vi "TLB Core Programming Tasks 1.00 (incomplete).vi"() -> ()   [LabVIEW 2018]
uses:
  TLB Type Definitions/Intruction Type Definitions.ctl
  TLB Type Definitions/State Type Definitions, for 0.26g versions and later 3.ctl
  <vilib>/Studica/Studica Toolkit/NavX/TypeDefs/Flags/Z900_navX_Flags_OpStatusTypeDef.ctl
  <vilib>/Studica/Studica Toolkit/NavX/TypeDefs/Flags/Z900_navX_Flags_CalibrationStatusTypeDef.ctl
  TLB Type Definitions/Vision cluster.ctl
  TLB Type Definitions/PING CLUSTER.ctl
  TLB Type Definitions/Encoder cluster.ctl
  TLB Type Definitions/Stepper cluster.ctl
  TLB Type Definitions/Yaw Cluster.ctl
  TLB Type Definitions/IR Sensor Type Def.ctl
  TLB Type Definitions/Line Sensor Cluster.ctl
  TLB Type Definitions/Time cluster.ctl
  TLB Type Definitions/Box Colour Detection Cluster (0.26d and above).ctl
  Underlying VI's/FGV's/Box FGV/Box Colour FGV Colours.ctl
  <vilib>/Studica/Studica Toolkit/Background/DIO Channel.ctl
  TLB Type Definitions/Y Stepper cluster.ctl
  TLB Type Definitions/Motor Speed Cluster.ctl
  Labview Training Phase 2/Enum Controls/States for Action Engine.ctl
  Underlying VI's/NavX VI/navX type def.ctl
  <vilib>/Studica/Studica Toolkit/Background/I2C Channel.ctl
  Underlying VI's/I2C Master VI/Arduino_Interfacing.ctl
  Underlying VI's/Motor Control VI with PID/MOTOR CONTROL WITH PID AE DATA MODE TYPE DEF.ctl
  Underlying VI's/Motor Control VI with PID/MOTOR CONTROL WITH PID AE DIRECTION TYPE DEF.ctl
  Experimental VI's/Archived VI's/MOTOR CONTROL NO PID Type Def.ctl
  <vilib>/myRIO/Common/Instrument Driver Framework/myRIO v1.0/AI/typedefs/AI Channels List.ctl
  <vilib>/myRIO/Common/Instrument Driver Framework/myRIO v1.0/AI/typedefs/AI Channels Enum.ctl
  Underlying VI's/Line Sensor AE/Line Sensor AE Type Def.ctl
  Underlying VI's/I2C Master VI/I2C MASTER Type Def.ctl
  Underlying VI's/Elasped Timer/Elapsed timer control.ctl
  Underlying VI's/IMAQ Create Reference AE/IMAQ Reference AE.ctl
  Underlying VI's/FGV's/Box FGV/Box Colour FGV States.ctl
  Underlying VI's/I2C Master VI/I2C_MASTER_WRITE_NEW Type Def.ctl
  Underlying VI's/Modified webcam FGV/Webcam AE.ctl
  <vilib>/userdefined/High Color/IMAQdx.ctl
  <vilib>/Studica/Studica Toolkit/NavX/NavX.lvlib
panel:
  out "Same colour?":bool
  out "Box Colour Detection":T1
  out "Errors detected":bool
  out "Robot ready":bool
  out "Time cluster":T3
  out "Table IR obstruct":bool
  out "Front IR obstruct":bool
  out "Line sensors":T4
  out "IR Sensors":T5
  out "NAVX Values":T6
  out "Stepper position values":T7
  out "Encoder values":T8
  out "Ultrasonic sensors":T9
  out "Selected Task":T10=enum."Start Task 9"
  out "Object recognition mode":enum16{"Ball", "Soap", "Gel", "Pipe", "None"}(ring)
  out "Image Processing Error":errorcluster
  out "Object Detection":T11
  out "Status":T14 {"OP Status" items=["INITIALIZING", "SELFTEST_IN_PROGRESS", "ERROR", "IMU_AUTOCAL_IN_PROGRESS", "NORMAL"]; "Calibration Status" items=["IMU_CAL_STATE_MASK"=3, "IMU_CAL_STATE_INPROGRESS"=0, "IMU_CAL_STATE_ACCUMULATE"=1, "IMU_CAL_STATE_COMPLETE"=2]}
  out "General Errors":errorcluster
  in  "Red LED":bool
  out "Front Ultrasonic obstruct":bool
  out "Speed & distance":T15
  out "Task selection":u8
  out "NavX Readings":T16
  out "Arduino Data":T17
  out "TASK ENABLE":bool
  out "Rising Edge":bool
  in  "Green LED":bool
  out "State Logic":T18=enum."Startup"
  out "elements":T10[](array[typedef])
  in  "STOP TASK":bool
  in  "OK Button":bool
  in  "STOP":bool
  out "Queue Errors":errorcluster
  out "Action Queue Items":i32
  out "State Logic Queue Items":i32
  out "Action Queues items":string[](array[string])=["Hardware reset", "Software reset", ""]
  out "Action State":string
  # "VISION"
  # "TLB FRAMEWORK STATUS"
  # "System Health Status Update"
  # "Test Programme written by Calvin Loke    Dated: 28 Aug 2019\nTest Programme revised by Dr Alex See   Dated 30 Aug 2019\n\nRevision date: 20/03/2020\nProgramme version:   TLB Native Dynamic Events ver 0.19a"
  # "0: Task 1\n1: Task 2\n2: Task 3\n3: Task 4\n4: Task 5\n5: Task 6\n6: Task 7\n7: Task 8 Ball\n8: Task 8 Soap\n9: Task 8 Gel\n10: Task 8 Pipe\n11: Task 9 Blue\n12: Task 9 Black\n13: Task 9 Green\n14: Task 9 Red\n15: Task 9 Yellow"
  # "Ball: Right\nSoap: Left\nGel: Reverse\nPipe: Forward"
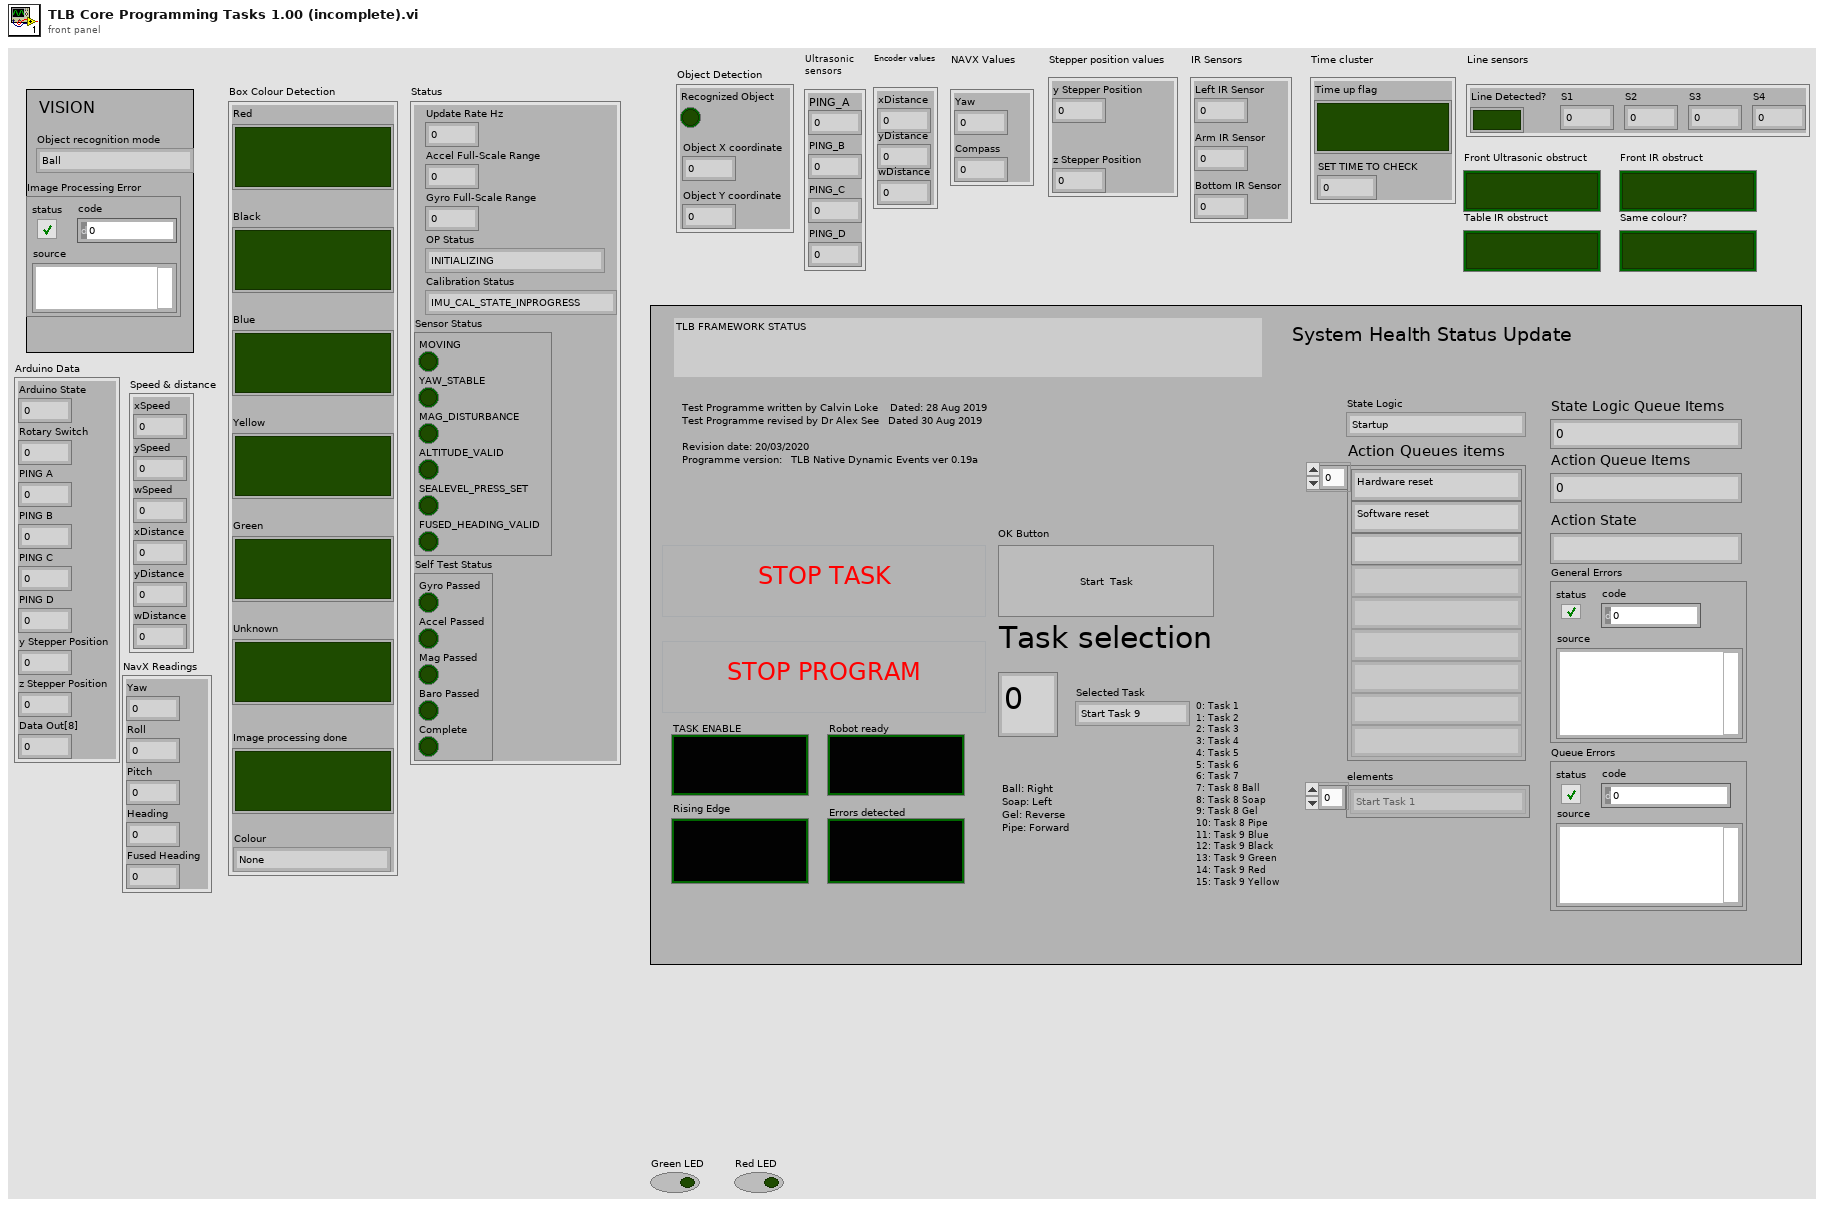
[diagram p1: front panel]
types:
  T1 = typedef "Box Colour Detection Cluster (0.26d and above).ctl" = cluster{"Red":bool, "Black":bool, "Blue":bool, "Yellow":bool, "Green":bool, "Unknown":bool, "Image processing done":bool, "Colour":T2}
  T2 = typedef "Box Colour FGV Colours.ctl" = enum16{"None", "Black", "Blue", "Green", "Red", "Yellow"}
  T3 = typedef "Time cluster.ctl" = cluster{"Time up flag":bool, "SET TIME TO CHECK":dbl}
  T4 = typedef "Line Sensor Cluster.ctl" = cluster{"Line Detected?":bool, "S1":dbl, "S2":dbl, "S3":dbl, "S4":dbl}
  T5 = typedef "IR Sensor Type Def.ctl" = cluster{"Left IR Sensor":dbl, "Arm IR Sensor":dbl, "Bottom IR Sensor":dbl}
  T6 = typedef "Yaw Cluster.ctl" = cluster{"Yaw":dbl, "Compass":dbl}
  T7 = typedef "Stepper cluster.ctl" = cluster{"y Stepper Position":u8, "z Stepper Position":u8}
  T8 = typedef "Encoder cluster.ctl" = cluster{"xDistance":dbl, "yDistance":dbl, "wDistance":dbl}
  T9 = typedef "PING CLUSTER.ctl" = cluster{"PING_A":u8, "PING_B":u8, "PING_C":u8, "PING_D":u8}
  T10 = typedef "Intruction Type Definitions.ctl" = enum16{"None", "Start Task 1", "Start Task 2", "Start Task 3", "Start Task 4", "Start Task 5", "Start Task 6", "Start Task 7", "Start Task 8 - BALL", "Start Task 8 - Gel", "Start Task 8 - Pipe", "Start Task 8 - Soap", "Start Task 9", "Start Task A", "Start Task B", "Exit"}
  T11 = typedef "Vision cluster.ctl" = cluster{"Recognized Object":bool, "Object X coordinate":dbl, "Object Y coordinate":dbl}
  T12 = typedef "NavX.lvlib/Z900_navX_Flags_OpStatusTypeDef.ctl" = u8
  T13 = typedef "NavX.lvlib/Z900_navX_Flags_CalibrationStatusTypeDef.ctl" = u8
  T14 = cluster{"Update Rate Hz":u8, "Accel Full-Scale Range":u8, "Gyro Full-Scale Range":u16, "OP Status":T12, "Calibration Status":T13, "Sensor Status":cluster{"MOVING":bool, "YAW_STABLE":bool, "MAG_DISTURBANCE":bool, "ALTITUDE_VALID":bool, "SEALEVEL_PRESS_SET":bool, "FUSED_HEADING_VALID":bool}, "Self Test Status":cluster{"Gyro Passed":bool, "Accel Passed":bool, "Mag Passed":bool, "Baro Passed":bool, "Complete":bool}}
  T15 = cluster{"xSpeed":dbl, "ySpeed":dbl, "wSpeed":dbl, "xDistance":dbl, "yDistance":dbl, "wDistance":dbl}
  T16 = cluster{"Yaw":dbl, "Roll":dbl, "Pitch":dbl, "Heading":dbl, "Fused Heading":dbl}
  T17 = cluster{"Arduino State":u8, "Rotary Switch":u8, "PING A":u8, "PING B":u8, "PING C":u8, "PING D":u8, "y Stepper Position":u8, "z Stepper Position":u8, "Data Out[8]":u8}
  T18 = typedef "State Type Definitions, for 0.26g versions and later 3.ctl" = enum16{"None", "Startup", "Move to Angle", "True Stop", "Idle", "Shutdown", "Task 1A", "Task 1B", "Task 2:Raise Arm", "Task 2:Sensor Mode", "Task 2:Reverse Mode", "Task 3", "Task 4_A", "Task 4_B", "Task 4_C", "Task 4_D", "Task 5A: RAISING ARM", "Task 5B: STILL WAITING", "Task 5C: GOING DOWN", "Task 5D: GRAB", "Task 5E: GOING UP", "Task 5F: ARM GRAB HEIGHT", "Task 5G: CLOSE CLAW", "Task 5H: RAISE ARM", "Task 6A: RAISE ARM", "Task 6B: CAM BURST", "Task 6C: PROCESS IMAGE", "Task 6D: BALL BUSTER", "Task 6E: STILL WAITING", "Task 6F: CAM BURST 2", "Task 6G: PROCESS IMAGE 2", "Task 6H: SKADI SOAPS", "Task 6I: STILL WAITING 2", "Task 6J: CAM BURST 3", "Task 6K: PROCESS IMAGE 3", "Task 6L: JAM IT IN", "Task 6M: STILL WAITING 3", "Task 6N: CAM BURST 4", "Task 6O: PROCESS IMAGE 4", "Task 6P: PIPE BOMB", "Task 7", "Task 8A: RAISE ARM", "Task 8B: MOVE TO BOX", "Task 8C: CAM BURST", "Task 8D: PROCESS IMAGE", "Task 8E: ROBOT ADJUST", "Task 8F: CAM BURST 2", "Task 8G: PROCESS IMAGE 2", "Task 8H: ARM ADJUST", "Task 8I: ARM GRAB HEIGHT", "Task 8J: CLOSE CLAW", "Task 8K: RAISE MY SWORD", "Task 8I: STILL WAITING", "Task 8L: Return to position", "Task 9A: Raise Arm", "Task 9B: Rotate to Angle", "Task 9C: Detect Box", "Task 9D: MOVE FORWARD", "Task 9E: MOVE LEFT", "Task 9E2: MOVE RIGHT", "Task 9F: SCAN BOX", "Task 9G: MOVE RIGHT", "Task 9H: SCAN BOX 2", "Task 9I: ROTATE 90 CW", "Task 9J: FORWARD", "Task 9K: RAM WALL", "Task 9L: MOVE RIGHT", "Task 9M: SCAN BOX 3", "Task 9N: MOVE RIGHT", "Task 9O: SCAN BOX 4", "Task A1: RAISE ARM", "Task A2: ROTATE TO ANGLE", "Task A3: MOVE TO BL BOX", "Task A4: MOVE FORWARD", "Task A5: ROTATE CW 90"}
  T19 = typedef "Motor Speed Cluster.ctl" = cluster{"ySpeed":dbl, "xSpeed":dbl, "wSpeed":dbl}
  T20 = typedef "Y Stepper cluster.ctl" = cluster{"yStepper desired":u8}
  T21 = typedef "DIO Channel.ctl" = enum16{"Not Connected", "A/DIO1", "A/DIO2", "A/DIO3", "A/DIO4", "A/DIO5", "A/DIO6", "A/DIO7", "A/DIO13", "B/DIO1", "B/DIO2", "B/DIO3", "B/DIO4", "B/DIO5", "B/DIO6", "B/DIO7", "B/DIO13", "C/DIO0", "C/DIO1", "C/DIO2", "C/DIO3", "C/DIO4", "C/DIO5", "C/DIO6", "C/DIO7"}
  T22 = cluster{"DIO Channel":T21, "FPGA VI Reference Out":refnum<k20>}
  T23 = typedef "States for Action Engine.ctl" = enum16{"Initialize", "Write", "Read"}
  T24 = typedef "MOTOR CONTROL WITH PID AE DATA MODE TYPE DEF.ctl" = enum16{"Init AE", "Write to AE", "Read from AE"}
  T25 = typedef "navX type def.ctl" = enum16{"Get i2C reference", "Read Values", "Zero Yaw"}
  T26 = typedef "Arduino_Interfacing.ctl" = enum16{"Initialize", "Write to Arduino", "Read From Arduino"}
  T27 = typedef "I2C Channel.ctl" = enum16{"Not Connected", "A", "B"}
  T28 = cluster{"I2C Ref Out":cluster{"I2C Channel":T27, "FPGA VI Reference Out":refnum<k20>}, "Connected":bool, "Slave Address (7-bit)":u8, "Registry":u8[]}
  T29 = typedef "Box Colour FGV States.ctl" = enum16{"Initialize", "Read", "Write"}
  T30 = typedef "MOTOR CONTROL WITH PID AE DIRECTION TYPE DEF.ctl" = enum16{"y-axis movement", "x-axis movement", "rotation", "stop", "reset encoders"}
  T31 = typedef "Line Sensor AE Type Def.ctl" = enum16{"INIT AE", "READ FROM LINE SENSORS"}
  T32 = typedef "IMAQ Reference AE.ctl" = enum16{"Initialize AE", "Get IMAQ Reference", "Dispose Processing Buffer"}
  T33 = typedef "Elapsed timer control.ctl" = enum16{"Start", "Pause", "Initialize"}
  T34 = typedef "I2C_MASTER_WRITE_NEW Type Def.ctl" = enum16{"Ultrasonic sensors", "Stepper origin", "zStepper 13.3k", "zStepper 13k", "zStepper 12k", "zStepper 11k", "zStepper 10k", "zStepper 9k", "zStepper 8k", "zStepper 7k", "zStepper 6k", "zStepper 5k", "zStepper 4k", "zStepper 3k", "zStepper 2k", "zStepper 1k", "zStepper 900", "zStepper 800", "zStepper 700", "zStepper 600", "zStepper 500", "zStepper 400", "zStepper 300", "zStepper 200", "zStepper 100", "zStepper 0", "yStepper control", "Open Claw", "Close Claw", "Soft Reset"}
  T35 = typedef "Webcam AE.ctl" = enum16{"Initialize Camera", "Open Camera", "Continuous Acquisition", "Close Camera", "Retrieve Image", "Dispose Camera Image Buffer"}
  T36 = typedef "IMAQdx.ctl" = refnum<k21>
  T37 = typedef "MOTOR CONTROL NO PID Type Def.ctl" = enum16{"Init", "Front Back", "Left Right", "Rotate", "Stop", "Latch"}
  T38 = typedef "AI Channels List.ctl" = T39[]
  T39 = typedef "AI Channels Enum.ctl" = enum16{"Not Connected", "AudioIn/Left", "AudioIn/Right", "C/AI0", "C/AI1", "A/AI0", "A/AI1", "A/AI2", "A/AI3", "A/AI4", "A/AI5", "A/AI6", "A/AI7", "B/AI0", "B/AI1", "B/AI2", "B/AI3", "B/AI4", "B/AI5", "B/AI6", "B/AI7", "AI/AI0", "AI/AI1", "AI/AI2", "AI/AI3", "A/AI0 (DIFF)", "A/AI1 (DIFF)", "A/AI2 (DIFF)", "A/AI3 (DIFF)", "B/AI0 (DIFF)", "B/AI1 (DIFF)", "B/AI2 (DIFF)", "B/AI3 (DIFF)"}
  T40 = cluster{"S1":dbl, "S2":dbl, "S3":dbl, "S4":dbl, "Array[4]":dbl, "Array[5]":dbl, "Array[6]":dbl, "Array[7]":dbl, "Array[8]":dbl}
  T41 = typedef "I2C MASTER Type Def.ctl" = enum16{"Last State", "Mode 0", "Mode 1", "Mode 2", "Mode 3", "Mode 4", "Mode 5", "Mode 6", "Mode 7", "Mode 8", "Mode 9", "Mode 10"}
  T42 = typedef "IMAQ Image.ctl" = refnum<image>
  T43 = cluster{"Number of Matches":i32, "Object detected?":bool}
  T44 = cluster{"Red":bool, "Black":bool, "Blue":bool, "Yellow":bool, "Green":bool, "No recognizable coolour":bool}
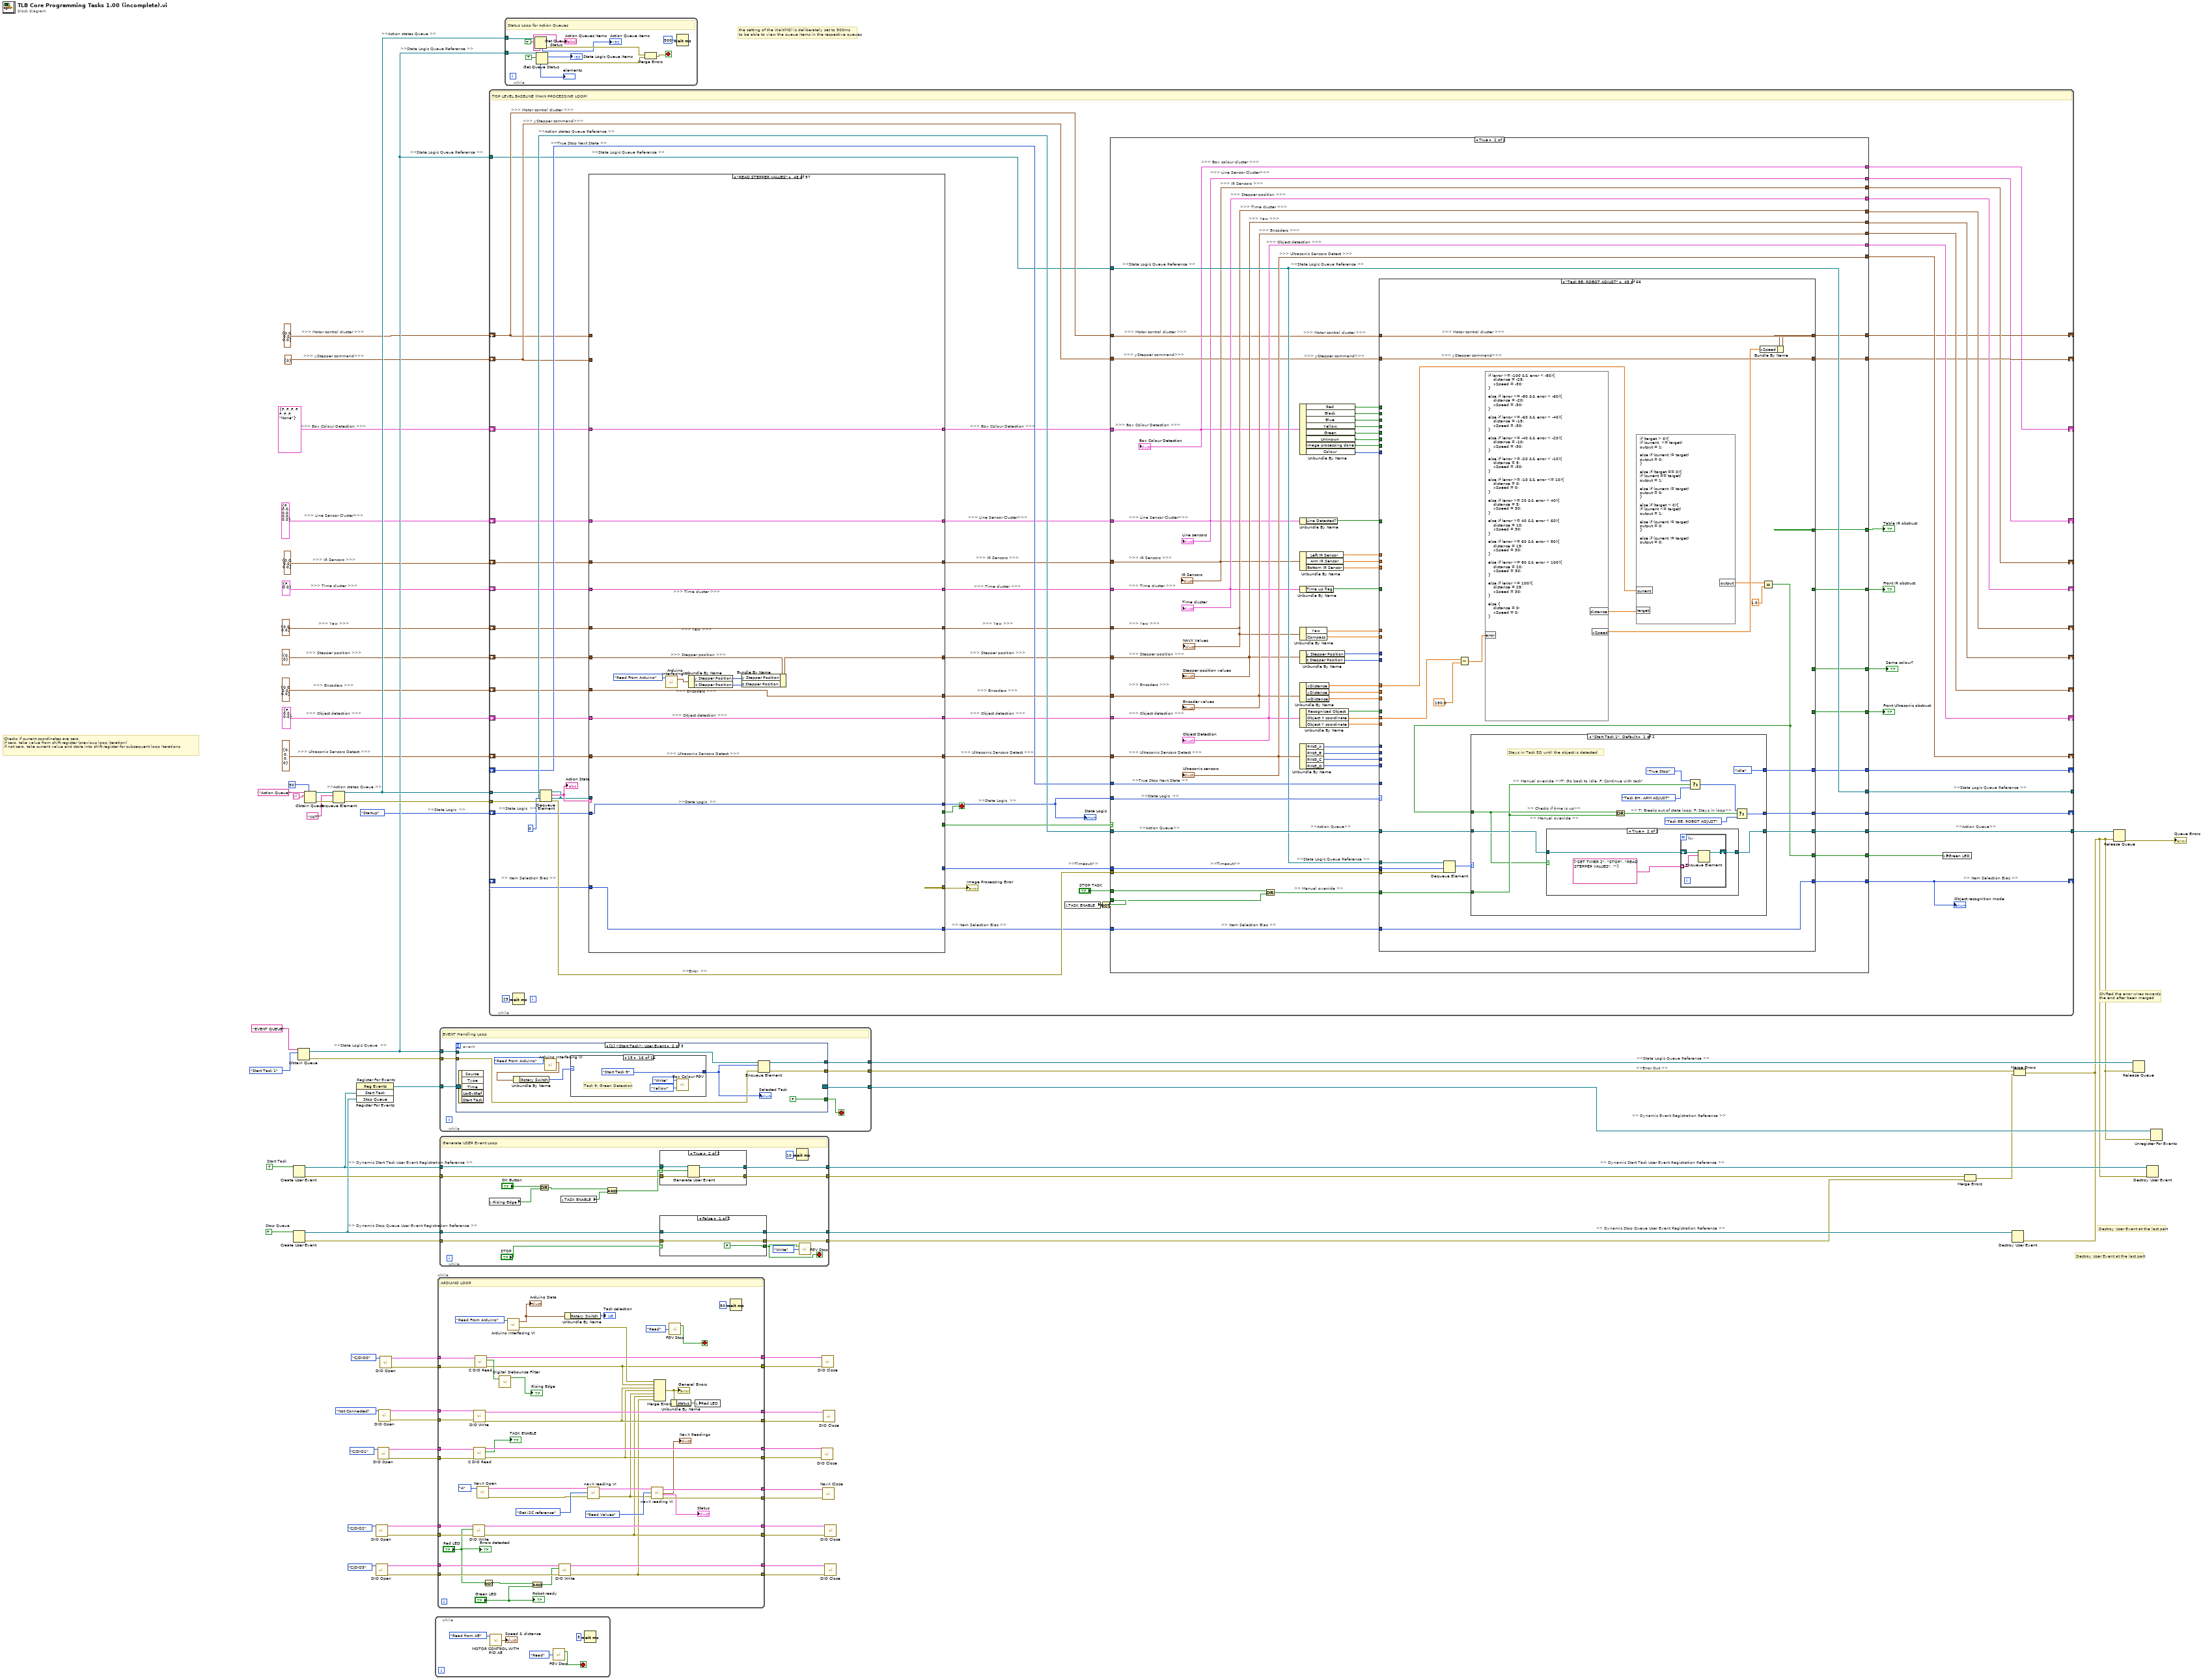
[diagram p0: block diagram]
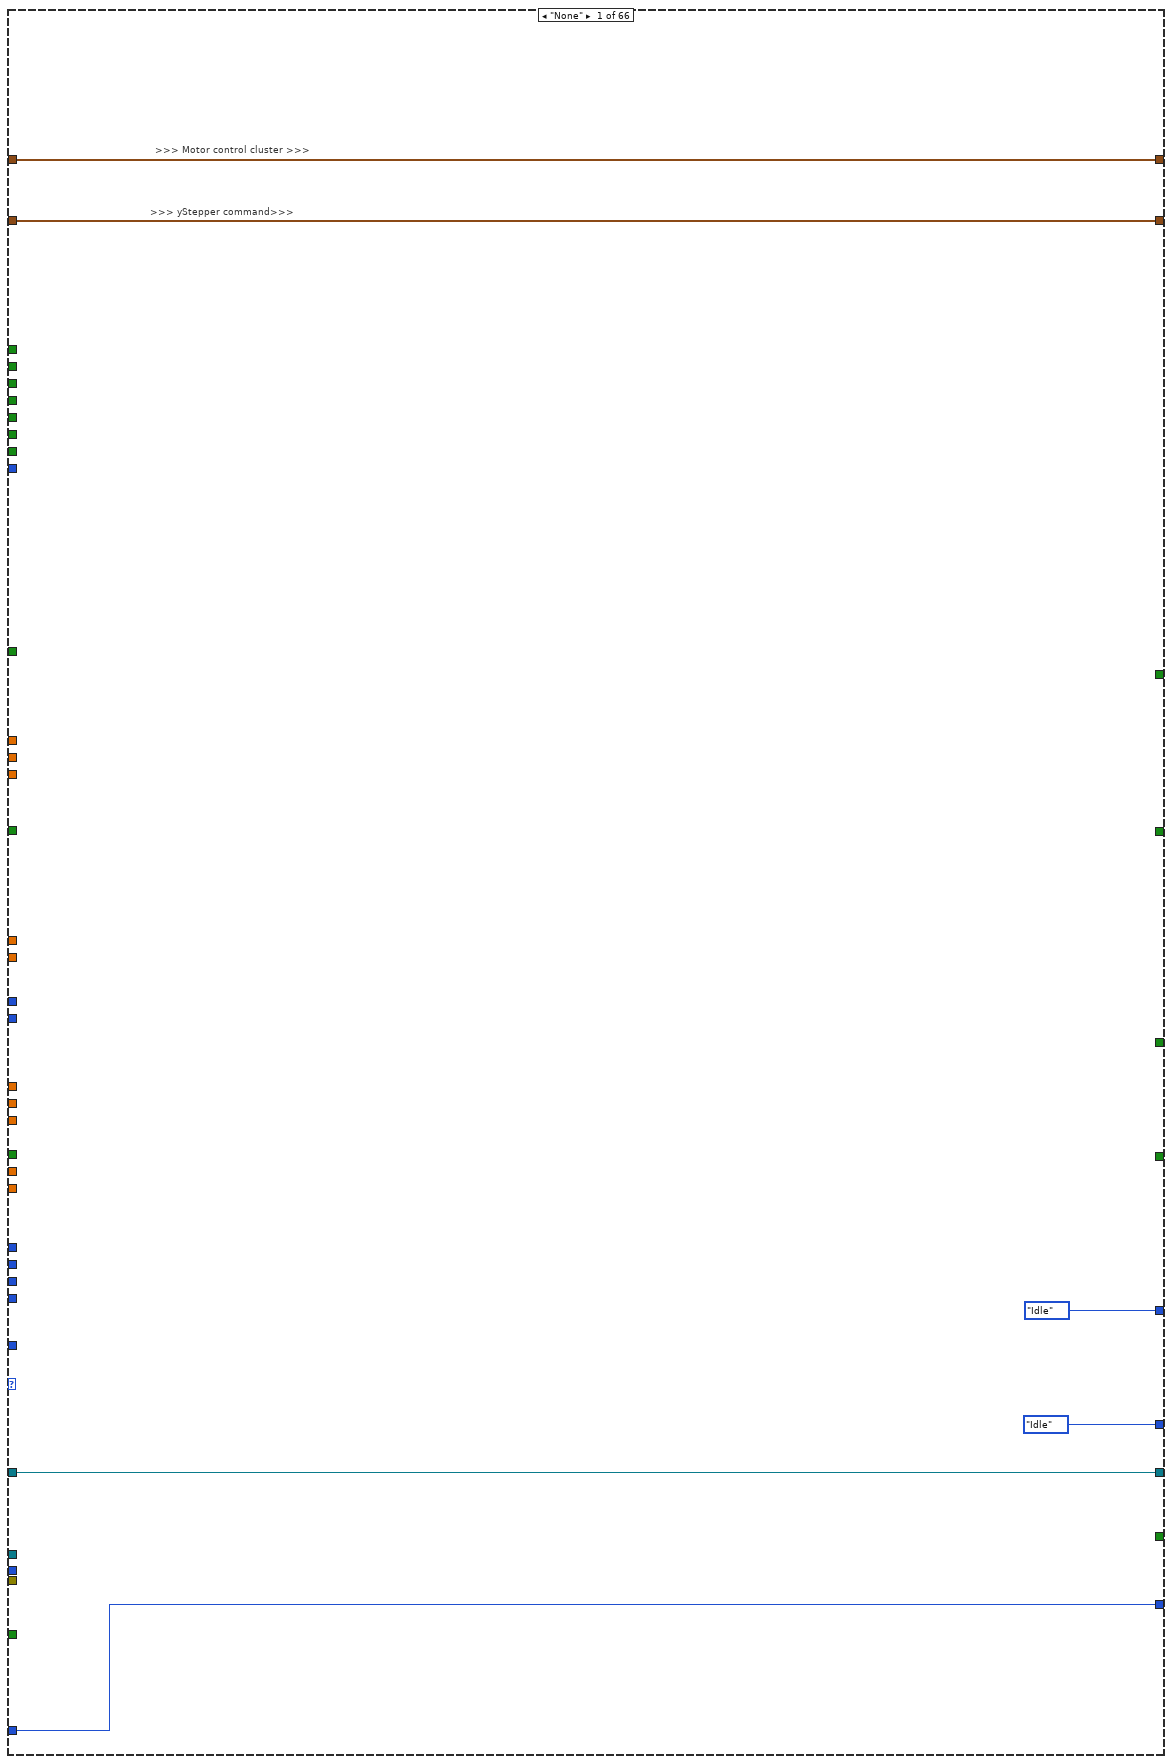
[diagram p3: hidden frame]
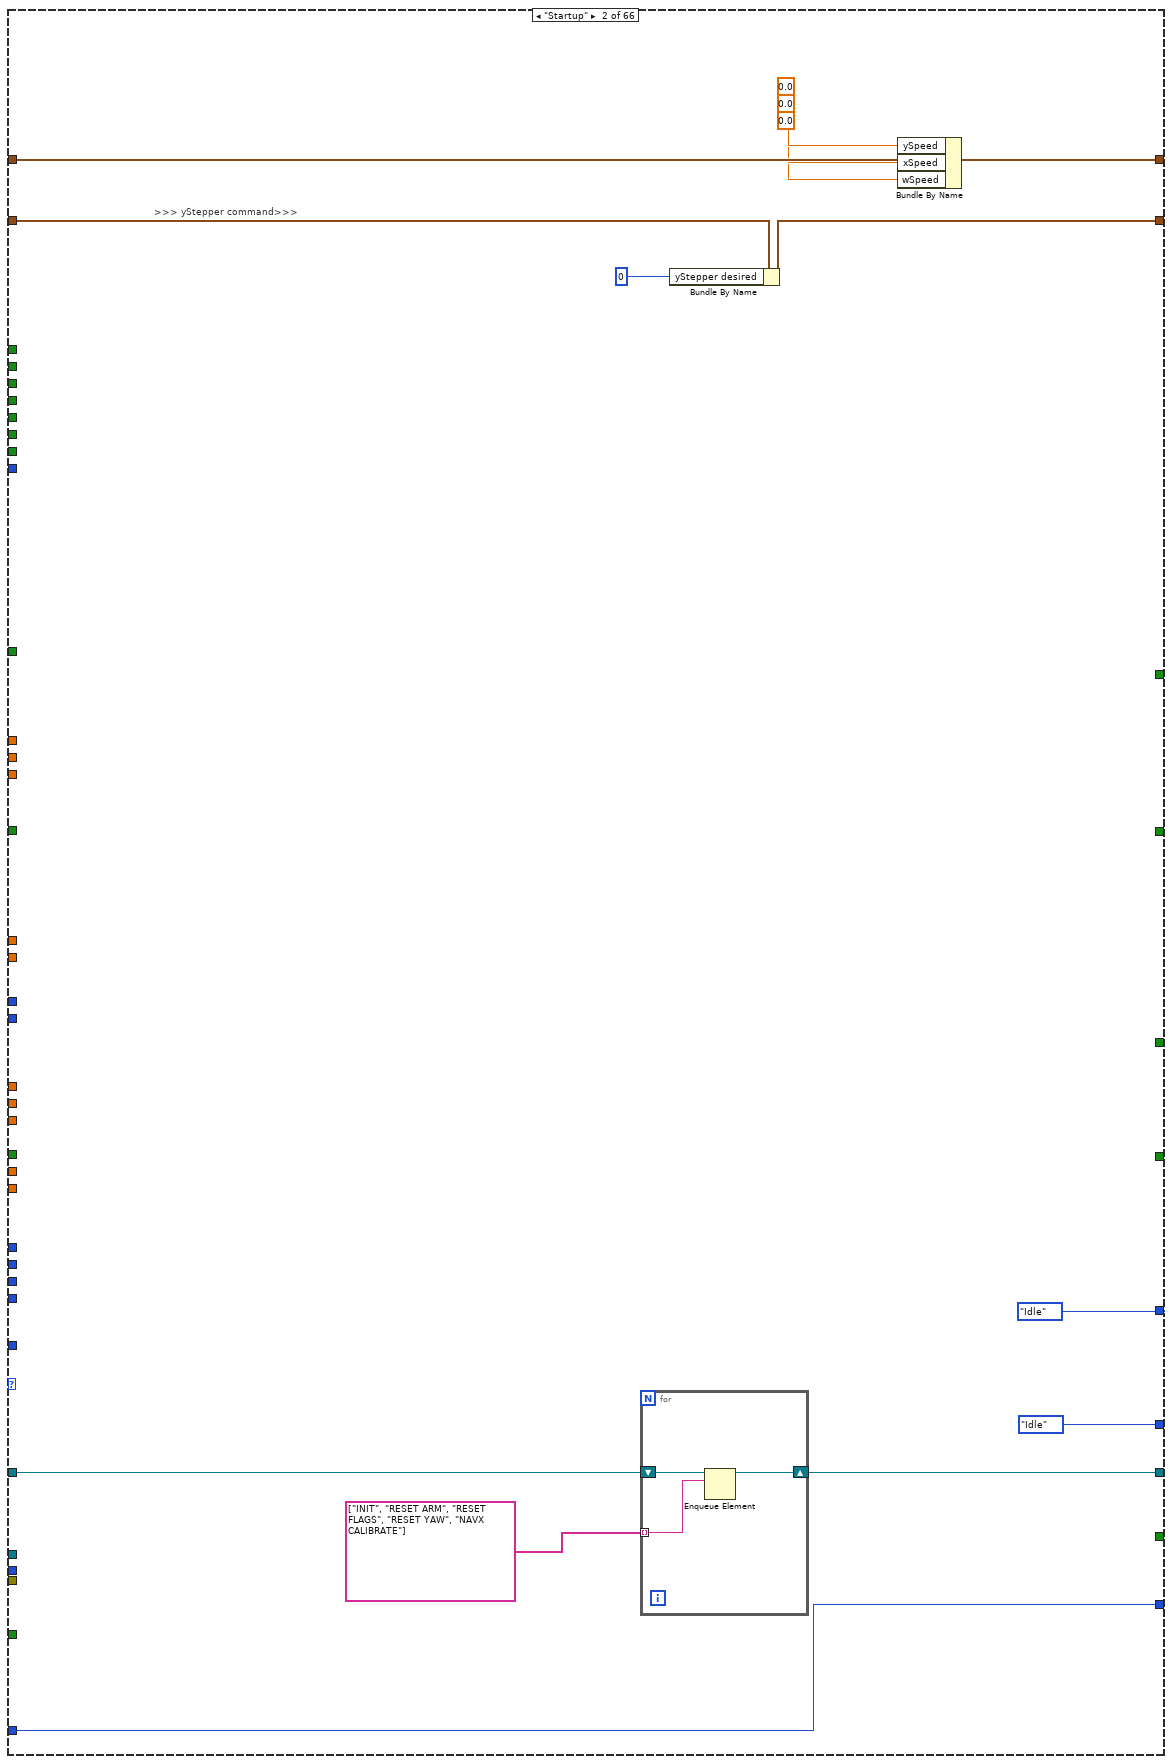
[diagram p4: hidden frame]
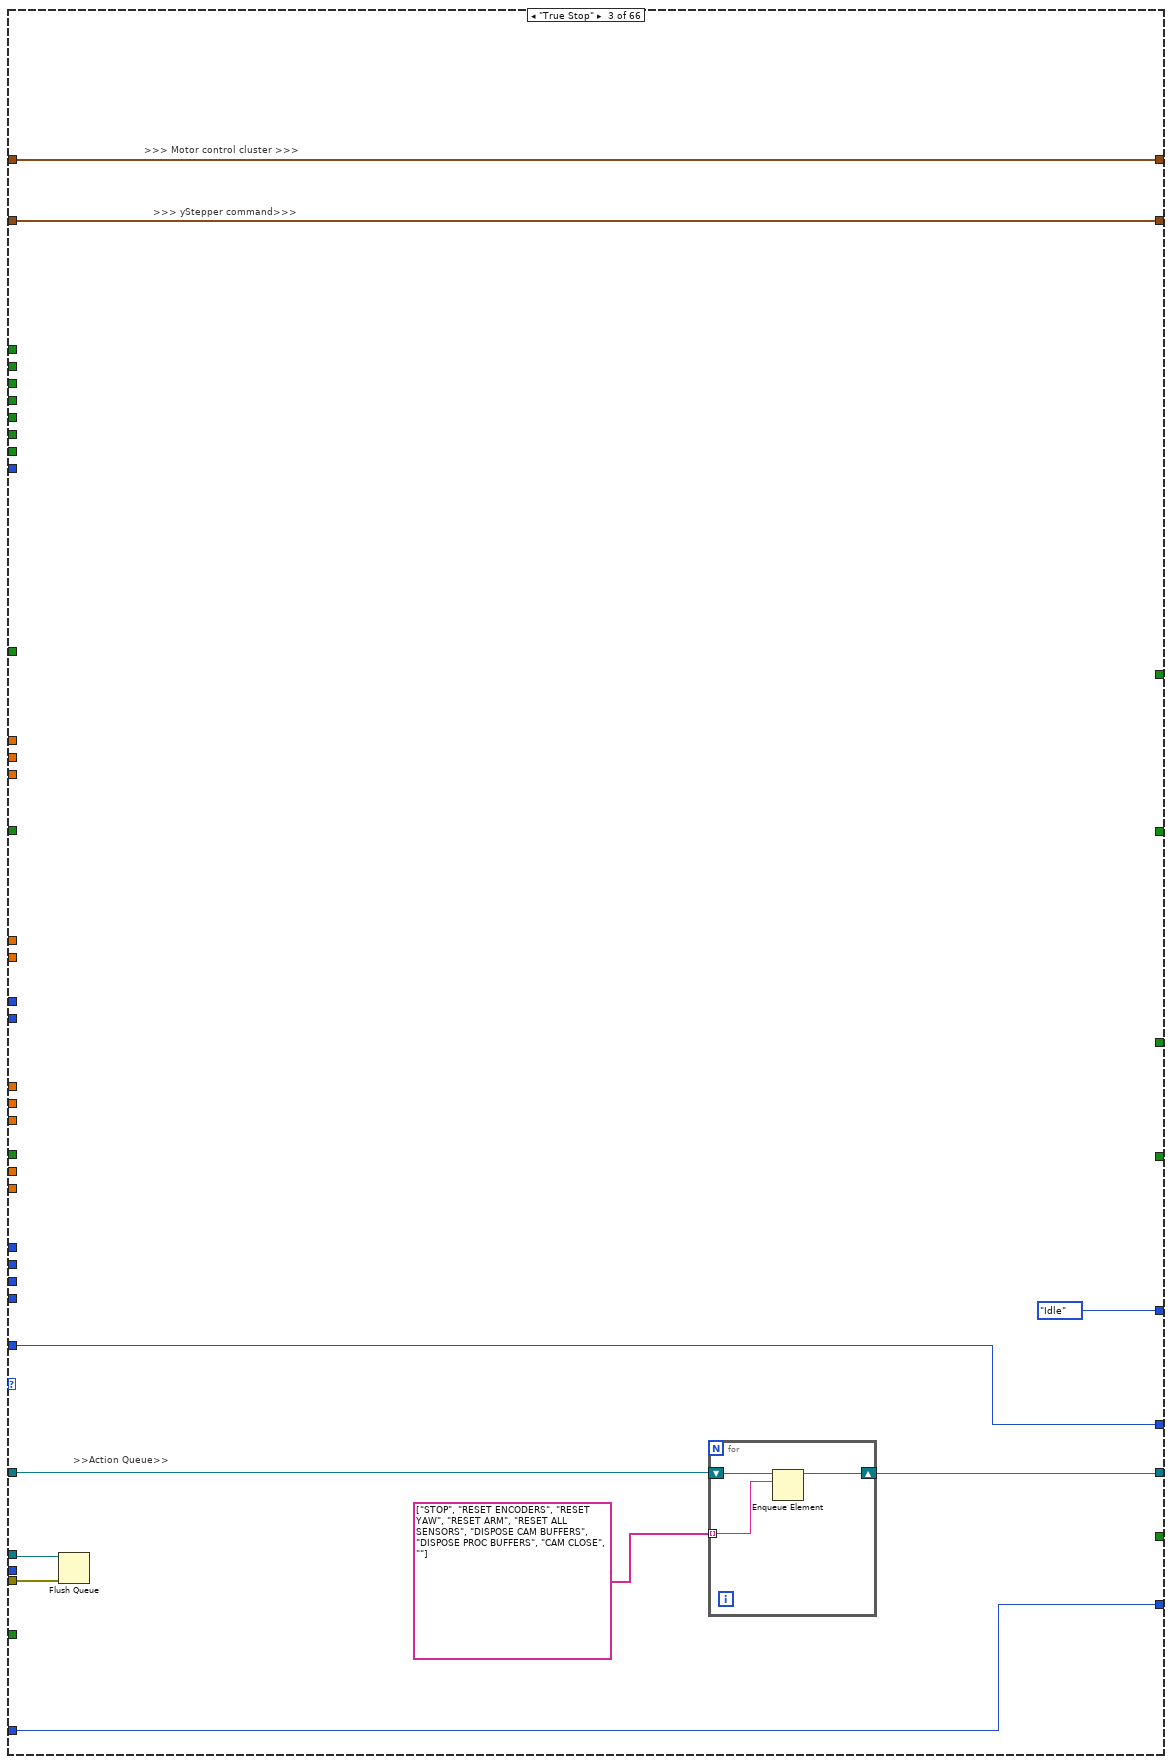
[diagram p5: hidden frame]
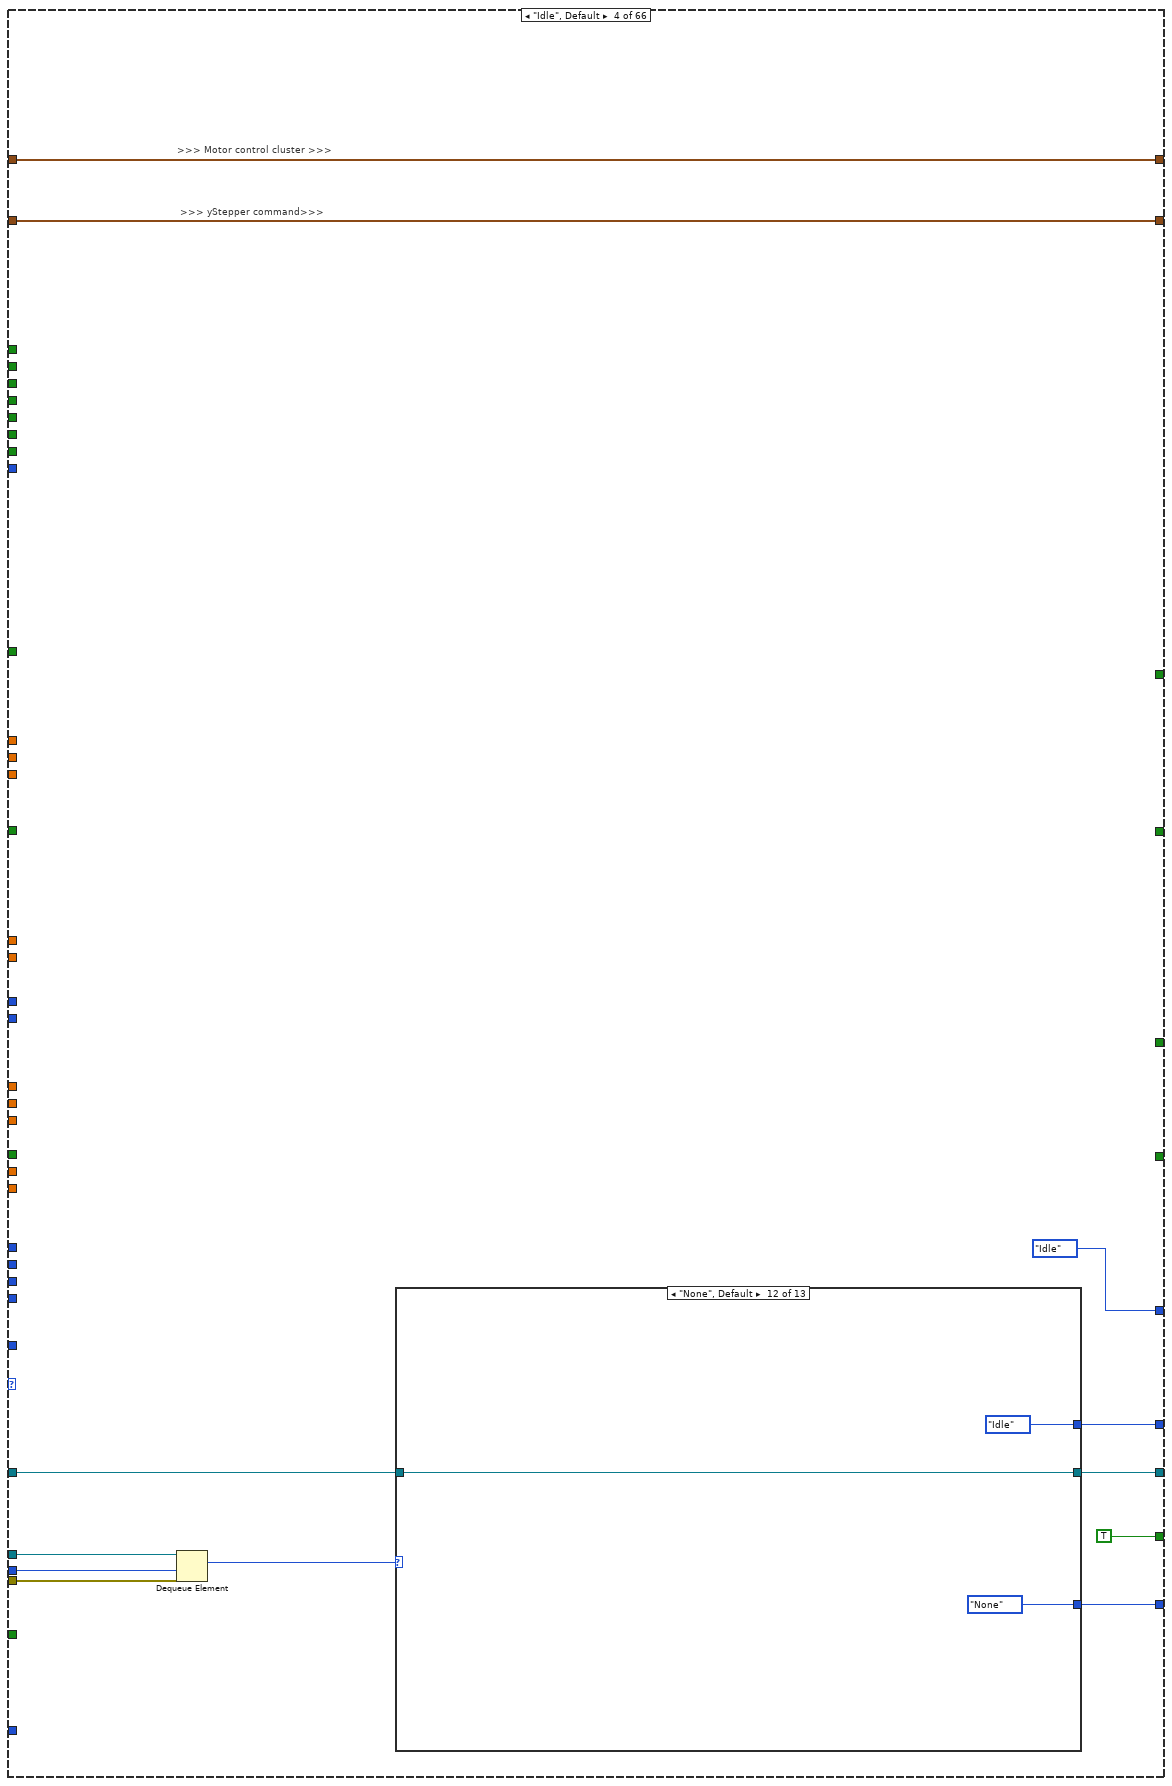
[diagram p6: hidden frame]
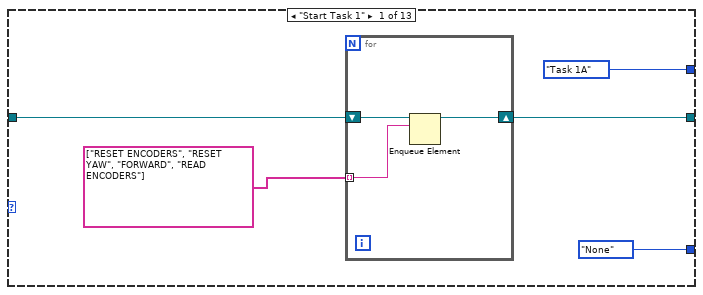
[diagram p7: hidden frame]
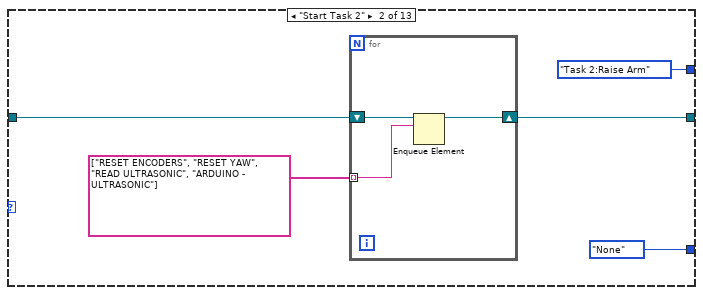
[diagram p8: hidden frame]
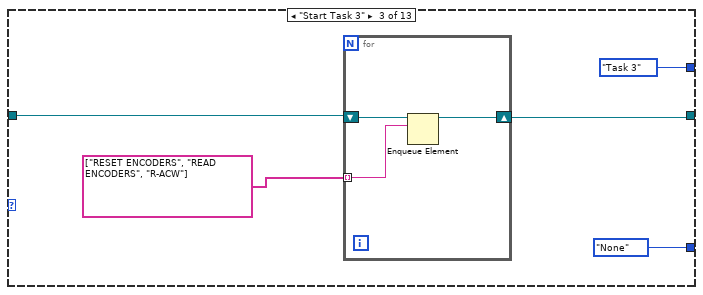
[diagram p9: hidden frame]
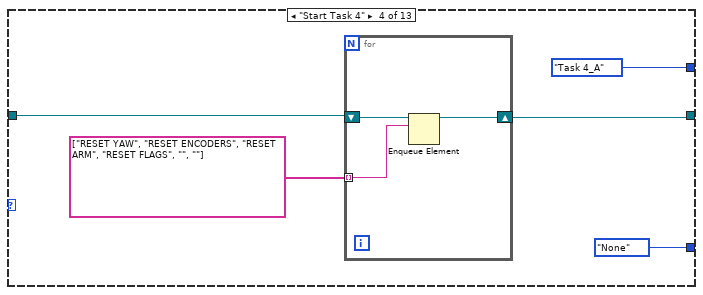
[diagram p10: hidden frame]
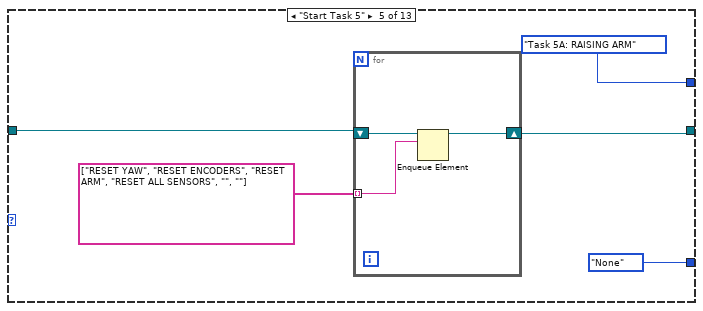
[diagram p11: hidden frame]
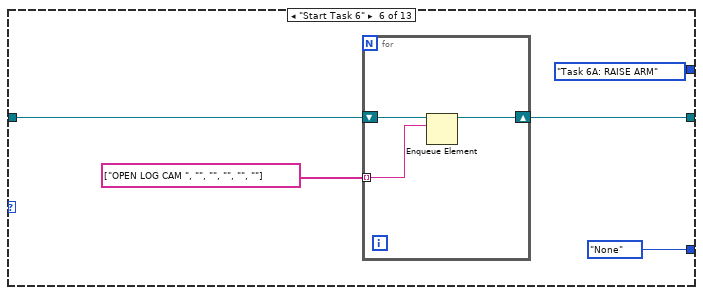
[diagram p12: hidden frame]
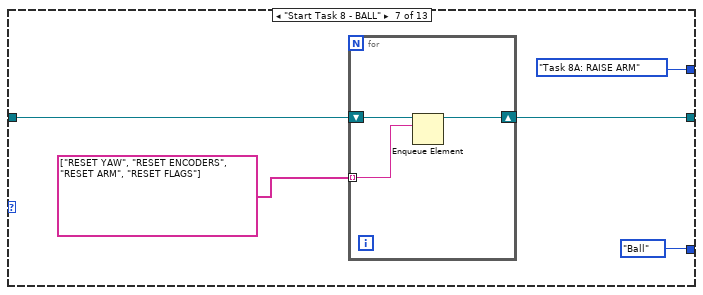
[diagram p13: hidden frame]
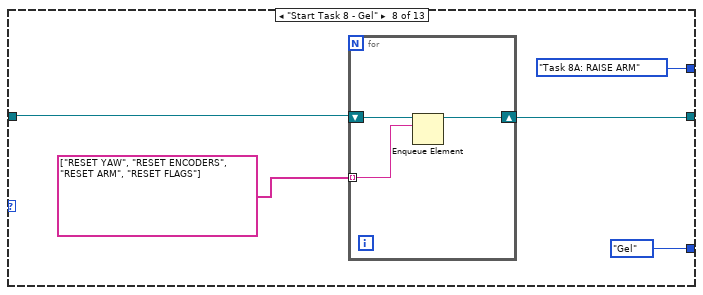
[diagram p14: hidden frame]
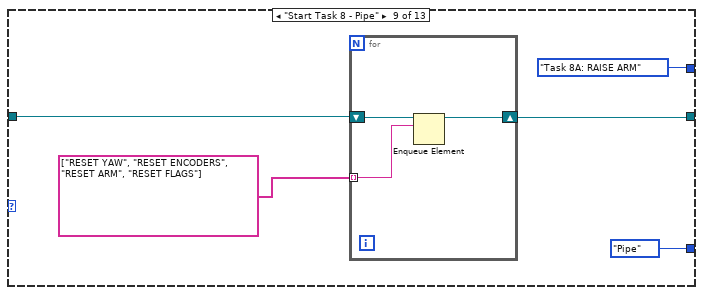
[diagram p15: hidden frame]
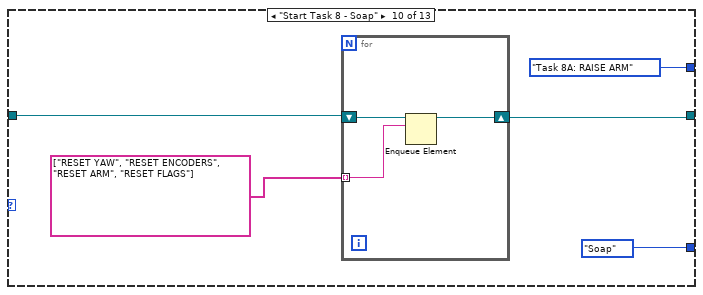
[diagram p16: hidden frame]
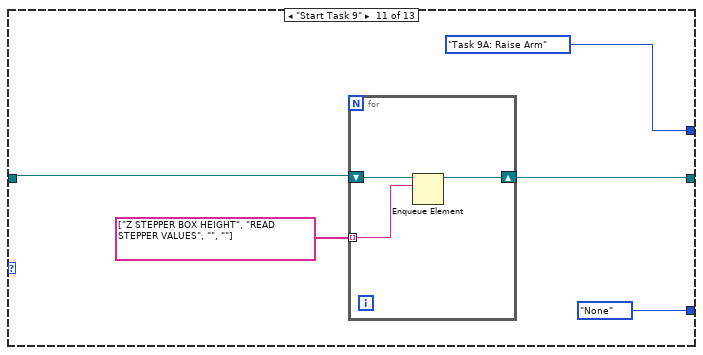
[diagram p17: hidden frame]
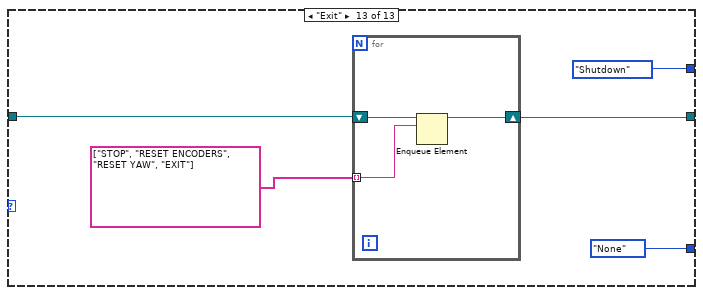
[diagram p18: hidden frame]
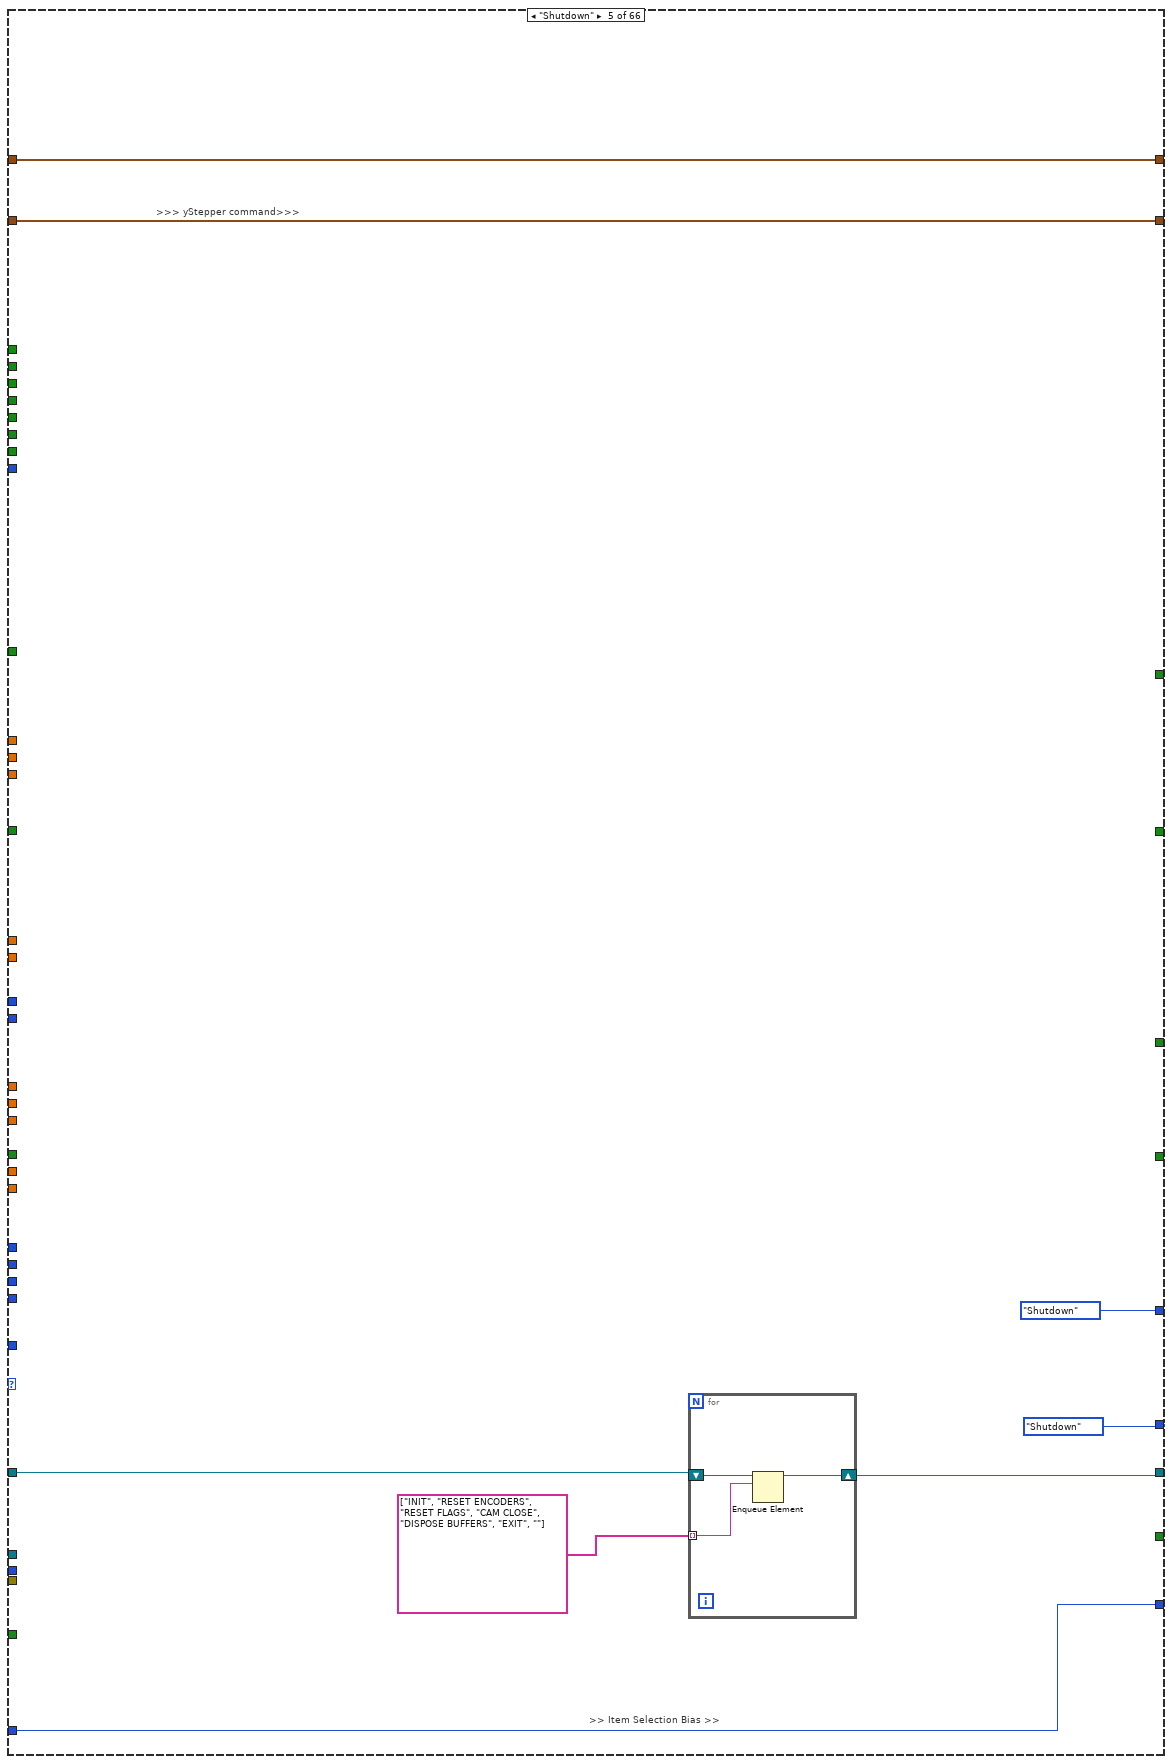
[diagram p19: hidden frame]
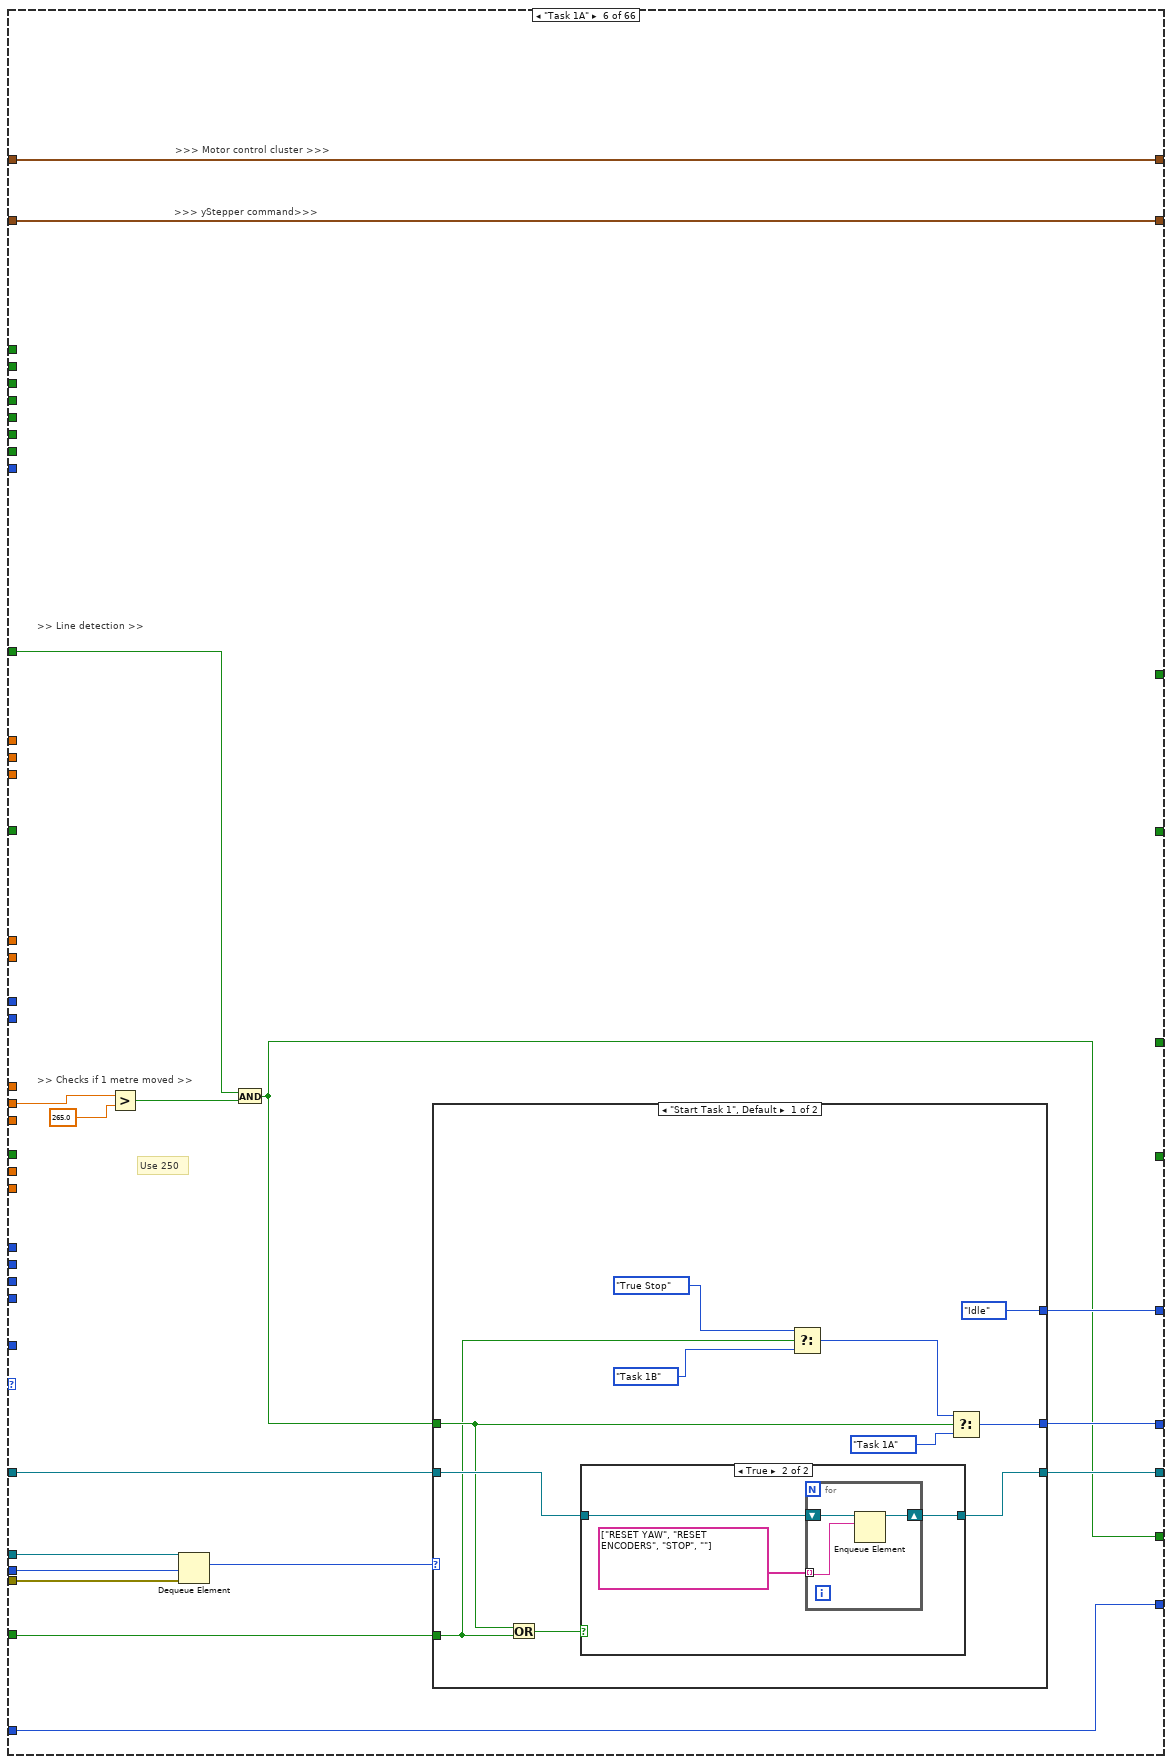
[diagram p20: hidden frame]
diagram:
  w69 = TRUE  # Stop Queue
  w68 = TRUE  # Start Task
  # ">>State Logic Queue Reference >>"
  # ">>Action states Queue >>"
  # ">>> Box Colour Detection >>>"
  # ">>State Logic Queue Reference >>"
  # ">>State Logic  >>"
  # ">>> Line Sensor Cluster>>>"
  # ">>> Motor control cluster >>>"
  # ">>> IR Sensors >>>"
  # "Checks if current coordinates are zero\nif zero, take value from shift register (previous loop iteration)\nif not zero, take current value and store into shift register for subsequent loop iterations"
  # ">>> yStepper command>>>"
  # ">>> Time cluster >>>"
  # ">>> Yaw >>>"
  # ">>> Stepper position >>>"
  # ">>> Encoders >>>"
  # ">>> Object detection >>>"
  # ">>> Ultrasonic Sensors Detect >>>"
  # "the setting of the Wait(MS) is deliberately set to 500ms\nto be able to view the queue items in the respective queues"
  # ">>Error Out >>"
  # ">> Dynamic Stop Queue User Event Registration Reference >>"
  # ">> Dynamic Start Task User Event Registration Reference >>"
  # ">> Dynamic Stop Queue User Event Registration Reference >>"
  # ">> Dynamic Start Task User Event Registration Reference >>"
  # ">> Dynamic Event Registration Reference >>"
  # ">>Action states Queue >>"
  # ">>State Logic Queue  >>"
  # ">>State Logic Queue Reference >>"
  # "Destroy User Event at the last part"
  # "Destroy User Event at the last part"
  # "Shifted the error wires towards\nthe end after been merged"
  n1 = Create User Event(user event datatype=w68) -> (user event=w60:refnum<user-event>, error out=w65:errorcluster)  [unwired: 1 in]
  n2 = Create User Event(user event datatype=w69) -> (user event=w61:refnum<user-event>, error out=w64:errorcluster)  [unwired: 1 in]
  n3 = Obtain Queue(name (unnamed)="EVENT QUEUE", element data type=Intruction_Type_Definitions."Start Task 1" ("Enum")) -> (queue out=w46:refnum<queue>, error out=w52:errorcluster)  [unwired: 3 in, 1 out]
  n4 = Obtain Queue(max queue size (-1, unlimited)=50, name (unnamed)="Action Queue", element data type="") -> (queue out=w55:refnum<queue>, error out=w51:errorcluster)  [unwired: 2 in, 1 out]
  n5 = Enqueue Element(queue=w55, element="INIT", error in (no error)=w51) -> (queue out=w47:refnum<queue>, error out=w50:errorcluster)  [unwired: 1 in, 1 out]
  n6 = register-events "Register For Events"(w60, w61) -> (reference out=w59:refnum<event-registration>)  [unwired: 2 in, 1 out]
  n7 = call <vilib>:"DIO Open.vi"("DIO Channel"=DIO_Channel."C/DIO2") -> ("error out"=w19:errorcluster, "DIO Info Out"=w20:T22)  [unwired: 9 in]
  n8 = call <vilib>:"DIO Open.vi"("DIO Channel"=DIO_Channel."C/DIO3") -> ("error out"=w14:errorcluster, "DIO Info Out"=w15:T22)  [unwired: 9 in]
  n9 = call <vilib>:"DIO Open.vi"("DIO Channel"=DIO_Channel."C/DIO1") -> ("error out"=w24:errorcluster, "DIO Info Out"=w25:T22)  [unwired: 9 in]
  n10 = call <vilib>:"DIO Open.vi"("DIO Channel"=DIO_Channel."Not Connected") -> ("error out"=w29:errorcluster, "DIO Info Out"=w31:T22)  [unwired: 9 in]
  n11 = call <vilib>:"DIO Open.vi"("DIO Channel"=DIO_Channel."C/DIO0") -> ("error out"=w34:errorcluster, "DIO Info Out"=w37:T22)  [unwired: 9 in]
  n12 = while {
    stop <- w71 stop-if-true
    n13 = call "MOTOR CONTROL WITH PID AE.vi"("AE Mode"=MOTOR_CONTROL_WITH_PID_AE_DATA_MODE_TYPE_DEF."Read from AE") -> ("Speed & distance"=→"Speed & distance":T15)  [unwired: 3 in]
    n14 = call "FGV Stop.vi"("Init/Read/Write State"=States_for_Action_Engine."Read") -> ("Output node"=w71:bool)  [unwired: 2 in, 1 out]
    n15 = Wait (ms)(milliseconds to wait=u32 5) -> ()  [unwired: 1 out]
  }
  n16 = while {
    tunnel: w37 -> [w118]
    tunnel: [w117] -> w35
    tunnel: w34 -> [w116]
    tunnel: [w87] -> w33
    tunnel: w31 -> [w113]
    tunnel: [w112] -> w30
    tunnel: w29 -> [w111]
    tunnel: [w86] -> w28
    tunnel: [w110] -> w26
    tunnel: w25 -> [w109]
    tunnel: w24 -> [w108]
    tunnel: [w85] -> w23
    tunnel: w20 -> [w102]
    tunnel: w19 -> [w101]
    tunnel: [w100] -> w18
    tunnel: [w83] -> w17
    tunnel: w15 -> [w99]
    tunnel: w14 -> [w98]
    tunnel: [w97] -> w13
    tunnel: [w82] -> w12
    tunnel: [w94] -> w9
    tunnel: [w93] -> w10
    stop <- w120 stop-if-true
    # "ARDUINO LOOP"
    n17 = call <vilib>:"DIO Write.vi"("error in (no error)"=w101, "Input"="Red LED", "DIO Info In"=w102) -> ("error out"=w83:errorcluster, "DIO Info Out"=w100:T22)  [unwired: 7 in]
    n18 = call <vilib>:"DIO Write.vi"("error in (no error)"=w111, "DIO Info In"=w113) -> ("error out"=w86:errorcluster, "DIO Info Out"=w112:T22)  [unwired: 8 in]
    n19 = call <vilib>:"C DIO Read.vi"("error in (no error)"=w108, "DIO Info In in"=w109) -> ("error out"=w85:errorcluster, "IN"=→"TASK ENABLE":bool, "DIO Info In out"=w110:T22)  [unwired: 7 in]
    n20 = call <vilib>:"C DIO Read.vi"("error in (no error)"=w116, "DIO Info In in"=w118) -> ("error out"=w87:errorcluster, "IN"=w115:bool, "DIO Info In out"=w117:T22)  [unwired: 7 in]
    n21 = call <vilib>:"NavX Open.vi"("I2C Channel"=I2C_Channel."A") -> ("error out"=w104:errorcluster, "NavX Info"=w106:T28)  [unwired: 9 in]
    n22 = Not(x="Red LED") -> (.not. x?=w77:bool)
    n23 = call "Digital Debounce Filter.vi"("Boolean input"=w115) -> ("Rising Edge"=→"Rising Edge":bool)  [unwired: 1 in, 2 out]
    n24 = call "Arduino Interfacing VI.vi"("AE Mode"=Arduino_Interfacing."Read From Arduino") -> ("error out"=w88:errorcluster, "Arduino Data"=w90:T17)  [unwired: 3 in]
    "Arduino Data" <- w90
    n25 = And(x=w77, y="Green LED") -> (x .and. y?=w79:bool)
    n26 = call <vilib>:"DIO Write.vi"("error in (no error)"=w98, "Input"=w79, "DIO Info In"=w99) -> ("error out"=w82:errorcluster, "DIO Info Out"=w97:T22)  [unwired: 7 in]
    n27 = Unbundle By Name(w90) -> ("Rotary Switch"=→"Task selection":u8)
    n28 = call "navX reading VI.vi"("NavX Info In"=w106, "Mode"=navX_type_def."Get i2C reference", "error in (no error)"=w104) -> ("NavX Info Out"=w95:T28, "Error Out"=w84:errorcluster)  [unwired: 2 out]
    n29 = call "navX reading VI.vi"("NavX Info In"=w95, "Mode"=navX_type_def."Read Values", "error in (no error)"=w84) -> ("NavX Info Out"=w94:T28, "NavX Readings"=→"NavX Readings":T16, "Status"=→"Status":T14, "Error Out"=w93:errorcluster)
    n30 = Merge Errors(w88, w87, w86, w85, w84, w83, w82) -> (w80:errorcluster)
    "General Errors" <- w80
    n31 = call "FGV Stop.vi"("Init/Read/Write State"=States_for_Action_Engine."Read") -> ("Output node"=w120:bool)  [unwired: 2 in, 1 out]
    n32 = Unbundle By Name(w80) -> ("status"=w78:bool)
    n33 = local write "Red LED"(w78) -> ()
    n34 = Wait (ms)(milliseconds to wait=u32 50) -> ()  [unwired: 1 out]
    "Robot ready" <- "Green LED"
    "Errors detected" <- "Red LED"
  }
  n35 = while {
    tunnel: w60 -> [w138]
    tunnel: w61 -> [w137]
    tunnel: [w136] -> w67
    tunnel: [w135] -> w66
    tunnel: w65 -> [w134]
    tunnel: [w133] -> w63
    tunnel: w64 -> [w132]
    tunnel: [w131] -> w62
    stop <- w129 stop-if-true
    # "Generate USER Event Loop"
    n36 = local read "Rising Edge"() -> (w126:bool)
    n37 = Or(x="OK Button", y=w126) -> (x .or. y?=w125:bool)
    n38 = local read "TASK ENABLE"() -> (w124:bool)
    n39 = And(x=w125, y=w124) -> (x .and. y?=w123:bool)
    n40 = case shown="True" w123 {
      selector: w123 -> [_ w149]
      tunnel: w138 -> [w148 w153]
      tunnel: [w148 w152] -> w135
      tunnel: w134 -> [w147 w151]
      tunnel: [w147 w150] -> w133
      frame False {
      }
      frame True {
        n41 = Generate User Event(user event=w153, event data cluster=w149, error in=w151) -> (user event out=w152:refnum<user-event>, error out=w150:errorcluster)  [unwired: 1 in]
      }
    }
    n42 = case shown="False" "STOP" {
      selector: "STOP" -> [_ w142]
      tunnel: w137 -> [w141 w146]
      tunnel: [w141 w145] -> w136
      tunnel: w132 -> [w140 w144]
      tunnel: [w140 w143] -> w131
      tunnel: [FALSE w142] -> w129
      frame False {
      }
      frame True {
        n43 = Generate User Event(user event=w146, event data cluster=w142, error in=w144) -> (user event out=w145:refnum<user-event>, error out=w143:errorcluster)  [unwired: 1 in]
      }
    }
    n44 = Wait (ms)(milliseconds to wait=u32 10) -> ()  [unwired: 1 out]
    n45 = call "FGV Stop.vi"("Init/Read/Write State"=States_for_Action_Engine."Write", "Input Node"=w129) -> ()  [unwired: 1 in, 2 out]
  }
  n46 = while {
    tunnel: w59 -> [w160]
    tunnel: [w159] -> w58
    tunnel: w46 -> [w157]
    tunnel: [w156] -> w57
    tunnel: w52 -> [w155]
    tunnel: [w154] -> w49
    stop <- w158 stop-if-true
    # "EVENT Handling Loop"
    n47 = event shown="[1] <Start Task>: User Event" {
      selector: w160 -> [_ _ _]
      dyn-events: [_ _ _] -> w159
      timeout: _ -> [_ _ _]
      tunnel: [FALSE FALSE w207] -> w158
      tunnel: w157 -> [w165 w174 w205]
      tunnel: [w164 w173 w206] -> w156
      tunnel: w155 -> [w163 w172 w204]
      tunnel: [w162 w171 w203] -> w154
      event Timeout {
        n48 = event-data() -> ()  [unwired: 1 in, 3 out]
        n49 = Enqueue Element(queue=w165, element=Intruction_Type_Definitions."Start Task 1" ("Enum"), error in (no error)=w163) -> (queue out=w164:refnum<queue>, error out=w162:errorcluster)  [unwired: 1 in, 1 out]
      }
      event User Event {
        n50 = event-data() -> ()  [unwired: 1 in, 5 out]
        n51 = call "Arduino Interfacing VI.vi"("AE Mode"=Arduino_Interfacing."Read From Arduino") -> ("Arduino Data"=w168:T17)  [unwired: 3 in, 1 out]
        n52 = Unbundle By Name(w168) -> ("Rotary Switch"=w167:u8)
        n53 = case shown="15" w167 {
          tunnel: [Intruction_Type_Definitions."Start Task 1" ("Enum") Intruction_Type_Definitions."Start Task 2" ("Enum") Intruction_Type_Definitions."Start Task 3" ("Enum") Intruction_Type_Definitions."Start Task 4" ("Enum") Intruction_Type_Definitions."Start Task 5" ("Enum") Intruction_Type_Definitions."Start Task 6" ("Enum") Intruction_Type_Definitions."Start Task 7" ("Enum") Intruction_Type_Definitions."Start Task 8 - BALL" ("Enum") Intruction_Type_Definitions."Start Task 8 - Soap" ("Enum") Intruction_Type_Definitions."Start Task 8 - Gel" ("Enum") Intruction_Type_Definitions."Start Task 8 - Pipe" ("Enum") Intruction_Type_Definitions."Start Task 9" ("Enum") Intruction_Type_Definitions."Start Task 9" ("Enum") Intruction_Type_Definitions."Start Task 9" ("Enum") Intruction_Type_Definitions."Start Task 9" ("Enum") Intruction_Type_Definitions."Start Task 9" ("Enum")] -> w170
          frame 0, Default {
          }
          frame 1 {
          }
          frame 2 {
          }
          frame 3 {
          }
          frame 4 {
          }
          frame 5 {
          }
          frame 6 {
          }
          frame 7 {
          }
          frame 8 {
          }
          frame 9 {
          }
          frame 10 {
          }
          frame 11 {
            # "Task 9: Red Detection"
            n54 = call "Box Colour FGV.vi"("Colour to detect"=Box_Colour_FGV_Colours."Blue", "Init/R/W State"=Box_Colour_FGV_States."Write") -> ()  [unwired: 8 in, 2 out]
          }
          frame 12 {
            # "Task 9: Black Detection"
            n55 = call "Box Colour FGV.vi"("Colour to detect"=Box_Colour_FGV_Colours."Black", "Init/R/W State"=Box_Colour_FGV_States."Write") -> ()  [unwired: 8 in, 2 out]
          }
          frame 13 {
            # "Task 9: Blue Detection"
            n56 = call "Box Colour FGV.vi"("Colour to detect"=Box_Colour_FGV_Colours."Green", "Init/R/W State"=Box_Colour_FGV_States."Write") -> ()  [unwired: 8 in, 2 out]
          }
          frame 14 {
            # "Task 9: Yellow Detection"
            n57 = call "Box Colour FGV.vi"("Colour to detect"=Box_Colour_FGV_Colours."Red", "Init/R/W State"=Box_Colour_FGV_States."Write") -> ()  [unwired: 8 in, 2 out]
          }
          frame 15 {
            # "Task 9: Green Detection"
            n58 = call "Box Colour FGV.vi"("Colour to detect"=Box_Colour_FGV_Colours."Yellow", "Init/R/W State"=Box_Colour_FGV_States."Write") -> ()  [unwired: 8 in, 2 out]
          }
        }
        "Selected Task" <- w170
        n59 = Enqueue Element(queue=w174, element=w170, error in (no error)=w172) -> (queue out=w173:refnum<queue>, error out=w171:errorcluster)  [unwired: 1 in, 1 out]
      }
      event User Event {
        n60 = event-data() -> ("Stop Queue"=w207:bool)  [unwired: 1 in, 4 out]
        n61 = Enqueue Element At Opposite End(queue=w205, element=Intruction_Type_Definitions."Exit" ("Enum"), error in (no error)=w204) -> (queue out=w206:refnum<queue>, error out=w203:errorcluster)  [unwired: 1 in, 1 out]
      }
    }
  }
  n62 = while {
    tunnel: w46 -> [w210]
    tunnel: w47 -> [w268]
    tunnel: w50 -> [w266]
    tunnel: [w265] -> _
    tunnel: [w264] -> w40
    shift-right: [w257] -> _
    shift-left: T9 {"PING_A"=0, "PING_B"=0, "PING_C"=0, "PING_D"=0} -> [w259]
    shift-right: [w251] -> _
    shift-left: State_Type_Definitions,_for_0.26g_versions_and_later_3."Startup" ("Enum") -> [w254]
    shift-right: [w247] -> _
    shift-left: T8 {"xDistance"=0.0, "yDistance"=0.0, "wDistance"=0.0} -> [w249]
    shift-right: [w244] -> _
    shift-left: _ -> [w243]
    shift-right: [w240] -> _
    shift-left: T11 {"Recognized Object"=FALSE, "Object X coordinate"=0.0, "Object Y coordinate"=0.0} -> [w242]
    shift-right: [w237] -> _
    shift-left: T7 {"y Stepper Position"=0, "z Stepper Position"=0} -> [w239]
    shift-right: [w234] -> _
    shift-left: T6 {"Yaw"=0.0, "Compass"=0.0} -> [w236]
    shift-right: [w231] -> _
    shift-left: T3 {"Time up flag"=FALSE, "SET TIME TO CHECK"=0.0} -> [w233]
    shift-right: [w229] -> _
    shift-left: T20 {"yStepper desired"=0} -> [w230]
    shift-right: [w225] -> _
    shift-left: T5 {"Left IR Sensor"=0.0, "Arm IR Sensor"=0.0, "Bottom IR Sensor"=0.0} -> [w227]
    shift-right: [w223] -> _
    shift-left: T19 {"ySpeed"=0.0, "xSpeed"=0.0, "wSpeed"=0.0} -> [w224]
    shift-right: [w220] -> _
    shift-left: T4 {"Line Detected?"=FALSE, "S1"=0.0, "S2"=0.0, "S3"=0.0, "S4"=0.0} -> [w222]
    shift-right: [w218] -> _
    shift-left: _ -> [w217]
    shift-right: [w209] -> _
    shift-left: T1 {"Red"=FALSE, "Black"=FALSE, "Blue"=FALSE, "Yellow"=FALSE, "Green"=FALSE, "Unknown"=FALSE, "Image processing done"=FALSE, "Colour"=enum."None"} -> [w212]
    stop <- w256 stop-if-true
    # ">>> Box Colour Detection >>>"
    # ">>State Logic Queue Reference >>"
    # ">>Action Queue>>"
    # ">>State Logic Queue Reference >>"
    # ">>> Line Sensor Cluster>>>"
    # ">>> IR Sensors >>>"
    # ">>> Time cluster >>>"
    # ">>> Object detection >>>"
    # ">>> Yaw >>>"
    # ">>> Ultrasonic Sensors Detect >>>"
    # ">>> Encoders >>>"
    # ">>> Stepper position >>>"
    # ">>State Logic  >>"
    # ">> Item Selection Bias >>"
    # ">> Item Selection Bias >>"
    # ">> Item Selection Bias >>"
    # ">>State Logic  >>"
    # ">>> Motor control cluster >>>"
    # ">>> yStepper command>>>"
    # ">>True Stop Next State >>"
    # ">>Error  >>"
    # ">>Timeout>>"
    # ">>Action states Queue Reference >>"
    # "TOP LEVEL BASELINE (MAIN PROCESSING LOOP)"
    n63 = Wait (ms)(milliseconds to wait=u32 25) -> ()  [unwired: 1 out]
    n64 = Dequeue Element(queue=w268, timeout in ms (-1)=0, error in (no error)=w266) -> (queue out=w260:refnum<queue>, element=w267:string, error out=w261:errorcluster)  [unwired: 1 out]
    "Action State" <- w267
    n65 = case shown="\"READ STEPPER VALUES\"" w267 {
      tunnel: [_ _ _ _ _ _ _ _ _ _ _ _ _ _ _ _ _ _ _ _ 0 w3637 _ _ _ _ _ _ _ _ _ _ _ _ _ _ _ _ _ _ _ _ _ _ _ _ _ _ _ _ _ _ _ _ _ _ _] -> w263
      tunnel: w260 -> [_ _ _ _ _ _ _ _ _ _ _ _ _ _ _ _ _ _ _ _ _ _ _ _ _ _ _ _ _ _ _ _ _ _ _ _ _ _ _ _ _ _ _ _ _ _ _ _ _ _ _ _ _ _ _ _ _]
      tunnel: w259 -> [w3309 w3321 w3336 w3350 w3370 w3385 w3399 w3413 w3429 w3444 w3458 w3468 w3486 w3503 w3518 w3533 w3557 w3567 w3598 w3611 w3625 w3638 w3650 w3663 w3683 w3718 w3755 w3769 w3780 w3792 w3805 w3820 w3836 w3848 w3860 w3880 w3903 w3914 w3930 w3961 w3971 w3984 w3997 w4010 w4020 w4038 w4048 w4067 w4076 w4092 w4108 w4124 w4140 w4156 w4170 w4185 w4205]
      tunnel: [w3309 w3321 w3336 w3350 w3370 w3385 w3399 w3413 w3429 w3444 w3458 w3468 w3486 w3504 w3518 w3533 w3557 w3567 w3599 w3611 w3625 w3638 w3650 w3663 w3683 w3717 w3754 w3769 w3780 w3792 w3805 w3820 w3836 w3848 w3860 w3880 w3903 w3914 w3930 w3961 w3971 w3984 w3997 w4010 w4020 w4038 w4048 w4067 w4076 w4092 w4108 w4124 w4140 w4156 w4170 w4185 w4205] -> w258
      tunnel: [TRUE TRUE _ _ _ _ _ _ _ _ _ _ _ _ _ _ _ _ _ _ _ _ _ _ _ _ _ _ _ _ _ _ _ _ _ _ _ _ _ _ _ _ _ _ _ _ _ _ _ _ _ _ _ _ _ _ _] -> w256
      tunnel: w254 -> [w3307 w3319 w3335 w3349 w3369 w3384 w3398 w3412 w3428 w3443 w3457 w3467 w3485 w3502 w3517 w3531 w3550 w3566 w3597 w3610 w3622 w3635 w3649 w3662 w3682 w3716 w3753 w3768 w3779 w3791 w3797 w3819 w3835 w3847 w3859 w3879 w3902 w3913 w3924 w3955 w3970 w3983 w3996 w4009 w4019 w4029 w4047 w4066 w4075 w4091 w4107 w4123 w4139 w4155 w4169 w4175 w4193]
      tunnel: [_ _ _ _ _ _ _ _ _ _ _ _ _ _ _ _ _ _ _ _ _ TRUE _ _ _ _ _ _ _ _ _ _ _ _ _ _ _ _ _ _ _ _ _ _ _ _ _ _ _ _ _ _ _ _ _ _ _] -> w253
      tunnel: [w3307 w3319 w3335 w3349 w3369 w3384 w3398 w3412 w3428 w3443 w3457 w3467 w3485 w3502 w3517 w3531 w3550 w3566 w3597 w3610 w3622 w3635 w3649 w3662 w3682 w3716 w3753 w3768 w3779 w3791 w3797 w3819 w3835 w3847 w3859 w3879 w3902 w3913 w3924 w3955 w3970 w3983 w3996 w4009 w4019 w4029 w4047 w4066 w4075 w4091 w4107 w4123 w4139 w4155 w4169 w4175 w4193] -> w252
      tunnel: w249 -> [w3306 w3318 w3334 w3352 w3368 w3383 w3397 w3411 w3427 w3442 w3456 w3469 w3484 w3501 w3519 w3535 w3552 w3568 w3596 w3612 w3621 w3634 w3651 w3664 w3678 w3707 w3743 w3767 w3782 w3793 w3802 w3821 w3837 w3849 w3861 w3881 w3904 w3916 w3928 w3959 w3973 w3986 w3999 w4012 w4022 w4033 w4050 w4069 w4078 w4094 w4110 w4126 w4142 w4158 w4172 w4177 w4198]
      tunnel: [w3306 w3318 w3334 w3352 w3368 w3383 w3397 w3411 w3427 w3442 w3456 w3469 w3483 w3501 w3519 w3535 w3552 w3568 w3595 w3612 w3621 w3634 w3651 w3664 w3678 w3706 w3742 w3767 w3782 w3793 w3802 w3821 w3837 w3849 w3861 w3881 w3904 w3916 w3928 w3959 w3973 w3986 w3999 w4012 w4022 w4033 w4050 w4069 w4078 w4094 w4110 w4126 w4142 w4158 w4172 w4177 w4198] -> w248
      tunnel: w242 -> [w3305 w3317 w3333 w3351 w3367 w3382 w3396 w3410 w3426 w3441 w3454 w3466 w3482 w3500 w3512 w3534 w3551 w3565 w3587 w3609 w3620 w3633 w3648 w3661 w3681 w3711 w3748 w3765 w3781 w3790 w3803 w3818 w3834 w3843 w3858 w3877 w3897 w3915 w3929 w3960 w3972 w3985 w3998 w4011 w4021 w4032 w4049 w4068 w4077 w4093 w4109 w4125 w4141 w4157 w4171 w4176 w4197]
      tunnel: [w3305 w3317 w3333 w3351 w3367 w3382 w3396 w3410 w3426 w3441 w3454 w3466 w3482 w3500 w3512 w3534 w3551 w3565 w3586 w3609 w3620 w3633 w3648 w3661 w3680 w3710 w3747 w3765 w3781 w3790 w3803 w3818 w3834 w3843 w3858 w3876 w3897 w3915 w3929 w3960 w3972 w3985 w3998 w4011 w4021 w4032 w4049 w4068 w4077 w4093 w4109 w4125 w4141 w4157 w4171 w4176 w4197] -> w241
      tunnel: w239 -> [w3304 w3316 w3332 w3353 w3366 w3381 w3395 w3409 w3425 w3440 w3453 w3465 w3481 w3499 w3520 w3536 w3553 w3564 w3592 w3608 w3619 w3632 w3647 w3660 w3677 w3702 w3738 w3764 w3778 w3789 w3801 w3817 w3833 w3846 w3857 w3882 w3905 w3917 w3927 w3958 w3969 w3982 w3995 w4008 w4023 w4034 w4051 w4065 w4079 w4095 w4111 w4127 w4143 w4159 w4173 w4178 w4199]
      tunnel: [w3304 w3316 w3332 w3353 w3366 w3381 w3395 w3409 w3425 w3440 w3453 w3465 w3481 w3499 w3520 w3536 w3553 w3564 w3591 w3608 w3619 w3632 w3647 w3660 w3677 w3701 w3737 w3764 w3778 w3789 w3801 w3817 w3833 w3846 w3857 w3882 w3905 w3917 w3927 w3958 w3969 w3982 w3995 w4008 w4023 w4034 w4051 w4064 w4079 w4095 w4111 w4127 w4143 w4159 w4173 w4178 w4199] -> w238
      tunnel: w236 -> [w3303 w3315 w3330 w3354 w3364 w3379 w3393 w3408 w3423 w3438 w3452 w3464 w3480 w3492 w3515 w3537 w3554 w3563 w3582 w3607 w3618 w3631 w3646 w3659 w3676 w3698 w3734 w3763 w3775 w3788 w3800 w3816 w3832 w3845 w3856 w3883 w3906 w3918 w3926 w3957 w3968 w3979 w3992 w4005 w4024 w4035 w4052 w4059 w4080 w4096 w4112 w4128 w4144 w4160 w4174 w4179 w4200]
      tunnel: [w3303 w3315 w3330 w3354 w3364 w3379 w3393 w3408 w3423 w3438 w3452 w3464 w3480 w3492 w3514 w3537 w3554 w3563 w3581 w3607 w3618 w3631 w3646 w3659 w3676 w3697 w3733 w3763 w3775 w3788 w3800 w3816 w3832 w3845 w3856 w3883 w3906 w3918 w3926 w3957 w3968 w3979 w3992 w4005 w4024 w4035 w4052 w4059 w4080 w4096 w4112 w4128 w4144 w4160 w4174 w4179 w4200] -> w235
      tunnel: w233 -> [w3301 w3314 w3331 w3355 w3365 w3380 w3394 w3407 w3424 w3439 w3451 w3463 w3479 w3491 w3511 w3538 w3555 w3562 w3578 w3604 w3617 w3630 w3645 w3658 w3675 w3695 w3731 w3761 w3774 w3787 w3799 w3815 w3831 w3844 w3855 w3884 w3907 w3919 w3925 w3956 w3967 w3978 w3991 w4004 w4025 w4036 w4053 w4058 w4074 w4090 w4106 w4122 w4138 w4154 w4168 w4180 w4201]
      tunnel: [w3301 w3314 w3331 w3355 w3365 w3380 w3394 w3407 w3424 w3439 w3451 w3463 w3479 w3491 w3511 w3538 w3555 w3562 w3578 w3604 w3617 w3630 w3645 w3658 w3674 w3694 w3730 w3761 w3774 w3787 w3799 w3815 w3831 w3844 w3855 w3884 w3907 w3919 w3925 w3956 w3967 w3978 w3991 w4004 w4025 w4036 w4053 w4058 w4074 w4088 w4104 w4120 w4136 w4153 w4167 w4180 w4201] -> w232
      tunnel: w230 -> [_ _ _ _ _ _ _ _ _ _ _ _ _ _ _ _ _ _ _ _ _ _ _ _ _ _ _ _ _ _ _ _ _ _ _ _ _ _ _ _ _ _ _ _ _ _ w4044 _ _ _ _ _ _ _ _ _ _]
      tunnel: [w3300 w3313 w3325 w3345 w3359 w3374 w3389 w3403 w3419 w3433 w3448 w3462 w3473 w3490 w3508 w3529 w3556 w3561 w3575 w3603 w3616 w3629 w3644 w3655 w3668 w3688 w3722 w3760 w3773 w3786 w3804 w3809 w3825 w3841 w3853 w3872 w3900 w3911 w3931 w3962 w3966 w3977 w3990 w4003 w4016 w4037 w4042 w4057 w4073 w4086 w4102 w4118 w4134 w4151 w4164 w4184 w4204] -> w226
      tunnel: w227 -> [w3300 w3313 w3325 w3345 w3359 w3374 w3389 w3403 w3419 w3433 w3448 w3462 w3473 w3490 w3508 w3530 w3556 w3561 w3575 w3603 w3616 w3629 w3644 w3655 w3668 w3689 w3723 w3760 w3773 w3786 w3804 w3809 w3825 w3841 w3853 w3872 w3900 w3911 w3931 w3962 w3966 w3977 w3990 w4003 w4016 w4037 w4042 w4057 w4073 w4086 w4102 w4118 w4134 w4151 w4164 w4184 w4204]
      tunnel: w224 -> [_ _ _ _ _ _ _ _ w3418 _ _ _ _ _ _ _ _ _ _ _ _ _ _ _ _ _ _ _ _ _ _ _ _ _ _ _ _ _ _ _ _ _ _ _ _ _ _ _ _ _ _ _ _ _ _ _ _]
      tunnel: w222 -> [w3299 w3312 w3324 w3339 w3358 w3373 w3388 w3402 w3416 w3432 w3447 w3461 w3472 w3489 w3507 w3525 w3549 w3560 w3573 w3602 w3615 w3628 w3643 w3654 w3671 w3691 w3726 w3759 w3772 w3785 w3796 w3808 w3824 w3840 w3852 w3870 w3899 w3910 w3922 w3954 w3965 w3976 w3989 w4002 w4015 w4028 w4041 w4056 w4072 w4085 w4101 w4117 w4133 w4150 w4163 w4183 w4203]
      tunnel: [w3299 w3312 w3324 w3339 w3358 w3373 w3388 w3402 w3416 w3432 w3447 w3461 w3472 w3489 w3507 w3525 w3548 w3560 w3573 w3602 w3615 w3628 w3643 w3654 w3670 w3690 w3725 w3759 w3772 w3785 w3796 w3808 w3824 w3840 w3852 w3870 w3899 w3910 w3922 w3954 w3965 w3976 w3989 w4002 w4015 w4028 w4041 w4056 w4072 w4085 w4101 w4117 w4133 w4150 w4163 w4183 w4203] -> w221
      tunnel: [_ _ _ _ _ _ _ _ _ _ _ _ _ _ _ _ _ _ _ _ _ _ _ _ _ _ _ _ _ _ _ _ _ _ _ w3864 w3894 _ _ _ _ _ _ _ _ _ _ _ _ _ _ _ _ _ _ _ _] -> w219
      tunnel: w217 -> [w3298 w3311 w3323 w3338 w3357 w3372 w3387 w3401 w3415 w3431 w3446 w3460 w3471 w3488 w3506 w3524 w3540 w3559 w3571 w3601 w3614 w3627 w3642 w3653 w3672 w3692 w3727 w3758 w3771 w3784 w3795 w3807 w3823 w3839 w3851 w3866 w3898 w3909 w3921 w3953 w3964 w3975 w3988 w4001 w4014 w4027 w4040 w4055 w4071 w4084 w4100 w4116 w4132 w4149 w4162 w4182 w4202]
      tunnel: [w3298 w3311 w3323 w3338 w3357 w3372 w3387 w3401 w3415 w3431 w3446 w3460 w3471 w3488 w3506 w3524 w3540 w3559 w3571 w3601 w3614 w3627 w3642 w3653 w3672 w3692 w3727 w3758 w3771 w3784 w3795 w3807 w3823 w3839 w3851 w3866 w3898 w3909 w3921 w3953 w3964 w3975 w3988 w4001 w4014 w4027 w4040 w4055 w4071 w4084 w4100 w4116 w4132 w4149 w4162 w4182 w4202] -> w216
      tunnel: w212 -> [w3297 w3310 w3322 w3337 w3356 w3371 w3386 w3400 w3414 w3430 w3445 w3459 w3470 w3487 w3505 w3521 w3539 w3558 w3570 w3600 w3613 w3626 w3641 w3652 w3667 w3685 w3721 w3757 w3770 w3783 w3794 w3806 w3822 w3838 w3850 w3869 w3892 w3908 w3920 w3952 w3963 w3974 w3987 w4000 w4013 w4026 w4039 w4054 w4070 w4083 w4099 w4115 w4131 w4148 w4161 w4181 w4196]
      tunnel: [w3297 w3310 w3322 w3337 w3356 w3371 w3386 w3400 w3414 w3430 w3445 w3459 w3470 w3487 w3505 w3521 w3539 w3558 w3570 w3600 w3613 w3626 w3641 w3652 w3666 w3685 w3721 w3757 w3770 w3783 w3794 w3806 w3822 w3838 w3850 w3869 w3885 w3908 w3920 w3951 w3963 w3974 w3987 w4000 w4013 w4026 w4039 w4054 w4070 w4083 w4099 w4115 w4131 w4148 w4161 w4181 w4195] -> w211
      frame "Exit" {
        # ">>State Logic  >>"
        # ">>> Time cluster >>>"
        # ">>> Yaw >>>"
        # ">>> Stepper position >>>"
        # ">>> Encoders >>>"
        # ">>> Object detection >>>"
        # ">>> Ultrasonic Sensors Detect >>>"
        n66 = call "Imaq Dispose"("All Images? (No)"=TRUE) -> ()  [unwired: 5 in, 1 out]
      }
      frame "----Movement States----" {
        # ">>State Logic  >>"
        # ">>> Time cluster >>>"
        # ">>> Yaw >>>"
        # ">>> Stepper position >>>"
        # ">>> Encoders >>>"
        # ">>> Object detection >>>"
        # ">>> Ultrasonic Sensors Detect >>>"
      }
      frame "FORWARD" {
        # "High voltage values: 30\nMid voltage values: 40\nLow voltage values: 50"
        # ">>State Logic  >>"
        # ">>> Time cluster >>>"
        # ">>> Yaw >>>"
        # ">>> Stepper position >>>"
        # ">>> Encoders >>>"
        # ">>> Object detection >>>"
        # ">>> Ultrasonic Sensors Detect >>>"
        n67 = Unbundle By Name(w3330) -> ("Yaw"=w3326:dbl)
        n68 = call "MOTOR CONTROL WITH PID AE.vi"("Yaw"=w3326, "Speed"=30.0, "Direction"=MOTOR_CONTROL_WITH_PID_AE_DIRECTION_TYPE_DEF."y-axis movement", "AE Mode"=MOTOR_CONTROL_WITH_PID_AE_DATA_MODE_TYPE_DEF."Write to AE") -> ()  [unwired: 1 out]
      }
      frame "FORWARD - IR ASSIST" {
        # "Algorithm sensitivity"
        # "Distance to maintain from wall"
        # ">>State Logic  >>"
        # ">>> Time cluster >>>"
        # ">>> Yaw >>>"
        # ">>> Stepper position >>>"
        # ">>> Encoders >>>"
        # ">>> Object detection >>>"
        # ">>> Ultrasonic Sensors Detect >>>"
        n69 = Unbundle By Name(w3345) -> ("Left IR Sensor"=w3344:dbl)
        n70 = Subtract(x=w3344, y=20.0) -> (x-y=w3342:dbl)
        n71 = Multiply(x=w3342, y=0.2) -> (x*y=w3340:dbl)
        n72 = call "MOTOR CONTROL WITH PID AE.vi"("Yaw"=w3340, "Speed"=35.0, "Direction"=MOTOR_CONTROL_WITH_PID_AE_DIRECTION_TYPE_DEF."y-axis movement", "AE Mode"=MOTOR_CONTROL_WITH_PID_AE_DATA_MODE_TYPE_DEF."Write to AE") -> ()  [unwired: 1 out]
      }
      frame "LEFT" {
        # ">>State Logic  >>"
        # ">>> Time cluster >>>"
        # ">>> Yaw >>>"
        # ">>> Stepper position >>>"
        # ">>> Encoders >>>"
        # ">>> Object detection >>>"
        # ">>> Ultrasonic Sensors Detect >>>"
        n73 = Unbundle By Name(w3364) -> ("Yaw"=w3361:dbl)
        n74 = call "MOTOR CONTROL WITH PID AE.vi"("Yaw"=w3361, "Speed"=-25.0, "Direction"=MOTOR_CONTROL_WITH_PID_AE_DIRECTION_TYPE_DEF."x-axis movement", "AE Mode"=MOTOR_CONTROL_WITH_PID_AE_DATA_MODE_TYPE_DEF."Write to AE") -> ()  [unwired: 1 out]
      }
      frame "RIGHT" {
        # ">>> Time cluster >>>"
        # ">>> Yaw >>>"
        # ">>> Stepper position >>>"
        # ">>> Encoders >>>"
        # ">>> Object detection >>>"
        # ">>> Ultrasonic Sensors Detect >>>"
        n75 = Unbundle By Name(w3379) -> ("Yaw"=w3375:dbl)
        n76 = call "MOTOR CONTROL WITH PID AE.vi"("Yaw"=w3375, "Speed"=25.0, "Direction"=MOTOR_CONTROL_WITH_PID_AE_DIRECTION_TYPE_DEF."x-axis movement", "AE Mode"=MOTOR_CONTROL_WITH_PID_AE_DATA_MODE_TYPE_DEF."Write to AE") -> ()  [unwired: 1 out]
      }
      frame "R-ACW" {
        # ">>> IR Sensors >>>"
        # ">>> Time cluster >>>"
        # ">>> Yaw >>>"
        # ">>> Stepper position >>>"
        # ">>> Encoders >>>"
        # ">>> Object detection >>>"
        # ">>> Ultrasonic Sensors Detect >>>"
        n77 = call "MOTOR CONTROL WITH PID AE.vi"("Speed"=10.0, "Direction"=MOTOR_CONTROL_WITH_PID_AE_DIRECTION_TYPE_DEF."rotation", "AE Mode"=MOTOR_CONTROL_WITH_PID_AE_DATA_MODE_TYPE_DEF."Write to AE") -> ()  [unwired: 1 in, 1 out]
      }
      frame "R-CW" {
        (unwired) -0.2 ("Speed")
        # ">>> Time cluster >>>"
        # ">>> Yaw >>>"
        # ">>> Stepper position >>>"
        # ">>> Encoders >>>"
        # ">>> Object detection >>>"
        # ">>> Ultrasonic Sensors Detect >>>"
        n78 = call "MOTOR CONTROL WITH PID AE.vi"("Speed"=-10.0, "Direction"=MOTOR_CONTROL_WITH_PID_AE_DIRECTION_TYPE_DEF."rotation", "AE Mode"=MOTOR_CONTROL_WITH_PID_AE_DATA_MODE_TYPE_DEF."Write to AE") -> ()  [unwired: 1 in, 1 out]
      }
      frame "X AXIS - SLOW" {
        # ">>> Line Sensor Cluster>>>"
        # ">>> IR Sensors >>>"
        # ">>> Time cluster >>>"
        # ">>> Yaw >>>"
        # ">>> Stepper position >>>"
        # ">>> Encoders >>>"
        # ">>> Object detection >>>"
        # ">>> Ultrasonic Sensors Detect >>>"
        n79 = Unbundle By Name(w3418) -> ("xSpeed"=w3417:dbl)
        n80 = Unbundle By Name(w3423) -> ("Yaw"=w3420:dbl)
        n81 = call "MOTOR CONTROL WITH PID AE.vi"("Yaw"=w3420, "Speed"=w3417, "Direction"=MOTOR_CONTROL_WITH_PID_AE_DIRECTION_TYPE_DEF."x-axis movement", "AE Mode"=MOTOR_CONTROL_WITH_PID_AE_DATA_MODE_TYPE_DEF."Write to AE") -> ()  [unwired: 1 out]
      }
      frame "REVERSE" {
        # ">>> Time cluster >>>"
        # ">>> Yaw >>>"
        # ">>> Stepper position >>>"
        # ">>> Encoders >>>"
        # ">>> Object detection >>>"
        # ">>> Ultrasonic Sensors Detect >>>"
        n82 = Unbundle By Name(w3438) -> ("Yaw"=w3434:dbl)
        n83 = call "MOTOR CONTROL WITH PID AE.vi"("Yaw"=w3434, "Speed"=-40.0, "Direction"=MOTOR_CONTROL_WITH_PID_AE_DIRECTION_TYPE_DEF."y-axis movement", "AE Mode"=MOTOR_CONTROL_WITH_PID_AE_DATA_MODE_TYPE_DEF."Write to AE") -> ()  [unwired: 1 out]
      }
      frame "STOP" {
        n84 = Wait (ms)(milliseconds to wait=u32 100) -> ()  [unwired: 1 out]
        n85 = call "MOTOR CONTROL WITH PID AE.vi"("Direction"=MOTOR_CONTROL_WITH_PID_AE_DIRECTION_TYPE_DEF."stop", "AE Mode"=MOTOR_CONTROL_WITH_PID_AE_DATA_MODE_TYPE_DEF."Write to AE") -> ()  [unwired: 2 in, 1 out]
      }
      frame "----SENSOR READING---- " {
      }
      frame "READ ENCODERS" {
        # ">>> Time cluster >>>"
        # ">>> Yaw >>>"
        # ">>> Stepper position >>>"
        # ">>> Object detection >>>"
        # ">>> Current encoder distance >>>"
        # ">>> Ultrasonic Sensors Detect >>>"
        n86 = call "MOTOR CONTROL WITH PID AE.vi"("AE Mode"=MOTOR_CONTROL_WITH_PID_AE_DATA_MODE_TYPE_DEF."Read from AE") -> ("Speed & distance"=w3477:T15)  [unwired: 3 in]
        n87 = Unbundle By Name(w3477) -> ("xDistance"=w3476:dbl, "yDistance"=w3475:dbl, "wDistance"=w3474:dbl)
        n88 = Bundle By Name(cluster=w3484, "xDistance"=w3476, "yDistance"=w3475, "wDistance"=w3474) -> (w3483:T8)
      }
      frame "READ ULTRASONIC" {
        (unwired) navX_type_def."Read Values" ("Mode")
        (unwired) MOTOR_CONTROL_NO_PID_Type_Def."Latch" ("Direction")
        # ">>> Line Sensor Cluster>>>"
        # ">>> IR Sensors >>>"
        # ">>State Logic  >>"
        # ">>> Time cluster >>>"
        # ">>> Ultrasonic Sensors Detect >>>"
        # ">>> Object detection >>>"
        # ">>> Encoders >>>"
        # ">>> Stepper position >>>"
        # ">>> Yaw >>>"
        n89 = call "Arduino Interfacing VI.vi"("AE Mode"=Arduino_Interfacing."Read From Arduino") -> ("Arduino Data"=w3497:T17)  [unwired: 3 in, 1 out]
        n90 = Unbundle By Name(w3497) -> ("PING A"=w3496:u8, "PING B"=w3495:u8, "PING C"=w3494:u8, "PING D"=w3493:u8)
        n91 = Bundle By Name(cluster=w3503, "PING_A"=w3496, "PING_B"=w3495, "PING_C"=w3494, "PING_D"=w3493) -> (w3504:T9)
      }
      frame "READ NAVX" {
        # ">> Item Selection Bias >>"
        # ">>State Logic  >>"
        # ">>> Line Sensor Cluster>>>"
        # ">>> IR Sensors >>>"
        # ">>> Time cluster >>>"
        # ">>> Yaw >>>"
        # ">>> Ultrasonic Sensors Detect >>>"
        # ">>> Object detection >>>"
        # ">>> Encoders >>>"
        # ">>> Stepper position >>>"
        n92 = call "navX reading VI.vi"("Mode"=navX_type_def."Read Values") -> ("NavX Readings"=w3510:T16)  [unwired: 2 in, 3 out]
        n93 = Unbundle By Name(w3510) -> ("Heading"=w3509:dbl)
        n94 = Unbundle By Name(w3510) -> ("Yaw"=w3513:dbl)
        n95 = Bundle By Name(cluster=w3515, "Yaw"=w3513, "Compass"=w3509) -> (w3514:T6)
      }
      frame "READ IR" {
        w3523 = T38 [enum."B/AI2"] items=["Not Connected", "AudioIn/Left", "AudioIn/Right", "C/AI0", "C/AI1", "A/AI0", "A/AI1", "A/AI2", "A/AI3", "A/AI4", "A/AI5", "A/AI6", "A/AI7", "B/AI0", "B/AI1", "B/AI2", "B/AI3", "B/AI4", "B/AI5", "B/AI6", "B/AI7", "AI/AI0", "AI/AI1", "AI/AI2", "AI/AI3", "A/AI0 (DIFF)", "A/AI1 (DIFF)", "A/AI2 (DIFF)", "A/AI3 (DIFF)", "B/AI0 (DIFF)", "B/AI1 (DIFF)", "B/AI2 (DIFF)", "B/AI3 (DIFF)"] ("AI Channel")
        w3527 = T38 [enum."B/AI1"] items=["Not Connected", "AudioIn/Left", "AudioIn/Right", "C/AI0", "C/AI1", "A/AI0", "A/AI1", "A/AI2", "A/AI3", "A/AI4", "A/AI5", "A/AI6", "A/AI7", "B/AI0", "B/AI1", "B/AI2", "B/AI3", "B/AI4", "B/AI5", "B/AI6", "B/AI7", "AI/AI0", "AI/AI1", "AI/AI2", "AI/AI3", "A/AI0 (DIFF)", "A/AI1 (DIFF)", "A/AI2 (DIFF)", "A/AI3 (DIFF)", "B/AI0 (DIFF)", "B/AI1 (DIFF)", "B/AI2 (DIFF)", "B/AI3 (DIFF)"] ("AI Channel")
        w3532 = T38 [enum."B/AI0"] items=["Not Connected", "AudioIn/Left", "AudioIn/Right", "C/AI0", "C/AI1", "A/AI0", "A/AI1", "A/AI2", "A/AI3", "A/AI4", "A/AI5", "A/AI6", "A/AI7", "B/AI0", "B/AI1", "B/AI2", "B/AI3", "B/AI4", "B/AI5", "B/AI6", "B/AI7", "AI/AI0", "AI/AI1", "AI/AI2", "AI/AI3", "A/AI0 (DIFF)", "A/AI1 (DIFF)", "A/AI2 (DIFF)", "A/AI3 (DIFF)", "B/AI0 (DIFF)", "B/AI1 (DIFF)", "B/AI2 (DIFF)", "B/AI3 (DIFF)"] ("AI Channel")
        # ">>> Line Sensor Cluster>>>"
        # ">>> IR Sensors >>>"
        # ">>State Logic  >>"
        # ">>> Time cluster >>>"
        # ">>> Ultrasonic Sensors Detect >>>"
        # ">>> Object detection >>>"
        # ">>> Encoders >>>"
        # ">>> Stepper position >>>"
        # ">>> Yaw >>>"
        n96 = call <vilib>:"Sharp IR.vi"("AI Channel"=w3532) -> ("Sharp IR Distance"=w3528:dbl)  [unwired: 8 in, 2 out]
        n97 = call <vilib>:"Sharp IR.vi"("AI Channel"=w3527) -> ("Sharp IR Distance"=w3526:dbl)  [unwired: 8 in, 2 out]
        n98 = call <vilib>:"Sharp IR.vi"("AI Channel"=w3523) -> ("Sharp IR Distance"=w3522:dbl)  [unwired: 8 in, 2 out]
        n99 = Bundle By Name(cluster=w3530, "Left IR Sensor"=w3528, "Arm IR Sensor"=w3526, "Bottom IR Sensor"=w3522) -> (w3529:T5)
      }
      frame "READ LINE SENSOR" {
        # ">>> IR Sensors >>>"
        # ">>> Line Sensor Cluster>>>"
        # ">>State Logic  >>"
        # ">>> Time cluster >>>"
        # ">>> Object detection >>>"
        # ">>> Yaw >>>"
        # ">>> Ultrasonic Sensors Detect >>>"
        # ">>> Encoders >>>"
        # ">>> Stepper position >>>"
        n100 = call "Line Sensor AE.vi"("AE State"=Line_Sensor_AE_Type_Def."READ FROM LINE SENSORS") -> ("Line Detected?"=w3546:bool, "Line Sensor Raw Values"=w3545:T40)
        n101 = Unbundle By Name(w3545) -> ("S1"=w3544:dbl, "S2"=w3543:dbl, "S3"=w3542:dbl, "S4"=w3541:dbl)
        n102 = Bundle By Name(cluster=w3549, "Line Detected?"=w3546, "S1"=w3544, "S2"=w3543, "S3"=w3542, "S4"=w3541) -> (w3548:T4)
      }
      frame "----SYSTEM MODES----" {
        (unwired) I2C_MASTER_Type_Def."Last State" ("Arduino Mode")
        # ">>> Object detection >>>"
        # ">>> Yaw >>>"
        # ">>> Ultrasonic Sensors Detect >>>"
        # ">>> Encoders >>>"
        # ">>> Stepper position >>>"
      }
      frame "INIT" {
        w3593 = u8 0
        w3594 = 0.0
        # ">>> IR Sensors >>>"
        # ">>> IR Sensors >>>"
        # ">>> Line Sensor Cluster>>>"
        # ">>> Time cluster >>>"
        # ">>> Object detection >>>"
        # ">>> Yaw >>>"
        # ">>> Ultrasonic Sensors Detect >>>"
        # ">>> Encoders >>>"
        # ">>> Stepper position >>>"
        # ">>State Logic  >>"
        n103 = call "Arduino Interfacing VI.vi"("AE Mode"=Arduino_Interfacing."Initialize") -> ()  [unwired: 3 in, 2 out]
        n104 = call "FGV Stop.vi"("Init/Read/Write State"=States_for_Action_Engine."Initialize") -> ()  [unwired: 2 in, 2 out]
        n105 = call "Elasped Timer.vi"("Action"=Elapsed_timer_control."Initialize") -> ()  [unwired: 7 in, 4 out]
        n106 = call "MOTOR CONTROL WITH PID AE.vi"("AE Mode"=MOTOR_CONTROL_WITH_PID_AE_DATA_MODE_TYPE_DEF."Init AE") -> ()  [unwired: 3 in, 1 out]
        n107 = call "IMAQ Reference AE.vi"("IMAQ AE States"=IMAQ_Reference_AE."Initialize AE") -> ()  [unwired: 1 in, 2 out]
        n108 = call "Line Sensor AE.vi"("AE State"=Line_Sensor_AE_Type_Def."INIT AE") -> ()  [unwired: 2 out]
        n109 = Bundle By Name(cluster=w3587, "Recognized Object"=FALSE, "Object X coordinate"=0.0, "Object Y coordinate"=0.0) -> (w3586:T11)
        n110 = Bundle By Name(cluster=w3592, "y Stepper Position"=u8 0, "z Stepper Position"=u8 0) -> (w3591:T7)
        n111 = Bundle By Name(cluster=w3596, "xDistance"=w3594, "yDistance"=w3594, "wDistance"=w3594) -> (w3595:T8)
        n112 = Bundle By Name(cluster=w3598, "PING_A"=w3593, "PING_B"=w3593, "PING_C"=w3593, "PING_D"=w3593) -> (w3599:T9)
        n113 = invoke class="VI" method="Default Vals.Reinit All"() -> ()  [unwired: 3 in, 3 out]
        n114 = Bundle By Name(cluster=w3582, "Yaw"=0.0) -> (w3581:T6)
        n115 = call "Box Colour FGV.vi"("Init/R/W State"=Box_Colour_FGV_States."Initialize") -> ()  [unwired: 9 in, 2 out]
      }
      frame "ARDUINO - ULTRASONIC" {
        # ">>> Time cluster >>>"
        # ">>> Line Sensor Cluster>>>"
        # ">>> Object detection >>>"
        # ">>> Yaw >>>"
        # ">>> Ultrasonic Sensors Detect >>>"
        # ">>> Encoders >>>"
        # ">>> Stepper position >>>"
        # ">>State Logic  >>"
        n116 = call "Arduino Interfacing VI.vi"("Data to Write"=I2C_MASTER_WRITE_NEW_Type_Def."Ultrasonic sensors", "AE Mode"=Arduino_Interfacing."Write to Arduino") -> ()  [unwired: 2 in, 2 out]
      }
      frame "NAVX CALIBRATE" {
        # ">>> Object detection >>>"
        # ">>> Yaw >>>"
        # ">>> Ultrasonic Sensors Detect >>>"
        # ">>> Encoders >>>"
        # ">>> Stepper position >>>"
        # ">>State Logic  >>"
        # "Adds a 15 second delay to the startup process \nfor the NavX to calibrate"
        n117 = Wait (ms)(milliseconds to wait=u32 1000) -> ()  [unwired: 1 out]
      }
      frame "NO ACTION", Default {
        (unwired) u8 0 ("y Stepper value")
        (unwired) TRUE ("Latch")
        (unwired) navX_type_def."Read Values" ("Mode")
        (unwired) MOTOR_CONTROL_NO_PID_Type_Def."Latch" ("Direction")
        # ">>> Object detection >>>"
        # ">>> Yaw >>>"
        # ">>> Ultrasonic Sensors Detect >>>"
        # ">>> Encoders >>>"
        # ">>> Stepper position >>>"
        # ">>State Logic  >>"
        n118 = case shown="\"Idle\"" w3635 {
          tunnel: [0 100] -> w3637
          frame "Startup", Default {
          }
          frame "Idle" {
          }
        }
      }
      frame "----RESET CASES----" {
        (unwired) I2C_MASTER_Type_Def."Last State" ("Arduino Mode")
        # ">>> Object detection >>>"
        # ">>> Yaw >>>"
        # ">>> Ultrasonic Sensors Detect >>>"
        # ">>> Encoders >>>"
        # ">>> Stepper position >>>"
        # ">>State Logic  >>"
      }
      frame "RESET ENCODERS" {
        # ">>> Object detection >>>"
        # ">>> Yaw >>>"
        # ">>> Ultrasonic Sensors Detect >>>"
        # ">>> Encoders >>>"
        # ">>> Stepper position >>>"
        # ">>State Logic  >>"
        n119 = call "MOTOR CONTROL WITH PID AE.vi"("Direction"=MOTOR_CONTROL_WITH_PID_AE_DIRECTION_TYPE_DEF."reset encoders", "AE Mode"=MOTOR_CONTROL_WITH_PID_AE_DATA_MODE_TYPE_DEF."Write to AE") -> ()  [unwired: 2 in, 1 out]
      }
      frame "RESET FLAGS" {
        w3665 = FALSE ("Line Detected?")
        # ">>> Line Sensor Cluster>>>"
        # ">>> IR Sensors >>>"
        # ">>> Time cluster >>>"
        # ">>> Object detection >>>"
        # ">>> Yaw >>>"
        # ">>> Ultrasonic Sensors Detect >>>"
        # ">>> Encoders >>>"
        # ">>> Stepper position >>>"
        # ">>> Line Sensor Cluster>>>"
        # ">>> IR Sensors >>>"
        # ">>> Time cluster >>>"
        # ">>> Object detection >>>"
        # ">>> Yaw >>>"
        # ">>> Ultrasonic Sensors Detect >>>"
        # ">>> Encoders >>>"
        # ">>> Stepper position >>>"
        # "Resets BOOLEAN FLAGS only"
        n120 = Wait (ms)(milliseconds to wait=u32 20) -> ()  [unwired: 1 out]
        n121 = Bundle By Name(cluster=w3681, "Recognized Object"=FALSE) -> (w3680:T11)
        n122 = Bundle By Name(cluster=w3671, "Line Detected?"=FALSE) -> (w3670:T4)
        n123 = Bundle By Name(cluster=w3675, "Time up flag"=FALSE) -> (w3674:T3)
        n124 = Bundle By Name(cluster=w3667, "Red"=w3665, "Black"=w3665, "Blue"=w3665, "Yellow"=w3665, "Green"=w3665, "Unknown"=w3665, "Image processing done"=w3665) -> (w3666:T1)
      }
      frame "RESET SENSOR VALUES" {
        w3686 = 0.0 ("S4")
        w3687 = 0.0 ("S4")
        # "Resets SENSOR VALUES only"
        # ">>> Line Sensor Cluster>>>"
        # ">>> IR Sensors >>>"
        # ">>> Time cluster >>>"
        # ">>> Object detection >>>"
        # ">>> Yaw >>>"
        # ">>> Ultrasonic Sensors Detect >>>"
        # ">>> Encoders >>>"
        # ">>> Stepper position >>>"
        # ">>> Line Sensor Cluster>>>"
        # ">>> IR Sensors >>>"
        # ">>> Time cluster >>>"
        # ">>> Object detection >>>"
        # ">>> Yaw >>>"
        # ">>> Ultrasonic Sensors Detect >>>"
        # ">>> Encoders >>>"
        # ">>> Stepper position >>>"
        # "Resets any software variables\nand/or non-critical states"
        n125 = Wait (ms)(milliseconds to wait=u32 20) -> ()  [unwired: 1 out]
        n126 = Bundle By Name(cluster=w3695, "SET TIME TO CHECK"=0.0) -> (w3694:T3)
        n127 = Bundle By Name(cluster=w3711, "Object X coordinate"=0.0, "Object Y coordinate"=0.0) -> (w3710:T11)
        n128 = Bundle By Name(cluster=w3702, "y Stepper Position"=u8 0, "z Stepper Position"=u8 0) -> (w3701:T7)
        n129 = Bundle By Name(cluster=w3689, "Left IR Sensor"=w3686, "Arm IR Sensor"=w3686) -> (w3688:T5)
        n130 = Bundle By Name(cluster=w3707, "xDistance"=0.0, "yDistance"=0.0, "wDistance"=0.0) -> (w3706:T8)
        n131 = Bundle By Name(cluster=w3718, "PING_A"=u8 0, "PING_B"=u8 0, "PING_C"=u8 0, "PING_D"=u8 0) -> (w3717:T9)
        n132 = Bundle By Name(cluster=w3698, "Yaw"=0.0) -> (w3697:T6)
        n133 = Bundle By Name(cluster=w3691, "S1"=w3687, "S2"=w3687, "S3"=w3687, "S4"=w3687) -> (w3690:T4)
      }
      frame "RESET ALL SENSORS" {
        w3720 = 0.0 ("SET TIME TO CHECK")
        # ">>> Line Sensor Cluster>>>"
        # ">>> IR Sensors >>>"
        # ">>> Time cluster >>>"
        # ">>> Object detection >>>"
        # ">>> Yaw >>>"
        # ">>> Ultrasonic Sensors Detect >>>"
        # ">>> Encoders >>>"
        # ">>> Stepper position >>>"
        # ">>> Line Sensor Cluster>>>"
        # ">>> IR Sensors >>>"
        # ">>> Time cluster >>>"
        # ">>> Object detection >>>"
        # ">>> Yaw >>>"
        # ">>> Ultrasonic Sensors Detect >>>"
        # ">>> Encoders >>>"
        # ">>> Stepper position >>>"
        # "Resets ALL SENSOR PARAMTERS"
        n134 = Wait (ms)(milliseconds to wait=u32 20) -> ()  [unwired: 1 out]
        n135 = Bundle By Name(cluster=w3731, "Time up flag"=FALSE, "SET TIME TO CHECK"=0.0) -> (w3730:T3)
        n136 = Bundle By Name(cluster=w3748, "Recognized Object"=FALSE, "Object X coordinate"=0.0, "Object Y coordinate"=0.0) -> (w3747:T11)
        n137 = Bundle By Name(cluster=w3738, "y Stepper Position"=u8 0, "z Stepper Position"=u8 0) -> (w3737:T7)
        n138 = Bundle By Name(cluster=w3723, "Left IR Sensor"=w3720, "Arm IR Sensor"=w3720, "Bottom IR Sensor"=w3720) -> (w3722:T5)
        n139 = Bundle By Name(cluster=w3726, "Line Detected?"=FALSE) -> (w3725:T4)
        n140 = Bundle By Name(cluster=w3743, "xDistance"=0.0, "yDistance"=0.0, "wDistance"=0.0) -> (w3742:T8)
        n141 = Bundle By Name(cluster=w3755, "PING_A"=u8 0, "PING_B"=u8 0, "PING_C"=u8 0, "PING_D"=u8 0) -> (w3754:T9)
        n142 = Bundle By Name(cluster=w3734, "Yaw"=0.0) -> (w3733:T6)
      }
      frame "RESET YAW" {
        n143 = Wait (ms)(milliseconds to wait=u32 100) -> ()  [unwired: 1 out]
        n144 = call "navX reading VI.vi"("Mode"=navX_type_def."Zero Yaw") -> ()  [unwired: 2 in, 4 out]
      }
      frame "RESET ARM" {
        n145 = call "Arduino Interfacing VI.vi"("Data to Write"=I2C_MASTER_WRITE_NEW_Type_Def."Soft Reset", "AE Mode"=Arduino_Interfacing."Write to Arduino") -> ()  [unwired: 2 in, 2 out]
      }
      frame "--------CAM STATES-------" {
      }
      frame "OPEN IMAQ REF" {
        # ">>> Line Sensor Cluster>>>"
        # ">>State Logic  >>"
        # ">>> Time cluster >>>"
        # ">>> Object detection >>>"
        # ">>> Yaw >>>"
        # ">>> Ultrasonic Sensors Detect >>>"
        # ">>> Encoders >>>"
        # ">>> Stepper position >>>"
        # ">>> IR Sensors >>>"
        n146 = call "IMAQ Reference AE.vi"("IMAQ AE States"=IMAQ_Reference_AE."Initialize AE") -> ()  [unwired: 1 in, 2 out]
      }
      frame "OPEN LOG CAM" {
        n147 = call "Webcam AE.vi"("Session In"=T36 "cam0", "Camera states"=Webcam_AE."Initialize Camera") -> ("error out"=w3812:errorcluster, "Session Out"=w3811:T36)  [unwired: 1 in, 1 out]
        n148 = call "Webcam AE.vi"("error in (no error)"=w3812, "Session In"=w3811, "Camera states"=Webcam_AE."Open Camera") -> ()  [unwired: 3 out]
      }
      frame "OPEN LIFE CAM" {
        n149 = call "Webcam AE.vi"("Session In"=T36 "cam1", "Camera states"=Webcam_AE."Initialize Camera") -> ("error out"=w3828:errorcluster, "Session Out"=w3827:T36)  [unwired: 1 in, 1 out]
        n150 = call "Webcam AE.vi"("error in (no error)"=w3828, "Session In"=w3827, "Camera states"=Webcam_AE."Open Camera") -> ()  [unwired: 3 out]
      }
      frame "CAM ACQ" {
        # ">>State Logic  >>"
        # ">>> Time cluster >>>"
        # ">>> Yaw >>>"
        # ">>> Stepper position >>>"
        # ">>> Encoders >>>"
        # ">>> Object detection >>>"
        # ">>> Ultrasonic Sensors Detect >>>"
        n151 = call "Webcam AE.vi"("Camera states"=Webcam_AE."Continuous Acquisition") -> ()  [unwired: 2 in, 3 out]
      }
      frame "CAM CLOSE" {
        # ">>> Box Colour Detection >>>"
        # ">>> Line Sensor Cluster>>>"
        # ">>> IR Sensors >>>"
        # ">>State Logic  >>"
        # ">>> Time cluster >>>"
        # ">>> Yaw >>>"
        # ">>> Stepper position >>>"
        # ">>> Encoders >>>"
        # ">>> Object detection >>>"
        # ">>> Ultrasonic Sensors Detect >>>"
        n152 = call "Webcam AE.vi"("Camera states"=Webcam_AE."Close Camera") -> ()  [unwired: 2 in, 3 out]
      }
      frame "PROCESS IMAGE" {
        # ">>> Line Sensor Cluster>>>"
        # ">>> IR Sensors >>>"
        # ">> Item Selection Bias >>"
        # ">> Item Selection Bias >>"
        # ">>State Logic  >>"
        # ">>> Time cluster >>>"
        # ">>> Yaw >>>"
        # ">>> Stepper position >>>"
        # ">>> Encoders >>>"
        # ">>> Object detection >>>"
        # ">>> Ultrasonic Sensors Detect >>>"
        n153 = call "Webcam AE.vi"("Camera states"=Webcam_AE."Retrieve Image") -> ("error out"=w3865:errorcluster, "Image Out"=w3868:T42)  [unwired: 2 in, 1 out]
        n154 = call "IMAQ Reference AE.vi"("IMAQ AE States"=IMAQ_Reference_AE."Get IMAQ Reference") -> ("Image Out"=w3867:T42)  [unwired: 1 in, 1 out]
        n155 = call "Object Detection SubVI v2.vi"("Error In"=w3865, "Mode"=w3866, "Image Dest"=w3867, "Image in"=w3868) -> ("Error out"=w3864:errorcluster, "Object Center Coordinates"=w3863:cluster{"x":sgl, "y":sgl}, "Object detection cluster"=w3862:T43)  [unwired: 1 out]
        n156 = Unbundle By Name(w3862) -> ("Object detected?"=w3873:bool)
        n157 = Unbundle By Name(w3863) -> ("x"=w3875:sgl, "y"=w3874:sgl)
        n158 = Bundle By Name(cluster=w3877, "Recognized Object"=w3873, "Object X coordinate"=w3875, "Object Y coordinate"=w3874) -> (w3876:T11)
      }
      frame "COLOUR PROCESSING" {
        # ">>> Box Colour Detection >>>"
        # ">>> Box Colour Detection >>>"
        # ">>> Line Sensor Cluster>>>"
        # ">>> IR Sensors >>>"
        # ">> Item Selection Bias >>"
        # ">> Item Selection Bias >>"
        # ">>State Logic  >>"
        # ">>> Time cluster >>>"
        # ">>> Yaw >>>"
        # ">>> Stepper position >>>"
        # ">>> Encoders >>>"
        # ">>> Object detection >>>"
        # ">>> Ultrasonic Sensors Detect >>>"
        n159 = call "Webcam AE.vi"("Camera states"=Webcam_AE."Retrieve Image") -> ("error out"=w3895:errorcluster, "Image Out"=w3896:T42)  [unwired: 2 in, 1 out]
        n160 = call "Box Colour Detection SubVI.vi"("Image In"=w3896, "Error In"=w3895) -> ("Colour output boolean cluster"=w3893:T44, "Error out"=w3894:errorcluster)  [unwired: 1 out]
        n161 = Unbundle By Name(w3893) -> ("Red"=w3891:bool, "Black"=w3890:bool, "Blue"=w3889:bool, "Yellow"=w3888:bool, "Green"=w3887:bool, "No recognizable coolour"=w3886:bool)
        n162 = Bundle By Name(cluster=w3892, "Red"=w3891, "Black"=w3890, "Blue"=w3889, "Yellow"=w3888, "Green"=w3887, "Unknown"=w3886) -> (w3885:T1)
      }
      frame "DISPOSE CAM BUFFERS" {
        # ">> Item Selection Bias >>"
        # ">>> Line Sensor Cluster>>>"
        # ">>> IR Sensors >>>"
        # ">>State Logic  >>"
        # ">>> Time cluster >>>"
        # ">>> Yaw >>>"
        # ">>> Stepper position >>>"
        # ">>> Encoders >>>"
        # ">>> Object detection >>>"
        # ">>> Ultrasonic Sensors Detect >>>"
        n163 = call "Webcam AE.vi"("Camera states"=Webcam_AE."Dispose Camera Image Buffer") -> ()  [unwired: 2 in, 3 out]
      }
      frame "DISPOSE PROC BUFFERS" {
        # ">>> Box Colour Detection >>>"
        # ">>> Line Sensor Cluster>>>"
        # ">>State Logic  >>"
        # ">>> IR Sensors >>>"
        # ">>> Time cluster >>>"
        # ">>> Object detection >>>"
        # ">>> Yaw >>>"
        # ">>> Ultrasonic Sensors Detect >>>"
        # ">>> Encoders >>>"
        # ">>> Stepper position >>>"
        n164 = call "IMAQ Reference AE.vi"("IMAQ AE States"=IMAQ_Reference_AE."Dispose Processing Buffer") -> ()  [unwired: 1 in, 2 out]
      }
      frame "BOX COLOUR" {
        # ">>> Box Colour Detection >>>"
        # ">>> Line Sensor Cluster>>>"
        # ">>State Logic  >>"
        # ">>> IR Sensors >>>"
        # ">>> Time cluster >>>"
        # ">>> Object detection >>>"
        # ">>> Yaw >>>"
        # ">>> Ultrasonic Sensors Detect >>>"
        # ">>> Encoders >>>"
        # ">>> Stepper position >>>"
        n165 = call "Box Colour Detection Sequence.vi"() -> ("Colour scan time out?"=w3948:bool, "Colour output boolean cluster"=w3950:T44)  [unwired: 9 in, 1 out]
        n166 = Unbundle By Name(w3950) -> ("Red"=w3947:bool, "Black"=w3943:bool, "Blue"=w3940:bool, "Yellow"=w3939:bool, "Green"=w3936:bool, "No recognizable coolour"=w3949:bool)
        n167 = Select(t=Box_Colour_FGV_Colours."Green" ("Colour"), s=w3936, f=Box_Colour_FGV_Colours."None" ("Colour")) -> (s? t:f=w3934:T2)
        n168 = Select(t=Box_Colour_FGV_Colours."Yellow" ("Colour"), s=w3939, f=w3934) -> (s? t:f=w3933:T2)
        n169 = Select(t=Box_Colour_FGV_Colours."Blue" ("Colour"), s=w3940, f=w3933) -> (s? t:f=w3942:T2)
        n170 = Select(t=Box_Colour_FGV_Colours."Black" ("Colour"), s=w3943, f=w3942) -> (s? t:f=w3945:T2)
        n171 = Select(t=Box_Colour_FGV_Colours."Red" ("Colour"), s=w3947, f=w3945) -> (s? t:f=w3932:T2)
        n172 = Bundle By Name(cluster=w3952, "Red"=w3947, "Black"=w3943, "Blue"=w3940, "Yellow"=w3939, "Green"=w3936, "Unknown"=w3949, "Image processing done"=w3948, "Colour"=w3932) -> (w3951:T1)
      }
      frame "-----ARM ACTIONS-----" {
      }
      frame "CLOSE CLAW" {
        n173 = call "Arduino Interfacing VI.vi"("Data to Write"=I2C_MASTER_WRITE_NEW_Type_Def."Close Claw", "AE Mode"=Arduino_Interfacing."Write to Arduino") -> ()  [unwired: 2 in, 2 out]
      }
      frame "OPEN CLAW" {
        n174 = call "Arduino Interfacing VI.vi"("Data to Write"=I2C_MASTER_WRITE_NEW_Type_Def."Open Claw", "AE Mode"=Arduino_Interfacing."Write to Arduino") -> ()  [unwired: 2 in, 2 out]
      }
      frame "Z STEPPER CAM HEIGHT" {
        n175 = call "Arduino Interfacing VI.vi"("Data to Write"=I2C_MASTER_WRITE_NEW_Type_Def."zStepper 6k", "AE Mode"=Arduino_Interfacing."Write to Arduino") -> ()  [unwired: 2 in, 2 out]
      }
      frame "Z STEPPER GRAB HEIGHT" {
        # ">>State Logic  >>"
        # ">>> Time cluster >>>"
        # ">>> Yaw >>>"
        # ">>> Stepper position >>>"
        # ">>> Encoders >>>"
        # ">>> Object detection >>>"
        # ">>> Ultrasonic Sensors Detect >>>"
        n176 = call "Arduino Interfacing VI.vi"("Data to Write"=I2C_MASTER_WRITE_NEW_Type_Def."zStepper 100", "AE Mode"=Arduino_Interfacing."Write to Arduino") -> ()  [unwired: 2 in, 2 out]
      }
      frame "Z STEPPER BOX HEIGHT" {
        # ">>> IR Sensors >>>"
        # ">>> Time cluster >>>"
        # ">>> Yaw >>>"
        # ">>> Stepper position >>>"
        # ">>> Encoders >>>"
        # ">>> Object detection >>>"
        # ">>> Ultrasonic Sensors Detect >>>"
        n177 = call "Arduino Interfacing VI.vi"("Data to Write"=I2C_MASTER_WRITE_NEW_Type_Def."zStepper 5k", "AE Mode"=Arduino_Interfacing."Write to Arduino") -> ()  [unwired: 2 in, 2 out]
      }
      frame "Y STEPPER CONTROL" {
        # ">>State Logic  >>"
        # ">>> yStepper command>>>"
        # ">>> Time cluster >>>"
        # ">>> Yaw >>>"
        # ">>> Stepper position >>>"
        # ">>> Encoders >>>"
        # ">>> Object detection >>>"
        # ">>> Ultrasonic Sensors Detect >>>"
        n178 = Unbundle By Name(w4044) -> ("yStepper desired"=w4043:u8)
        n179 = call "Arduino Interfacing VI.vi"("y Stepper value"=w4043, "Data to Write"=I2C_MASTER_WRITE_NEW_Type_Def."yStepper control", "AE Mode"=Arduino_Interfacing."Write to Arduino") -> ()  [unwired: 1 in, 2 out]
      }
      frame "READ STEPPER VALUES" {
        # ">>State Logic  >>"
        # ">>> Time cluster >>>"
        # ">>> Yaw >>>"
        # ">>> Stepper position >>>"
        # ">>> Encoders >>>"
        # ">>> Object detection >>>"
        # ">>> Ultrasonic Sensors Detect >>>"
        n180 = call "Arduino Interfacing VI.vi"("AE Mode"=Arduino_Interfacing."Read From Arduino") -> ("Arduino Data"=w4062:T17)  [unwired: 3 in, 1 out]
        n181 = Unbundle By Name(w4062) -> ("y Stepper Position"=w4061:u8, "z Stepper Position"=w4060:u8)
        n182 = Bundle By Name(cluster=w4065, "y Stepper Position"=w4061, "z Stepper Position"=w4060) -> (w4064:T7)
      }
      frame " -----TIMING-----" {
        # ">>State Logic  >>"
        # ">>> Time cluster >>>"
        # ">>> Yaw >>>"
        # ">>> Stepper position >>>"
        # ">>> Encoders >>>"
        # ">>> Object detection >>>"
        # ">>> Ultrasonic Sensors Detect >>>"
      }
      frame "SET TIMER 1" {
        w4081 = 1.0 ("Time Setting")
        # ">>State Logic  >>"
        # ">>> Time cluster >>>"
        # ">>> Yaw >>>"
        # ">>> Stepper position >>>"
        # ">>> Encoders >>>"
        # ">>> Object detection >>>"
        # ">>> Ultrasonic Sensors Detect >>>"
        n183 = Wait (ms)(milliseconds to wait=u32 250) -> ()  [unwired: 1 out]
        n184 = call "Elasped Timer.vi"("Time Setting"=w4081, "Action"=Elapsed_timer_control."Initialize") -> ()  [unwired: 6 in, 4 out]
        n185 = Bundle By Name(cluster=w4090, "Time up flag"=FALSE, "SET TIME TO CHECK"=w4081) -> (w4088:T3)
      }
      frame "SET TIMER 2" {
        w4097 = 2.0 ("Time Setting")
        # ">>State Logic  >>"
        # ">>> Time cluster >>>"
        # ">>> Yaw >>>"
        # ">>> Stepper position >>>"
        # ">>> Encoders >>>"
        # ">>> Object detection >>>"
        # ">>> Ultrasonic Sensors Detect >>>"
        n186 = Wait (ms)(milliseconds to wait=u32 250) -> ()  [unwired: 1 out]
        n187 = call "Elasped Timer.vi"("Time Setting"=w4097, "Action"=Elapsed_timer_control."Initialize") -> ()  [unwired: 6 in, 4 out]
        n188 = Bundle By Name(cluster=w4106, "Time up flag"=FALSE, "SET TIME TO CHECK"=w4097) -> (w4104:T3)
      }
      frame "SET TIMER 3" {
        w4113 = 3.0 ("Time Setting")
        # ">>State Logic  >>"
        # ">>> Time cluster >>>"
        # ">>> Yaw >>>"
        # ">>> Stepper position >>>"
        # ">>> Encoders >>>"
        # ">>> Object detection >>>"
        # ">>> Ultrasonic Sensors Detect >>>"
        n189 = Wait (ms)(milliseconds to wait=u32 250) -> ()  [unwired: 1 out]
        n190 = call "Elasped Timer.vi"("Time Setting"=w4113, "Action"=Elapsed_timer_control."Initialize") -> ()  [unwired: 6 in, 4 out]
        n191 = Bundle By Name(cluster=w4122, "Time up flag"=FALSE, "SET TIME TO CHECK"=w4113) -> (w4120:T3)
      }
      frame "SET TIMER 4" {
        w4129 = 4.0 ("Time Setting")
        # ">>State Logic  >>"
        # ">>> Time cluster >>>"
        # ">>> Yaw >>>"
        # ">>> Stepper position >>>"
        # ">>> Encoders >>>"
        # ">>> Object detection >>>"
        # ">>> Ultrasonic Sensors Detect >>>"
        n192 = call "Elasped Timer.vi"("Time Setting"=w4129, "Action"=Elapsed_timer_control."Initialize") -> ()  [unwired: 6 in, 4 out]
        n193 = Wait (ms)(milliseconds to wait=u32 250) -> ()  [unwired: 1 out]
        n194 = Bundle By Name(cluster=w4138, "Time up flag"=FALSE, "SET TIME TO CHECK"=w4129) -> (w4136:T3)
      }
      frame "SET TIMER 5" {
        w4146 = 5.0 ("Time Setting")
        # ">>State Logic  >>"
        # ">>> Time cluster >>>"
        # ">>> Yaw >>>"
        # ">>> Stepper position >>>"
        # ">>> Encoders >>>"
        # ">>> Object detection >>>"
        # ">>> Ultrasonic Sensors Detect >>>"
        n195 = call "Elasped Timer.vi"("Time Setting"=w4146, "Action"=Elapsed_timer_control."Initialize") -> ("Time Out?!"=w4145:bool)  [unwired: 6 in, 3 out]
        n196 = Wait (ms)(milliseconds to wait=u32 250) -> ()  [unwired: 1 out]
        n197 = Bundle By Name(cluster=w4154, "Time up flag"=w4145, "SET TIME TO CHECK"=w4146) -> (w4153:T3)
      }
      frame "START TIMER" {
        # ">>State Logic  >>"
        # ">>> Time cluster >>>"
        # ">>> Yaw >>>"
        # ">>> Stepper position >>>"
        # ">>> Encoders >>>"
        # ">>> Object detection >>>"
        # ">>> Ultrasonic Sensors Detect >>>"
        n198 = call "Elasped Timer.vi"("Action"=Elapsed_timer_control."Start") -> ("Time Out?!"=w4165:bool)  [unwired: 7 in, 3 out]
        n199 = Bundle By Name(cluster=w4168, "Time up flag"=w4165) -> (w4167:T3)
      }
      frame "-----MISC-----" {
        # ">>> Box Colour Detection >>>"
        # ">>> Line Sensor Cluster>>>"
        # ">>> IR Sensors >>>"
        # ">>> Time cluster >>>"
        # ">>> Object detection >>>"
        # ">>> Yaw >>>"
        # ">>> Ultrasonic Sensors Detect >>>"
        # ">>> Encoders >>>"
        # ">>> Stepper position >>>"
      }
      frame "Task 9" {
        # ">>> Box Colour Detection >>>"
        # ">>> Line Sensor Cluster>>>"
        # ">>> IR Sensors >>>"
        # ">>> Time cluster >>>"
        # ">>> Object detection >>>"
        # ">>> Yaw >>>"
        # ">>> Ultrasonic Sensors Detect >>>"
        # ">>> Encoders >>>"
        # ">>> Stepper position >>>"
        n200 = call "Colour Processing Test Env.vi"() -> ("Colour scan time out?"=w4194:bool, "Colour output boolean cluster"=w4192:T44)  [unwired: 10 in]
        n201 = Unbundle By Name(w4192) -> ("Red"=w4186:bool, "Black"=w4187:bool, "Blue"=w4188:bool, "Yellow"=w4189:bool, "Green"=w4190:bool, "No recognizable coolour"=w4191:bool)
        n202 = Bundle By Name(cluster=w4196, "Red"=w4186, "Black"=w4187, "Blue"=w4188, "Yellow"=w4189, "Green"=w4190, "Unknown"=w4191, "Image processing done"=w4194) -> (w4195:T1)
      }
    }
    "State Logic" <- w252
    "Image Processing Error" <- w219
    n203 = local read "TASK ENABLE"() -> (w246:bool)
    n204 = Not(x=w246) -> (.not. x?=w245:bool)
    n205 = case shown="True" w253 {
      tunnel: w210 -> [w284 w338]
      tunnel: w260 -> [w280 w340]
      tunnel: [w284 w338] -> w265
      tunnel: [w280 w341] -> w264
      tunnel: w261 -> [_ w336]
      tunnel: w263 -> [_ w337]
      tunnel: w258 -> [w283 w343]
      tunnel: [w283 w343] -> w257
      tunnel: "STOP TASK" -> [_ w326]
      tunnel: w252 -> [w282 w342]
      tunnel: [w282 w339] -> w251
      tunnel: w248 -> [w281 w332]
      tunnel: [w281 w332] -> w247
      tunnel: w245 -> [_ w327]
      tunnel: [w279 w324] -> w244
      tunnel: w243 -> [w279 w323]
      tunnel: w241 -> [w278 w320]
      tunnel: [w278 w320] -> w240
      tunnel: w238 -> [w277 w316]
      tunnel: [w277 w316] -> w237
      tunnel: w235 -> [w276 w314]
      tunnel: [w276 w314] -> w234
      tunnel: w232 -> [w275 w312]
      tunnel: [w275 w312] -> w231
      tunnel: w230 -> [w274 w311]
      tunnel: [w274 w310] -> w229
      tunnel: [_ w308] -> w228
      tunnel: w226 -> [w273 w306]
      tunnel: [w273 w306] -> w225
      tunnel: w224 -> [w272 w305]
      tunnel: [w272 w304] -> w223
      tunnel: w221 -> [w271 w301]
      tunnel: [w271 w301] -> w220
      tunnel: [w270 w300] -> w218
      tunnel: w216 -> [w270 w299]
      tunnel: [_ w297] -> w215
      tunnel: [_ w296] -> w214
      tunnel: [_ w295] -> w213
      tunnel: w211 -> [w269 w294]
      tunnel: [w269 w294] -> w209
      tunnel: [_ w285] -> w208
      frame False {
        # ">>> Box Colour Detection >>>"
        # ">>> Line Sensor Cluster>>>"
        # ">> Item Selection Bias >>"
        # ">>State Logic Queue Reference >>"
        # ">>Action states Queue Reference >>"
        # ">>True Stop Next State >>"
        # ">>State Logic  >>"
        # ">>> IR Sensors >>>"
        # ">>> Line Sensor Cluster>>>"
        # ">>> Line Sensor Cluster>>>"
        # ">>> Motor control cluster >>>"
        # ">>> yStepper command>>>"
        # ">>> Motor control cluster >>>"
        # ">>> yStepper command>>>"
        # ">>> Motor control cluster >>>"
        # ">>> IR Sensors >>>"
        # ">>> IR Sensors >>>"
        # ">>> yStepper command>>>"
        # ">>> Time cluster >>>"
        # ">>> Yaw >>>"
        # ">>> Stepper position >>>"
        # ">>> Encoders >>>"
        # ">>> Object detection >>>"
        # ">>> Ultrasonic Sensors Detect >>>"
        # ">>> Time cluster >>>"
        # ">>> Yaw >>>"
        # ">>> Stepper position >>>"
        # ">>> Encoders >>>"
        # ">>> Object detection >>>"
        # ">>> Ultrasonic Sensors Detect >>>"
      }
      frame True {
        # ">>> Box colour cluster >>>"
        # ">>State Logic Queue Reference >>"
        # ">>> Box Colour Detection >>>"
        # ">> Item Selection Bias >>"
        # ">>> IR Sensors >>>"
        # ">>> Line Sensor Cluster>>>"
        # ">>> Line Sensor Cluster>>>"
        # ">>> Motor control cluster >>>"
        # ">>> yStepper command>>>"
        # ">>> IR Sensors >>>"
        # ">>> Motor control cluster >>>"
        # ">>State Logic Queue Reference >>"
        # ">>Timeout>>"
        # ">>> yStepper command>>>"
        # ">>> Time cluster >>>"
        # ">>> Object detection >>>"
        # ">>> Yaw >>>"
        # ">>> Ultrasonic Sensors Detect >>>"
        # ">>> Encoders >>>"
        # ">>> Stepper position >>>"
        # ">>State Logic  >>"
        # ">>True Stop Next State >>"
        # ">>Action Queue>>"
        # ">> Manual override >>"
        # ">>> Time cluster >>>"
        # ">>> Yaw >>>"
        # ">>> Stepper position >>>"
        # ">>> Encoders >>>"
        # ">>> Object detection >>>"
        # ">>> Ultrasonic Sensors Detect >>>"
        # ">>Action Queue>>"
        # ">>State Logic Queue Reference >>"
        n206 = Or(x=w326, y=w327) -> (x .or. y?=w325:bool)
        n207 = Unbundle By Name(w294) -> ("Red"=w293:bool, "Black"=w292:bool, "Blue"=w291:bool, "Yellow"=w290:bool, "Green"=w289:bool, "Unknown"=w288:bool, "Image processing done"=w287:bool, "Colour"=w286:T2)
        n208 = Unbundle By Name(w301) -> ("Line Detected?"=w302:bool)
        n209 = Unbundle By Name(w306) -> ("Left IR Sensor"=w307:dbl, "Arm IR Sensor"=w303:dbl, "Bottom IR Sensor"=w298:dbl)
        n210 = Unbundle By Name(w312) -> ("Time up flag"=w313:bool)
        n211 = Unbundle By Name(w314) -> ("Yaw"=w315:dbl, "Compass"=w309:dbl)
        n212 = Unbundle By Name(w316) -> ("y Stepper Position"=w318:u8, "z Stepper Position"=w317:u8)
        n213 = Unbundle By Name(w332) -> ("xDistance"=w329:dbl, "yDistance"=w330:dbl, "wDistance"=w331:dbl)
        n214 = Unbundle By Name(w320) -> ("Recognized Object"=w319:bool, "Object X coordinate"=w322:dbl, "Object Y coordinate"=w321:dbl)
        n215 = Unbundle By Name(w343) -> ("PING_A"=w335:u8, "PING_B"=w334:u8, "PING_C"=w333:u8, "PING_D"=w328:u8)
        n216 = case shown="\"Task 8E: ROBOT ADJUST\"" w342 {
          tunnel: [w348 w360 w374 w385 w495 w512 w558 w596 w650 w692 w741 w784 w839 w887 w931 w991 w1032 w1075 w1124 w1167 w1220 w1258 w1310 w1356 w1402 w1443 w1492 w1536 w1582 w1623 w1672 w1716 w1762 w1803 w1852 w1896 w1942 w1983 w2032 w2067 w2085 w2133 w2174 w2224 w2280 w2319 w2368 w2411 w2464 w2502 w2554 w2591 w2639 w2682 w2732 w2776 w2824 w2880 w2921 w2973 w3021 w3066 w3110 w3158 w3209 w3252] -> w341
          tunnel: w340 -> [w348 w363 w375 w388 w497 w513 w559 w605 w648 w696 w742 w790 w832 w890 w938 w981 w1035 w1081 w1123 w1170 w1210 w1264 w1300 w1351 w1394 w1442 w1491 w1535 w1574 w1622 w1671 w1715 w1754 w1802 w1851 w1895 w1934 w1982 w2031 w2067 w2075 w2136 w2180 w2223 w2279 w2325 w2367 w2414 w2454 w2508 w2544 w2595 w2646 w2687 w2737 w2781 w2825 w2878 w2922 w2974 w3023 w3072 w3117 w3163 w3208 w3248]
          tunnel: [State_Type_Definitions,_for_0.26g_versions_and_later_3."Idle" ("Enum") State_Type_Definitions,_for_0.26g_versions_and_later_3."Idle" ("Enum") w370 w387 State_Type_Definitions,_for_0.26g_versions_and_later_3."Shutdown" ("Enum") w514 w560 w603 w651 w693 w740 w785 w838 w888 w933 w990 w1033 w1082 w1125 w1169 w1219 w1265 w1309 w1357 w1395 w1444 w1493 w1537 w1575 w1624 w1673 w1717 w1755 w1804 w1853 w1897 w1935 w1984 w2033 State_Type_Definitions,_for_0.26g_versions_and_later_3."Idle" ("Enum") w2084 w2134 w2181 w2225 w2281 w2326 w2369 w2413 w2463 w2509 w2553 w2592 w2640 w2683 w2733 w2777 w2823 w2881 w2920 w2972 w3022 w3065 w3112 w3164 w3210 w3251] -> w339
          tunnel: w338 -> [_ _ w373 w391 _ w518 w565 w599 w647 w697 w748 w789 w836 w891 w937 w988 w1030 w1080 w1121 w1171 w1217 w1263 w1307 w1354 w1401 w1440 w1489 w1533 w1581 w1620 w1669 w1713 w1761 w1800 w1849 w1893 w1941 w1980 w2029 _ w2082 w2131 w2179 w2221 w2277 w2324 w2365 w2415 w2461 w2507 w2551 w2599 w2645 w2690 w2740 w2784 w2833 w2877 w2923 w2967 w3024 w3071 w3116 w3162 w3207 w3257]
          tunnel: w337 -> [_ _ _ w390 _ w517 w564 w598 w646 w698 w747 w788 w835 w884 w936 w987 w1029 w1079 w1120 w1172 w1216 w1262 w1306 w1353 w1399 w1439 w1488 w1532 w1579 w1619 w1668 w1712 w1759 w1799 w1848 w1892 w1939 w1979 w2028 _ w2081 w2130 w2178 w2220 w2276 w2323 w2364 w2416 w2460 w2506 w2550 w2594 w2644 w2689 w2739 w2783 w2831 w2876 w2924 w2968 w3025 w3070 w3115 w3161 w3206 w3256]
          tunnel: w336 -> [_ _ w372 w386 _ w516 w563 w597 w645 w699 w746 w787 w834 w883 w935 w989 w1031 w1078 w1119 w1173 w1218 w1261 w1308 w1352 w1400 w1438 w1487 w1531 w1580 w1618 w1667 w1711 w1760 w1798 w1847 w1891 w1940 w1978 w2027 _ w2083 w2132 w2177 w2219 w2275 w2322 w2363 w2417 w2462 w2505 w2552 w2598 w2643 w2688 w2738 w2782 w2832 w2875 w2925 w2969 w3026 w3069 w3114 w3160 w3205 w3255]
          tunnel: w325 -> [_ _ _ _ _ w503 w557 w604 w644 w700 w743 w783 w837 w889 w939 w982 w1036 w1076 w1122 w1174 w1211 w1259 w1301 w1355 w1397 w1441 w1490 w1534 w1577 w1621 w1670 w1714 w1757 w1801 w1850 w1894 w1937 w1981 w2030 _ w2076 w2137 w2175 w2222 w2278 w2320 w2366 w2418 w2455 w2503 w2545 w2597 w2638 w2686 w2736 w2780 w2827 w2874 w2926 w2970 w3027 w3068 w3113 w3159 w3204 w3254]
          tunnel: w335 -> [_ _ _ _ _ _ _ _ _ _ _ _ _ _ _ _ _ _ _ _ _ _ _ _ _ _ _ _ _ _ _ _ _ _ _ _ _ _ _ _ _ _ _ _ _ _ _ _ _ _ _ _ _ _ _ _ _ _ _ _ _ _ _ _ _ _]
          tunnel: w334 -> [_ _ _ _ _ _ _ _ w643 _ _ _ w828 w872 w929 _ _ _ _ _ _ _ _ _ _ _ _ _ _ _ _ _ _ _ _ _ _ _ _ _ _ w2123 _ _ _ _ _ _ _ _ _ _ _ _ _ _ _ _ _ _ _ _ _ _ _ _]
          tunnel: w333 -> [_ _ _ _ _ _ _ _ w642 _ _ _ w829 w873 w930 _ _ _ _ _ _ _ _ _ _ _ _ _ _ _ _ _ _ _ _ _ _ _ _ _ _ w2124 _ _ _ _ _ _ _ _ _ _ _ _ _ _ _ _ _ _ _ _ _ _ _ _]
          tunnel: w331 -> [_ _ _ _ _ _ _ _ _ _ w745 _ _ _ _ _ _ _ _ _ _ _ _ _ _ _ _ _ _ _ _ _ _ _ _ _ _ _ _ _ _ _ _ _ _ _ _ _ _ _ _ _ _ _ _ _ _ _ _ w2966 _ _ _ _ _ _]
          tunnel: w330 -> [_ _ _ _ _ w511 w556 _ _ w691 _ _ _ _ w934 _ _ _ _ _ _ _ _ _ _ _ _ _ _ _ _ _ _ _ w1840 _ _ _ w2020 _ _ _ _ _ _ _ _ _ _ _ _ _ _ _ _ _ _ _ _ _ _ _ _ _ _ _]
          tunnel: w329 -> [_ _ _ _ _ _ _ _ _ _ _ _ _ w878 _ _ _ _ _ _ _ _ _ _ _ _ w1480 _ _ _ w1660 _ _ _ _ _ _ _ _ _ _ _ _ _ w2266 _ _ _ _ _ _ _ _ _ _ _ _ w2867 _ _ _ _ _ _ _ _]
          tunnel: w328 -> [_ _ _ _ _ _ _ _ _ _ _ _ _ _ _ _ _ _ _ _ _ _ _ _ _ _ _ _ _ _ _ _ _ _ _ _ _ _ _ _ _ _ _ _ _ _ _ _ _ _ _ _ _ _ _ _ _ _ _ _ _ _ _ _ _ _]
          tunnel: [State_Type_Definitions,_for_0.26g_versions_and_later_3."Idle" ("Enum") State_Type_Definitions,_for_0.26g_versions_and_later_3."Idle" ("Enum") State_Type_Definitions,_for_0.26g_versions_and_later_3."Idle" ("Enum") State_Type_Definitions,_for_0.26g_versions_and_later_3."Idle" ("Enum") State_Type_Definitions,_for_0.26g_versions_and_later_3."Shutdown" ("Enum") w509 w554 w602 w649 w694 w737 w782 w831 w886 w932 w992 w1034 w1074 w1126 w1168 w1221 w1257 w1311 w1358 w1396 w1445 w1494 w1538 w1576 w1625 w1674 w1718 w1756 w1805 w1854 w1898 w1936 w1985 w2034 w2069 w2086 w2135 w2173 w2226 w2282 w2318 w2370 w2412 w2465 w2501 w2555 w2593 w2641 w2685 w2735 w2779 w2822 w2879 w2919 w2971 w3020 w3064 w3111 w3165 w3211 w3250] -> w324
          tunnel: w323 -> [_ _ w370 _ _ _ _ _ _ _ _ _ _ _ _ _ _ _ _ _ _ _ _ _ _ _ _ _ _ _ _ _ _ _ _ _ _ _ _ w2069 _ _ _ _ _ _ _ _ _ _ _ _ _ _ _ _ _ _ _ _ _ _ _ _ _ _]
          tunnel: w319 -> [_ _ _ _ _ _ _ _ _ _ _ _ _ _ _ _ _ _ _ _ _ _ _ _ _ w1432 _ _ _ w1612 _ _ _ w1792 _ _ _ w1972 _ _ _ _ _ w2214 _ _ _ _ _ _ _ _ _ _ _ _ _ _ _ _ _ _ _ _ _ _]
          tunnel: w322 -> [_ _ _ _ _ _ _ _ _ _ _ _ _ _ _ _ _ _ _ _ _ _ _ _ _ _ _ _ _ _ _ _ _ _ _ _ _ _ _ _ _ _ _ _ w2272 _ _ _ _ _ _ _ _ _ _ _ _ _ _ _ _ _ _ _ _ _]
          tunnel: w321 -> [_ _ _ _ _ _ _ _ _ _ _ _ _ _ _ _ _ _ _ w1163 _ _ _ _ _ _ _ _ _ _ _ _ _ _ _ _ _ _ _ _ _ _ _ _ _ _ _ w2407 _ _ _ _ _ _ _ _ _ _ _ _ _ _ _ _ _ _]
          tunnel: w318 -> [_ _ _ _ _ _ _ _ _ _ _ _ _ _ _ _ _ _ _ w1162 _ _ _ _ _ _ _ _ _ _ _ _ _ _ _ _ _ _ _ _ _ _ _ _ _ _ _ w2406 _ _ _ _ _ _ _ _ _ _ _ _ _ _ _ _ _ _]
          tunnel: w317 -> [_ _ _ _ _ _ _ w601 _ _ _ w780 _ _ _ w985 _ w1070 _ _ w1214 _ w1304 w1350 _ _ _ _ _ _ _ _ _ _ _ _ _ _ _ _ w2079 _ _ _ _ _ _ _ w2458 _ w2548 w2596 _ _ _ _ _ _ _ _ _ _ _ _ _ _]
          tunnel: w315 -> [_ _ _ _ _ _ _ _ _ _ _ _ _ _ _ _ _ _ _ _ _ _ _ _ _ _ _ _ _ _ _ _ _ _ _ _ _ _ _ _ _ _ _ _ _ _ _ _ _ _ _ _ _ _ _ _ _ _ _ _ _ _ _ _ _ _]
          tunnel: w313 -> [_ _ _ _ _ _ _ _ _ _ _ _ _ _ _ _ _ _ w1116 _ _ w1255 _ _ w1390 w1433 _ _ w1570 w1613 _ _ w1750 w1793 _ _ w1930 w1973 _ _ _ _ w2171 w2213 _ w2316 w2360 _ _ w2499 _ _ _ _ _ _ _ _ _ _ _ _ _ _ _ _]
          tunnel: w311 -> [w346 w358 w369 w383 w493 w508 w553 w600 w641 w695 w736 w781 w830 w882 w928 w980 w1027 w1073 w1117 w1165 w1209 w1256 w1299 w1348 w1393 w1436 w1485 w1529 w1573 w1616 w1665 w1709 w1753 w1796 w1845 w1889 w1933 w1976 w2025 w2070 w2074 w2128 w2172 w2217 w2273 w2317 w2361 w2409 w2453 w2500 w2543 w2590 w2642 w2684 w2734 w2778 w2830 w2873 w2928 w2976 w3029 w3076 w3119 w3167 w3213 w3262]
          tunnel: [w346 w357 w369 w383 w493 w508 w553 w600 w641 w695 w736 w781 w830 w882 w928 w980 w1027 w1073 w1117 w1164 w1209 w1256 w1299 w1348 w1393 w1436 w1485 w1529 w1573 w1616 w1665 w1709 w1753 w1796 w1845 w1889 w1933 w1976 w2025 w2070 w2074 w2128 w2172 w2217 w2273 w2317 w2361 w2408 w2453 w2500 w2543 w2590 w2642 w2684 w2734 w2778 w2830 w2873 w2928 w2976 w3029 w3076 w3119 w3167 w3213 w3262] -> w310
          tunnel: w309 -> [_ _ _ _ _ _ _ _ _ _ _ _ _ _ _ _ _ _ _ _ _ _ _ _ _ _ _ _ _ _ _ _ _ _ _ _ _ _ _ _ _ _ _ _ _ _ _ _ _ _ _ _ w2637 _ _ _ _ _ _ _ _ _ _ _ _ _]
          tunnel: [_ _ _ TRUE _ w502 w550 w593 w638 w687 w733 w776 _ _ _ _ _ _ _ _ _ _ _ w1344 _ w1433 _ _ _ w1613 _ _ _ w1793 _ _ _ w1973 _ _ _ _ _ w2213 w2261 _ _ _ _ _ _ w2587 w2632 w2679 w2723 w2773 w2817 w2866 w2914 w2964 w3011 _ _ _ w3203 w3247] -> w308
          tunnel: w307 -> [_ _ _ _ _ _ _ _ _ _ _ _ _ _ _ _ _ _ _ _ _ _ _ _ _ _ _ _ _ _ _ _ _ _ _ _ _ _ _ _ _ _ _ _ _ _ _ _ _ _ _ _ _ _ _ _ _ _ _ _ _ w3063 _ _ _ _]
          tunnel: w305 -> [w345 w355 w368 w381 w492 w507 w552 w595 w640 w689 w735 w778 w823 w871 w927 w979 w1026 w1072 w1115 w1159 w1208 w1254 w1298 w1347 w1392 w1435 w1484 w1528 w1572 w1615 w1664 w1708 w1752 w1795 w1844 w1888 w1932 w1975 w2024 w2071 w2073 w2122 w2170 w2216 w2269 w2315 w2359 w2403 w2452 w2498 w2542 w2589 w2634 w2681 w2731 w2775 w2829 w2872 w2930 w2978 w3031 w3077 w3121 w3169 w3215 w3263]
          tunnel: [w345 w354 w368 w381 w492 w507 w552 w595 w640 w689 w735 w778 w823 w871 w927 w979 w1026 w1072 w1115 w1159 w1208 w1254 w1298 w1347 w1392 w1435 w1484 w1528 w1572 w1615 w1664 w1708 w1752 w1795 w1844 w1888 w1932 w1975 w2024 w2071 w2073 w2122 w2170 w2216 w2268 w2315 w2359 w2403 w2452 w2498 w2542 w2589 w2634 w2681 w2731 w2775 w2829 w2872 w2930 w2978 w3031 w3077 w3121 w3169 w3215 w3263] -> w304
          tunnel: w303 -> [_ _ _ _ _ _ _ _ _ _ _ _ _ _ _ _ _ _ _ _ _ _ _ _ _ _ _ _ _ _ _ _ _ _ _ _ _ _ _ _ _ _ _ _ _ _ _ _ _ _ _ _ _ _ w2729 _ _ _ _ _ w3018 _ _ _ _ _]
          tunnel: w302 -> [_ _ _ _ _ w504 _ _ _ _ _ _ _ _ w925 _ _ _ _ _ _ _ _ _ _ _ _ _ _ _ _ _ _ _ _ _ _ _ _ _ _ _ _ _ _ _ _ _ _ _ _ _ _ w2679 _ w2773 _ w2868 _ _ _ _ w3109 _ w3203 _]
          tunnel: [w344 w350 w367 w380 w491 w506 w551 w594 w639 w688 w734 w777 w822 w870 w926 w978 w1025 w1071 w1114 w1158 w1207 w1253 w1297 w1346 enum16{"Ball", "Soap", "Gel", "Pipe", "None"}."Ball" ("Object recognition mode") w1434 w1483 enum16{"Ball", "Soap", "Gel", "Pipe", "None"}."Soap" ("Object recognition mode") enum16{"Ball", "Soap", "Gel", "Pipe", "None"}."Soap" ("Object recognition mode") w1614 w1663 enum16{"Ball", "Soap", "Gel", "Pipe", "None"}."Gel" ("Object recognition mode") enum16{"Ball", "Soap", "Gel", "Pipe", "None"}."Gel" ("Object recognition mode") w1794 w1843 enum16{"Ball", "Soap", "Gel", "Pipe", "None"}."Pipe" ("Object recognition mode") enum16{"Ball", "Soap", "Gel", "Pipe", "None"}."Pipe" ("Object recognition mode") w1974 w2023 w2066 w2072 w2121 w2169 w2215 w2262 w2314 w2358 w2402 w2451 w2497 w2541 w2588 w2633 w2680 w2728 w2774 w2828 w2871 w2929 w2977 w3030 w3067 w3120 w3168 w3214 w3253] -> w300
          tunnel: w299 -> [w344 w350 w367 _ w491 w506 w551 w594 w639 w688 w734 w777 w822 w870 w926 w978 w1025 w1071 w1114 w1158 w1207 w1253 w1297 w1346 _ w1434 w1483 _ _ w1614 w1663 _ _ w1794 w1843 _ _ w1974 w2023 w2066 w2072 w2121 w2169 w2215 w2262 w2314 w2358 w2402 w2451 w2497 w2541 w2588 w2633 w2680 w2728 w2774 w2828 w2871 w2929 w2977 w3030 w3067 w3120 w3168 w3214 w3253]
          tunnel: w298 -> [_ _ _ _ _ _ _ _ _ _ _ _ _ _ _ _ _ _ _ _ _ _ _ _ _ _ _ _ _ _ _ _ _ _ _ _ _ _ _ _ _ w2120 _ _ _ _ _ _ _ _ _ _ _ _ w2727 _ _ _ _ _ w3012 _ _ _ _ _]
          tunnel: [_ _ _ _ _ _ _ _ w638 _ _ _ _ _ _ _ _ _ _ _ _ _ _ _ _ _ _ _ _ _ _ _ _ _ _ _ _ _ _ _ _ _ _ _ _ _ _ _ _ _ _ _ _ _ _ _ _ _ _ _ _ _ _ _ _ _] -> w297
          tunnel: [_ _ _ _ _ _ _ _ _ _ _ _ _ _ _ _ _ _ _ _ _ _ _ _ _ _ _ _ _ _ _ _ _ _ _ _ _ _ _ _ _ _ _ _ _ _ _ _ _ _ _ _ _ _ w2725 _ _ _ _ _ w3010 _ _ _ _ _] -> w296
          tunnel: [_ _ _ _ _ _ _ _ _ _ _ _ _ _ _ _ _ _ _ _ _ _ _ _ _ _ _ _ _ _ _ _ _ _ _ _ _ _ _ _ _ _ _ _ _ _ _ _ _ _ _ _ _ _ w2724 _ _ _ _ _ w3010 _ _ _ _ _] -> w295
          tunnel: w293 -> [_ _ _ _ _ _ _ _ _ _ _ _ _ _ _ _ _ _ _ _ _ _ _ _ _ _ _ _ _ _ _ _ _ _ _ _ _ _ _ _ _ _ _ _ _ _ _ _ _ _ _ _ _ _ _ _ _ _ _ _ _ _ _ _ _ _]
          tunnel: w292 -> [_ _ _ _ _ _ _ _ _ _ _ _ _ _ _ _ _ _ _ _ _ _ _ _ _ _ _ _ _ _ _ _ _ _ _ _ _ _ _ _ _ _ _ _ _ _ _ _ _ _ _ _ _ _ _ _ _ _ _ _ _ _ _ _ _ _]
          tunnel: w291 -> [_ _ _ _ _ _ _ _ _ _ _ _ _ _ _ _ _ _ _ _ _ _ _ _ _ _ _ _ _ _ _ _ _ _ _ _ _ _ _ _ _ _ _ _ _ _ _ _ _ _ _ _ _ _ _ _ _ _ _ _ _ _ _ _ _ _]
          tunnel: w290 -> [_ _ _ _ _ _ _ _ _ _ _ _ _ _ _ _ _ _ _ _ _ _ _ _ _ _ _ _ _ _ _ _ _ _ _ _ _ _ _ _ _ _ _ _ _ _ _ _ _ _ _ _ _ _ _ _ _ _ _ _ _ _ _ _ _ _]
          tunnel: w289 -> [_ _ _ _ _ _ _ _ _ _ _ _ _ _ _ _ _ _ _ _ _ _ _ _ _ _ _ _ _ _ _ _ _ _ _ _ _ _ _ _ _ _ _ _ _ _ _ _ _ _ _ _ _ _ _ _ _ _ _ _ _ _ _ _ _ _]
          tunnel: w288 -> [_ _ _ _ _ _ _ _ _ _ _ _ _ _ _ _ _ _ _ _ _ _ _ _ _ _ _ _ _ _ _ _ _ _ _ _ _ _ _ _ _ _ _ _ _ _ _ _ _ _ _ _ _ _ _ _ _ _ _ _ _ _ _ _ _ _]
          tunnel: w287 -> [_ _ _ _ _ _ _ _ _ _ _ _ _ _ _ _ _ _ _ _ _ _ _ _ _ _ _ _ _ _ _ _ _ _ _ _ _ _ _ _ _ _ _ _ _ _ _ _ _ _ _ _ _ _ _ _ w2817 _ w2914 _ _ _ _ w3153 _ w3247]
          tunnel: w286 -> [_ _ _ _ _ _ _ _ _ _ _ _ _ _ _ _ _ _ _ _ _ _ _ _ _ _ _ _ _ _ _ _ _ _ _ _ _ _ _ _ _ _ _ _ _ _ _ _ _ _ _ _ _ _ _ _ w2820 _ w2916 _ _ _ _ w3155 _ w3249]
          tunnel: [_ _ _ _ _ _ _ _ _ _ _ _ _ _ _ _ _ _ _ _ _ _ _ _ _ _ _ _ _ _ _ _ _ _ _ _ _ _ _ _ _ _ _ _ _ _ _ _ _ _ _ _ _ _ _ _ w2818 _ w2915 _ _ _ _ _ _ _] -> w285
          frame "None" {
            # ">>> Motor control cluster >>>"
            # ">>> yStepper command>>>"
          }
          frame "Startup" {
            # ">>> yStepper command>>>"
            n217 = for {
              shift-right: [w366] -> w360
              shift-left: w363 -> [w365]
              tunnel: string[] ["INIT", "RESET ARM", "RESET FLAGS", "RESET YAW", "NAVX CALIBRATE"] -> [w364] mode=indexing
              n218 = Enqueue Element(queue=w365, element=w364) -> (queue out=w366:refnum<queue>)  [unwired: 2 in, 2 out]
            }
            n219 = Bundle By Name(cluster=w358, "yStepper desired"=u8 0) -> (w357:T20)
            n220 = Bundle By Name(cluster=w355, "ySpeed"=0.0, "xSpeed"=0.0, "wSpeed"=0.0) -> (w354:T19)
          }
          frame "True Stop" {
            # ">>Action Queue>>"
            # ">>> Motor control cluster >>>"
            # ">>> yStepper command>>>"
            n221 = Flush Queue(queue=w373, error in (no error)=w372) -> ()  [unwired: 3 out]
            n222 = for {
              shift-right: [w379] -> w374
              shift-left: w375 -> [w378]
              tunnel: string[] ["STOP", "RESET ENCODERS", "RESET YAW", "RESET ARM", "RESET ALL SENSORS", "DISPOSE CAM BUFFERS", "DISPOSE PROC BUFFERS", "CAM CLOSE", ""] -> [w377] mode=indexing
              n223 = Enqueue Element(queue=w378, element=w377) -> (queue out=w379:refnum<queue>)  [unwired: 2 in, 2 out]
            }
          }
          frame "Idle", Default {
            # ">>> Motor control cluster >>>"
            # ">>> yStepper command>>>"
            n224 = Dequeue Element(queue=w391, timeout in ms (-1)=w390, error in (no error)=w386) -> (element=w389:T10)  [unwired: 3 out]
            n225 = case shown="\"None\", Default" w389 {
              tunnel: [w394 w402 w410 w418 w426 w434 w442 w450 w458 w465 w475 w482 w485] -> w385
              tunnel: w388 -> [w395 w403 w411 w419 w427 w435 w443 w451 w459 w466 w474 w482 w486]
              tunnel: [State_Type_Definitions,_for_0.26g_versions_and_later_3."Task 1A" ("Enum") State_Type_Definitions,_for_0.26g_versions_and_later_3."Task 2:Raise Arm" ("Enum") State_Type_Definitions,_for_0.26g_versions_and_later_3."Task 3" ("Enum") State_Type_Definitions,_for_0.26g_versions_and_later_3."Task 4_A" ("Enum") State_Type_Definitions,_for_0.26g_versions_and_later_3."Task 5A: RAISING ARM" ("Enum") State_Type_Definitions,_for_0.26g_versions_and_later_3."Task 6A: RAISE ARM" ("Enum") State_Type_Definitions,_for_0.26g_versions_and_later_3."Task 8A: RAISE ARM" ("Enum") State_Type_Definitions,_for_0.26g_versions_and_later_3."Task 8A: RAISE ARM" ("Enum") State_Type_Definitions,_for_0.26g_versions_and_later_3."Task 8A: RAISE ARM" ("Enum") State_Type_Definitions,_for_0.26g_versions_and_later_3."Task 8A: RAISE ARM" ("Enum") State_Type_Definitions,_for_0.26g_versions_and_later_3."Task 9A: Raise Arm" ("Enum") State_Type_Definitions,_for_0.26g_versions_and_later_3."Idle" ("Enum") State_Type_Definitions,_for_0.26g_versions_and_later_3."Shutdown" ("Enum")] -> w387
              tunnel: [enum16{"Ball", "Soap", "Gel", "Pipe", "None"}."None" ("Object recognition mode") enum16{"Ball", "Soap", "Gel", "Pipe", "None"}."None" ("Object recognition mode") enum16{"Ball", "Soap", "Gel", "Pipe", "None"}."None" ("Object recognition mode") enum16{"Ball", "Soap", "Gel", "Pipe", "None"}."None" ("Object recognition mode") enum16{"Ball", "Soap", "Gel", "Pipe", "None"}."None" ("Object recognition mode") enum16{"Ball", "Soap", "Gel", "Pipe", "None"}."None" ("Object recognition mode") enum16{"Ball", "Soap", "Gel", "Pipe", "None"}."Ball" ("Object recognition mode") enum16{"Ball", "Soap", "Gel", "Pipe", "None"}."Gel" ("Object recognition mode") enum16{"Ball", "Soap", "Gel", "Pipe", "None"}."Pipe" ("Object recognition mode") enum16{"Ball", "Soap", "Gel", "Pipe", "None"}."Soap" ("Object recognition mode") enum16{"Ball", "Soap", "Gel", "Pipe", "None"}."None" ("Object recognition mode") enum16{"Ball", "Soap", "Gel", "Pipe", "None"}."None" ("Object recognition mode") enum16{"Ball", "Soap", "Gel", "Pipe", "None"}."None" ("Object recognition mode")] -> w380
              frame "Start Task 1" {
                n226 = for {
                  shift-right: [w399] -> w394
                  shift-left: w395 -> [w398]
                  tunnel: string[] ["RESET ENCODERS", "RESET YAW", "FORWARD", "READ ENCODERS"] -> [w397] mode=indexing
                  n227 = Enqueue Element(queue=w398, element=w397) -> (queue out=w399:refnum<queue>)  [unwired: 2 in, 2 out]
                }
              }
              frame "Start Task 2" {
                n228 = for {
                  shift-right: [w407] -> w402
                  shift-left: w403 -> [w406]
                  tunnel: string[] ["RESET ENCODERS", "RESET YAW", "READ ULTRASONIC", "ARDUINO - ULTRASONIC"] -> [w405] mode=indexing
                  n229 = Enqueue Element(queue=w406, element=w405) -> (queue out=w407:refnum<queue>)  [unwired: 2 in, 2 out]
                }
              }
              frame "Start Task 3" {
                n230 = for {
                  shift-right: [w415] -> w410
                  shift-left: w411 -> [w414]
                  tunnel: string[] ["RESET ENCODERS", "READ ENCODERS", "R-ACW"] -> [w413] mode=indexing
                  n231 = Enqueue Element(queue=w414, element=w413) -> (queue out=w415:refnum<queue>)  [unwired: 2 in, 2 out]
                }
              }
              frame "Start Task 4" {
                n232 = for {
                  shift-right: [w423] -> w418
                  shift-left: w419 -> [w422]
                  tunnel: string[] ["RESET YAW", "RESET ENCODERS", "RESET ARM", "RESET FLAGS", "", ""] -> [w421] mode=indexing
                  n233 = Enqueue Element(queue=w422, element=w421) -> (queue out=w423:refnum<queue>)  [unwired: 2 in, 2 out]
                }
              }
              frame "Start Task 5" {
                n234 = for {
                  shift-right: [w431] -> w426
                  shift-left: w427 -> [w430]
                  tunnel: string[] ["RESET YAW", "RESET ENCODERS", "RESET ARM", "RESET ALL SENSORS", "", ""] -> [w429] mode=indexing
                  n235 = Enqueue Element(queue=w430, element=w429) -> (queue out=w431:refnum<queue>)  [unwired: 2 in, 2 out]
                }
              }
              frame "Start Task 6" {
                n236 = for {
                  shift-right: [w439] -> w434
                  shift-left: w435 -> [w438]
                  tunnel: string[] ["OPEN LOG CAM ", "", "", "", "", ""] -> [w437] mode=indexing
                  n237 = Enqueue Element(queue=w438, element=w437) -> (queue out=w439:refnum<queue>)  [unwired: 2 in, 2 out]
                }
              }
              frame "Start Task 8 - BALL" {
                n238 = for {
                  shift-right: [w447] -> w442
                  shift-left: w443 -> [w446]
                  tunnel: string[] ["RESET YAW", "RESET ENCODERS", "RESET ARM", "RESET FLAGS"] -> [w445] mode=indexing
                  n239 = Enqueue Element(queue=w446, element=w445) -> (queue out=w447:refnum<queue>)  [unwired: 2 in, 2 out]
                }
              }
              frame "Start Task 8 - Gel" {
                n240 = for {
                  shift-right: [w455] -> w450
                  shift-left: w451 -> [w454]
                  tunnel: string[] ["RESET YAW", "RESET ENCODERS", "RESET ARM", "RESET FLAGS"] -> [w453] mode=indexing
                  n241 = Enqueue Element(queue=w454, element=w453) -> (queue out=w455:refnum<queue>)  [unwired: 2 in, 2 out]
                }
              }
              frame "Start Task 8 - Pipe" {
                n242 = for {
                  shift-right: [w463] -> w458
                  shift-left: w459 -> [w462]
                  tunnel: string[] ["RESET YAW", "RESET ENCODERS", "RESET ARM", "RESET FLAGS"] -> [w461] mode=indexing
                  n243 = Enqueue Element(queue=w462, element=w461) -> (queue out=w463:refnum<queue>)  [unwired: 2 in, 2 out]
                }
              }
              frame "Start Task 8 - Soap" {
                n244 = for {
                  shift-right: [w471] -> w465
                  shift-left: w466 -> [w470]
                  tunnel: string[] ["RESET YAW", "RESET ENCODERS", "RESET ARM", "RESET FLAGS"] -> [w469] mode=indexing
                  n245 = Enqueue Element(queue=w470, element=w469) -> (queue out=w471:refnum<queue>)  [unwired: 2 in, 2 out]
                }
              }
              frame "Start Task 9" {
                n246 = for {
                  shift-right: [w479] -> w475
                  shift-left: w474 -> [w478]
                  tunnel: string[] ["Z STEPPER BOX HEIGHT", "READ STEPPER VALUES", "", ""] -> [w477] mode=indexing
                  n247 = Enqueue Element(queue=w478, element=w477) -> (queue out=w479:refnum<queue>)  [unwired: 2 in, 2 out]
                }
              }
              frame "None", Default {
              }
              frame "Exit" {
                n248 = for {
                  shift-right: [w490] -> w485
                  shift-left: w486 -> [w489]
                  tunnel: string[] ["STOP", "RESET ENCODERS", "RESET YAW", "EXIT"] -> [w488] mode=indexing
                  n249 = Enqueue Element(queue=w489, element=w488) -> (queue out=w490:refnum<queue>)  [unwired: 2 in, 2 out]
                }
              }
            }
          }
          frame "Shutdown" {
            # ">> Item Selection Bias >>"
            # ">>> yStepper command>>>"
            n250 = for {
              shift-right: [w501] -> w495
              shift-left: w497 -> [w500]
              tunnel: string[] ["INIT", "RESET ENCODERS", "RESET FLAGS", "CAM CLOSE", "DISPOSE BUFFERS", "EXIT", ""] -> [w499] mode=indexing
              n251 = Enqueue Element(queue=w500, element=w499) -> (queue out=w501:refnum<queue>)  [unwired: 2 in, 2 out]
            }
          }
          frame "Task 1A" {
            # ">>> Motor control cluster >>>"
            # ">> Line detection >>"
            # ">> Checks if 1 metre moved >>"
            # ">>> yStepper command>>>"
            # "Use 250"
            n252 = Greater?(x=w511, y=265.0) -> (0:w505:bool)
            n253 = Dequeue Element(queue=w518, timeout in ms (-1)=w517, error in (no error)=w516) -> (element=w515:T10)  [unwired: 3 out]
            n254 = And(x=w504, y=w505) -> (x .and. y?=w502:bool)
            n255 = case shown="\"Start Task 1\", Default" w515 {
              tunnel: w503 -> [w519 _]
              tunnel: [w529 State_Type_Definitions,_for_0.26g_versions_and_later_3."True Stop" ("Enum")] -> w514
              tunnel: w513 -> [w527 w544]
              tunnel: [w526 w543] -> w512
              tunnel: [State_Type_Definitions,_for_0.26g_versions_and_later_3."Idle" ("Enum") State_Type_Definitions,_for_0.26g_versions_and_later_3."Shutdown" ("Enum")] -> w509
              tunnel: w502 -> [w520 _]
              frame "Start Task 1", Default {
                n256 = Or(x=w520, y=w519) -> (x .or. y?=w521:bool)
                n257 = case shown="True" w521 {
                  tunnel: w527 -> [w532 w538]
                  tunnel: [w531 w536] -> w526
                  frame False {
                    n258 = for {
                      shift-right: [w534] -> w531
                      shift-left: w532 -> [w535]
                      tunnel: string[] ["READ ENCODERS", "READ NAVX", "FORWARD", "READ LINE SENSOR"] ("element") -> [w533] mode=indexing
                      n259 = Enqueue Element(queue=w535, element=w533) -> (queue out=w534:refnum<queue>)  [unwired: 2 in, 2 out]
                    }
                  }
                  frame True {
                    n260 = for {
                      shift-right: [w540] -> w536
                      shift-left: w538 -> [w541]
                      tunnel: string[] ["RESET YAW", "RESET ENCODERS", "STOP", ""] -> [w539] mode=indexing
                      n261 = Enqueue Element(queue=w541, element=w539) -> (queue out=w540:refnum<queue>)  [unwired: 2 in, 2 out]
                    }
                  }
                }
                n262 = Select(t=State_Type_Definitions,_for_0.26g_versions_and_later_3."True Stop" ("Enum"), s=w519, f=State_Type_Definitions,_for_0.26g_versions_and_later_3."Task 1B" ("Enum")) -> (s? t:f=w524:T18)
                n263 = Select(t=w524, s=w520, f=State_Type_Definitions,_for_0.26g_versions_and_later_3."Task 1A" ("Enum")) -> (s? t:f=w529:T18)
              }
              frame "Exit" {
                n264 = for {
                  shift-right: [w548] -> w543
                  shift-left: w544 -> [w549]
                  tunnel: string[] ["STOP", "RESET ENCODERS", "RESET YAW", ""] -> [w547] mode=indexing
                  n265 = Enqueue Element(queue=w549, element=w547) -> (queue out=w548:refnum<queue>)  [unwired: 2 in, 2 out]
                }
              }
            }
          }
          frame "Task 1B" {
            # ">>> Motor control cluster >>>"
            # ">> Line detection >>"
            # ">> Adds small distance overhead after 1M >>"
            # ">>> yStepper command>>>"
            n266 = Greater?(x=w556, y=50.0) -> (0:w550:bool)
            n267 = Dequeue Element(queue=w565, timeout in ms (-1)=w564, error in (no error)=w563) -> (element=w562:T10)  [unwired: 3 out]
            n268 = Or(x=w550, y=w557) -> (x .or. y?=w561:bool)
            n269 = case shown="\"Start Task 1\", Default" w562 {
              tunnel: w561 -> [w568 _]
              tunnel: [w572 State_Type_Definitions,_for_0.26g_versions_and_later_3."True Stop" ("Enum")] -> w560
              tunnel: w559 -> [w569 w587]
              tunnel: [w567 w586] -> w558
              tunnel: [State_Type_Definitions,_for_0.26g_versions_and_later_3."Idle" ("Enum") State_Type_Definitions,_for_0.26g_versions_and_later_3."Shutdown" ("Enum")] -> w554
              frame "Start Task 1", Default {
                n270 = case shown="True" w568 {
                  tunnel: w569 -> [w575 w581]
                  tunnel: [w574 w579] -> w567
                  frame False {
                    n271 = for {
                      shift-right: [w577] -> w574
                      shift-left: w575 -> [w578]
                      tunnel: string[] ["READ ENCODERS", "READ NAVX", "FORWARD", "READ LINE SENSOR"] ("element") -> [w576] mode=indexing
                      n272 = Enqueue Element(queue=w578, element=w576) -> (queue out=w577:refnum<queue>)  [unwired: 2 in, 2 out]
                    }
                  }
                  frame True {
                    n273 = for {
                      shift-right: [w583] -> w579
                      shift-left: w581 -> [w584]
                      tunnel: string[] ["RESET YAW", "RESET ENCODERS", "STOP", ""] -> [w582] mode=indexing
                      n274 = Enqueue Element(queue=w584, element=w582) -> (queue out=w583:refnum<queue>)  [unwired: 2 in, 2 out]
                    }
                  }
                }
                n275 = Select(t=State_Type_Definitions,_for_0.26g_versions_and_later_3."True Stop" ("Enum"), s=w568, f=State_Type_Definitions,_for_0.26g_versions_and_later_3."Task 1B" ("Enum")) -> (s? t:f=w572:T18)
              }
              frame "Exit" {
                n276 = for {
                  shift-right: [w591] -> w586
                  shift-left: w587 -> [w592]
                  tunnel: string[] ["STOP", "RESET ENCODERS", "RESET YAW", ""] -> [w590] mode=indexing
                  n277 = Enqueue Element(queue=w592, element=w590) -> (queue out=w591:refnum<queue>)  [unwired: 2 in, 2 out]
                }
              }
            }
          }
          frame "Task 2:Raise Arm" {
            # ">> Stepper height reeached >>"
            # ">>> yStepper command>>>"
            # ">> Manual override >>"
            n278 = Dequeue Element(queue=w599, timeout in ms (-1)=w598, error in (no error)=w597) -> (element=w607:T10)  [unwired: 3 out]
            n279 = Equal?(x=w601, y=u8 60) -> (x = y?=w593:bool)
            n280 = case shown="\"Start Task 1\", Default" w607 {
              tunnel: [w618 State_Type_Definitions,_for_0.26g_versions_and_later_3."True Stop" ("Enum")] -> w603
              tunnel: [w616 w633] -> w596
              tunnel: w605 -> [w615 _]
              tunnel: w604 -> [w609 _]
              tunnel: [State_Type_Definitions,_for_0.26g_versions_and_later_3."Idle" ("Enum") State_Type_Definitions,_for_0.26g_versions_and_later_3."Shutdown" ("Enum")] -> w602
              tunnel: w593 -> [w608 _]
              frame "Start Task 1", Default {
                # ">> WIill proceed to part ii if not manual override >>"
                # ">>If ENABLE or Trigger is set to true>>"
                n281 = Or(x=w608, y=w609) -> (x .or. y?=w610:bool)
                n282 = case shown="True" w608 {
                  tunnel: [w621 w627] -> w616
                  tunnel: w615 -> [w620 w626]
                  frame False {
                    n283 = for {
                      shift-right: [w623] -> w621
                      shift-left: w620 -> [w624]
                      tunnel: string[] ["Z STEPPER CAM HEIGHT", "READ STEPPER VALUES"] ("element") -> [w622] mode=indexing
                      n284 = Enqueue Element(queue=w624, element=w622) -> (queue out=w623:refnum<queue>)  [unwired: 2 in, 2 out]
                    }
                  }
                  frame True {
                    n285 = for {
                      shift-right: [w629] -> w627
                      shift-left: w626 -> [w630]
                      tunnel: string[] ["ARDUINO - ULTRASONIC", "READ ULTRASONIC", "", "", "", ""] -> [w628] mode=indexing
                      n286 = Enqueue Element(queue=w630, element=w628) -> (queue out=w629:refnum<queue>)  [unwired: 2 in, 2 out]
                    }
                  }
                }
                n287 = Select(t=State_Type_Definitions,_for_0.26g_versions_and_later_3."True Stop" ("Enum"), s=w609, f=State_Type_Definitions,_for_0.26g_versions_and_later_3."Task 2:Sensor Mode" ("Enum")) -> (s? t:f=w612:T18)
                n288 = Select(t=w612, s=w610, f=State_Type_Definitions,_for_0.26g_versions_and_later_3."Task 2:Raise Arm" ("Enum")) -> (s? t:f=w618:T18)
              }
              frame "Exit" {
                n289 = for {
                  shift-right: [w636] -> w633
                  shift-left: _ -> [w637]
                  tunnel: string[] ["STOP", "RESET ENCODERS", "RESET YAW", ""] -> [w635] mode=indexing
                  n290 = Enqueue Element(queue=w637, element=w635) -> (queue out=w636:refnum<queue>)  [unwired: 2 in, 2 out]
                }
              }
            }
          }
          frame "Task 2:Sensor Mode" {
            w654 = u8 20 ("y")
            # ">>> yStepper command>>>"
            # ">>Object detected>>"
            n291 = Dequeue Element(queue=w647, timeout in ms (-1)=w646, error in (no error)=w645) -> (element=w655:T10)  [unwired: 3 out]
            n292 = Less?(x=w643, y=w654) -> (x < y?=w653:bool)
            n293 = Less?(x=w642, y=w654) -> (x < y?=w652:bool)
            n294 = Or(x=w653, y=w652) -> (x .or. y?=w638:bool)
            n295 = case shown="\"Start Task 1\", Default" w655 {
              tunnel: w638 -> [w658 _]
              tunnel: [w665 State_Type_Definitions,_for_0.26g_versions_and_later_3."True Stop" ("Enum")] -> w651
              tunnel: w644 -> [w657 _]
              tunnel: w648 -> [w664 w681]
              tunnel: [w663 w682] -> w650
              tunnel: [State_Type_Definitions,_for_0.26g_versions_and_later_3."Idle" ("Enum") State_Type_Definitions,_for_0.26g_versions_and_later_3."Shutdown" ("Enum")] -> w649
              frame "Start Task 1", Default {
                n296 = case shown="False" w658 {
                  tunnel: w664 -> [w668 w675]
                  tunnel: [w669 w674] -> w663
                  frame False {
                    n297 = for {
                      tunnel: string[] ["READ ULTRASONIC", "STOP"] ("element") -> [w670] mode=indexing
                      shift-right: [w672] -> w669
                      shift-left: w668 -> [w671]
                      n298 = Enqueue Element(queue=w671, element=w670) -> (queue out=w672:refnum<queue>)  [unwired: 2 in, 2 out]
                    }
                  }
                  frame True {
                    n299 = for {
                      shift-right: [w677] -> w674
                      shift-left: w675 -> [w678]
                      tunnel: string[] ["RESET ENCODERS", "READ NAVX", "READ ENCODERS"] -> [w676] mode=indexing
                      n300 = Enqueue Element(queue=w678, element=w676) -> (queue out=w677:refnum<queue>)  [unwired: 2 in, 2 out]
                    }
                  }
                }
                n301 = Or(x=w658, y=w657) -> (x .or. y?=w656:bool)
                n302 = Select(t=State_Type_Definitions,_for_0.26g_versions_and_later_3."True Stop" ("Enum"), s=w657, f=State_Type_Definitions,_for_0.26g_versions_and_later_3."Task 2:Reverse Mode" ("Enum")) -> (s? t:f=w659:T18)
                n303 = Select(t=w659, s=w656, f=State_Type_Definitions,_for_0.26g_versions_and_later_3."Task 2:Sensor Mode" ("Enum")) -> (s? t:f=w665:T18)
              }
              frame "Exit" {
                n304 = for {
                  shift-right: [w685] -> w682
                  shift-left: w681 -> [w686]
                  tunnel: string[] ["STOP", "RESET ENCODERS", "RESET YAW", "ARDUINO MODE 0"] -> [w684] mode=indexing
                  n305 = Enqueue Element(queue=w686, element=w684) -> (queue out=w685:refnum<queue>)  [unwired: 2 in, 2 out]
                }
              }
            }
          }
          frame "Task 2:Reverse Mode" {
            # ">>> yStepper command>>>"
            n306 = Dequeue Element(queue=w697, timeout in ms (-1)=w698, error in (no error)=w699) -> (element=w701:T10)  [unwired: 3 out]
            n307 = Less?(x=w691, y=-30.0) -> (x < y?=w687:bool)
            n308 = case shown="\"Start Task 1\", Default" w701 {
              tunnel: [w711 State_Type_Definitions,_for_0.26g_versions_and_later_3."True Stop" ("Enum")] -> w693
              tunnel: w700 -> [w704 _]
              tunnel: w696 -> [w710 w727]
              tunnel: [w709 w728] -> w692
              tunnel: [State_Type_Definitions,_for_0.26g_versions_and_later_3."Idle" ("Enum") State_Type_Definitions,_for_0.26g_versions_and_later_3."Shutdown" ("Enum")] -> w694
              tunnel: w687 -> [w702 _]
              frame "Start Task 1", Default {
                n309 = case shown="True" w702 {
                  tunnel: w710 -> [w714 w721]
                  tunnel: [w715 w720] -> w709
                  frame False {
                    n310 = for {
                      tunnel: string[] ["READ ENCODERS", "REVERSE", "READ NAVX"] ("element") -> [w716] mode=indexing
                      shift-right: [w718] -> w715
                      shift-left: w714 -> [w717]
                      n311 = Enqueue Element(queue=w717, element=w716) -> (queue out=w718:refnum<queue>)  [unwired: 2 in, 2 out]
                    }
                  }
                  frame True {
                    n312 = for {
                      shift-right: [w723] -> w720
                      shift-left: w721 -> [w724]
                      tunnel: string[] ["STOP", "ARDUINO - ULTRASONIC", "READ ULTRASONIC", "RESET ENCODERS"] -> [w722] mode=indexing
                      n313 = Enqueue Element(queue=w724, element=w722) -> (queue out=w723:refnum<queue>)  [unwired: 2 in, 2 out]
                    }
                  }
                }
                n314 = Or(x=w702, y=w704) -> (x .or. y?=w703:bool)
                n315 = Select(t=State_Type_Definitions,_for_0.26g_versions_and_later_3."True Stop" ("Enum"), s=w704, f=State_Type_Definitions,_for_0.26g_versions_and_later_3."Task 2:Sensor Mode" ("Enum")) -> (s? t:f=w705:T18)
                n316 = Select(t=w705, s=w703, f=State_Type_Definitions,_for_0.26g_versions_and_later_3."Task 2:Reverse Mode" ("Enum")) -> (s? t:f=w711:T18)
              }
              frame "Exit" {
                n317 = for {
                  shift-right: [w731] -> w728
                  shift-left: w727 -> [w732]
                  tunnel: string[] ["STOP", "RESET ENCODERS", "RESET YAW", "ARDUINO MODE 0"] -> [w730] mode=indexing
                  n318 = Enqueue Element(queue=w732, element=w730) -> (queue out=w731:refnum<queue>)  [unwired: 2 in, 2 out]
                }
              }
            }
          }
          frame "Task 3" {
            # ">>> Motor control cluster >>>"
            # ">>> yStepper command>>>"
            n319 = Dequeue Element(queue=w748, timeout in ms (-1)=w747, error in (no error)=w746) -> (element=w738:T10)  [unwired: 3 out]
            n320 = Less?(x=w745, y=-160.0) -> (x < y?=w733:bool)
            n321 = Or(x=w733, y=w743) -> (x .or. y?=w739:bool)
            n322 = case shown="\"Start Task 1\", Default" w738 {
              tunnel: w739 -> [w751 _]
              tunnel: [w755 State_Type_Definitions,_for_0.26g_versions_and_later_3."True Stop" ("Enum")] -> w740
              tunnel: w742 -> [w752 w771]
              tunnel: [w750 w770] -> w741
              tunnel: [State_Type_Definitions,_for_0.26g_versions_and_later_3."Idle" ("Enum") State_Type_Definitions,_for_0.26g_versions_and_later_3."Shutdown" ("Enum")] -> w737
              frame "Start Task 1", Default {
                n323 = case shown="False" w751 {
                  tunnel: w752 -> [w758 w764]
                  tunnel: [w757 w762] -> w750
                  frame False {
                    n324 = for {
                      shift-right: [w760] -> w757
                      shift-left: w758 -> [w761]
                      tunnel: string[] ["READ ENCODERS", "R-CW"] ("element") -> [w759] mode=indexing
                      n325 = Enqueue Element(queue=w761, element=w759) -> (queue out=w760:refnum<queue>)  [unwired: 2 in, 2 out]
                    }
                  }
                  frame True {
                    n326 = for {
                      shift-right: [w766] -> w762
                      shift-left: w764 -> [w767]
                      tunnel: string[] ["RESET YAW", "RESET ENCODERS", "STOP", "ARDUINO MODE 0"] -> [w765] mode=indexing
                      n327 = Enqueue Element(queue=w767, element=w765) -> (queue out=w766:refnum<queue>)  [unwired: 2 in, 2 out]
                    }
                  }
                }
                n328 = Select(t=State_Type_Definitions,_for_0.26g_versions_and_later_3."True Stop" ("Enum"), s=w751, f=State_Type_Definitions,_for_0.26g_versions_and_later_3."Task 3" ("Enum")) -> (s? t:f=w755:T18)
              }
              frame "Exit" {
                n329 = for {
                  shift-right: [w774] -> w770
                  shift-left: w771 -> [w775]
                  tunnel: string[] ["STOP", "RESET ENCODERS", "RESET YAW", ""] -> [w773] mode=indexing
                  n330 = Enqueue Element(queue=w775, element=w773) -> (queue out=w774:refnum<queue>)  [unwired: 2 in, 2 out]
                }
              }
            }
          }
          frame "Task 4_A" {
            # ">> Stepper height reeached >>"
            # ">>> yStepper command>>>"
            # ">> Manual override >>"
            n331 = Dequeue Element(queue=w789, timeout in ms (-1)=w788, error in (no error)=w787) -> (element=w786:T10)  [unwired: 3 out]
            n332 = Equal?(x=w780, y=u8 60) -> (x = y?=w776:bool)
            n333 = case shown="\"Start Task 1\", Default" w786 {
              tunnel: [w801 State_Type_Definitions,_for_0.26g_versions_and_later_3."True Stop" ("Enum")] -> w785
              tunnel: [w799 w817] -> w784
              tunnel: w790 -> [w798 w814]
              tunnel: w783 -> [w792 _]
              tunnel: [State_Type_Definitions,_for_0.26g_versions_and_later_3."Idle" ("Enum") State_Type_Definitions,_for_0.26g_versions_and_later_3."Shutdown" ("Enum")] -> w782
              tunnel: w776 -> [w791 _]
              frame "Start Task 1", Default {
                # ">> WIill proceed to part ii if not manual override >>"
                # ">>If ENABLE or Trigger is set to true>>"
                n334 = Or(x=w791, y=w792) -> (x .or. y?=w793:bool)
                n335 = case shown="False" w791 {
                  tunnel: [w804 w810] -> w799
                  tunnel: w798 -> [w803 w809]
                  frame False {
                    n336 = for {
                      shift-right: [w806] -> w804
                      shift-left: w803 -> [w807]
                      tunnel: string[] ["Z STEPPER CAM HEIGHT", "READ STEPPER VALUES"] ("element") -> [w805] mode=indexing
                      n337 = Enqueue Element(queue=w807, element=w805) -> (queue out=w806:refnum<queue>)  [unwired: 2 in, 2 out]
                    }
                  }
                  frame True {
                    n338 = for {
                      shift-right: [w812] -> w810
                      shift-left: w809 -> [w813]
                      tunnel: string[] ["ARDUINO - ULTRASONIC", "READ ULTRASONIC", "FORWARD", "", "", ""] -> [w811] mode=indexing
                      n339 = Enqueue Element(queue=w813, element=w811) -> (queue out=w812:refnum<queue>)  [unwired: 2 in, 2 out]
                    }
                  }
                }
                n340 = Select(t=State_Type_Definitions,_for_0.26g_versions_and_later_3."True Stop" ("Enum"), s=w792, f=State_Type_Definitions,_for_0.26g_versions_and_later_3."Task 4_B" ("Enum")) -> (s? t:f=w795:T18)
                n341 = Select(t=w795, s=w793, f=State_Type_Definitions,_for_0.26g_versions_and_later_3."Task 4_A" ("Enum")) -> (s? t:f=w801:T18)
              }
              frame "Exit" {
                n342 = for {
                  shift-right: [w820] -> w817
                  shift-left: w814 -> [w821]
                  tunnel: string[] ["STOP", "RESET ENCODERS", "RESET YAW", ""] -> [w819] mode=indexing
                  n343 = Enqueue Element(queue=w821, element=w819) -> (queue out=w820:refnum<queue>)  [unwired: 2 in, 2 out]
                }
              }
            }
          }
          frame "Task 4_B" {
            w827 = u8 20
            # ">> Path blocked >>"
            # ">>> yStepper command>>>"
            # ">> Manual override >>"
            n344 = Dequeue Element(queue=w836, timeout in ms (-1)=w835, error in (no error)=w834) -> (element=w833:T10)  [unwired: 3 out]
            n345 = Less?(x=w829, y=w827) -> (x < y?=w824:bool)
            n346 = Less?(x=w828, y=w827) -> (x < y?=w825:bool)
            n347 = And(x=w825, y=w824) -> (x .and. y?=w826:bool)
            n348 = case shown="\"Start Task 1\", Default" w833 {
              tunnel: [w850 State_Type_Definitions,_for_0.26g_versions_and_later_3."True Stop" ("Enum")] -> w838
              tunnel: [w848 w865] -> w839
              tunnel: w832 -> [w847 _]
              tunnel: w837 -> [w841 _]
              tunnel: [State_Type_Definitions,_for_0.26g_versions_and_later_3."Idle" ("Enum") State_Type_Definitions,_for_0.26g_versions_and_later_3."Shutdown" ("Enum")] -> w831
              tunnel: w826 -> [w840 _]
              frame "Start Task 1", Default {
                # ">> Manual override forces program to true stop >>"
                # ">>If ENABLE or Trigger is set to true>>"
                n349 = Or(x=w840, y=w841) -> (x .or. y?=w846:bool)
                n350 = case shown="False" w840 {
                  tunnel: [w853 w858] -> w848
                  tunnel: w847 -> [w852 w857]
                  frame False {
                    n351 = for {
                      shift-right: [w855] -> w853
                      shift-left: w852 -> [w856]
                      tunnel: string[] ["FORWARD", "READ ULTRASONIC", "READ NAVX"] ("element") -> [w854] mode=indexing
                      n352 = Enqueue Element(queue=w856, element=w854) -> (queue out=w855:refnum<queue>)  [unwired: 2 in, 2 out]
                    }
                  }
                  frame True {
                    n353 = for {
                      shift-right: [w861] -> w858
                      shift-left: w857 -> [w862]
                      tunnel: string[] ["STOP", "RESET YAW", "RESET ENCODERS", "RESET FLAGS"] -> [w860] mode=indexing
                      n354 = Enqueue Element(queue=w862, element=w860) -> (queue out=w861:refnum<queue>)  [unwired: 2 in, 2 out]
                    }
                  }
                }
                n355 = Select(t=State_Type_Definitions,_for_0.26g_versions_and_later_3."True Stop" ("Enum"), s=w841, f=State_Type_Definitions,_for_0.26g_versions_and_later_3."Task 4_C" ("Enum")) -> (s? t:f=w843:T18)
                n356 = Select(t=w843, s=w846, f=State_Type_Definitions,_for_0.26g_versions_and_later_3."Task 4_B" ("Enum")) -> (s? t:f=w850:T18)
              }
              frame "Exit" {
                n357 = for {
                  shift-right: [w868] -> w865
                  shift-left: _ -> [w869]
                  tunnel: string[] ["STOP", "RESET ENCODERS", "RESET YAW", ""] -> [w867] mode=indexing
                  n358 = Enqueue Element(queue=w869, element=w867) -> (queue out=w868:refnum<queue>)  [unwired: 2 in, 2 out]
                }
              }
            }
          }
          frame "Task 4_C" {
            w881 = u8 20
            # ">> xDistance travelled>>"
            # ">> Path NOT blocked >>"
            # ">>> yStepper command>>>"
            # ">> Manual override >>"
            n359 = Dequeue Element(queue=w891, timeout in ms (-1)=w884, error in (no error)=w883) -> (element=w885:T10)  [unwired: 3 out]
            n360 = Greater?(x=w873, y=w881) -> (0:w879:bool)
            n361 = Greater?(x=w878, y=80.0) -> (0:w876:bool)
            n362 = Greater?(x=w872, y=w881) -> (0:w880:bool)
            n363 = And(x=w880, y=w879) -> (x .and. y?=w875:bool)
            n364 = And(x=w876, y=w875) -> (x .and. y?=w874:bool)
            n365 = case shown="\"Start Task 1\", Default" w885 {
              tunnel: [w902 State_Type_Definitions,_for_0.26g_versions_and_later_3."True Stop" ("Enum")] -> w888
              tunnel: [w900 w918] -> w887
              tunnel: w890 -> [w899 w915]
              tunnel: w889 -> [w893 _]
              tunnel: [State_Type_Definitions,_for_0.26g_versions_and_later_3."Idle" ("t") State_Type_Definitions,_for_0.26g_versions_and_later_3."Shutdown" ("Enum")] -> w886
              tunnel: w874 -> [w892 _]
              frame "Start Task 1", Default {
                # ">> Manual override forces program to true stop >>"
                # ">>If ENABLE or Trigger is set to true>>"
                n366 = Or(x=w892, y=w893) -> (x .or. y?=w898:bool)
                n367 = case shown="False" w892 {
                  tunnel: [w905 w910] -> w900
                  tunnel: w899 -> [w903 w909]
                  frame False {
                    n368 = for {
                      shift-right: [w907] -> w905
                      shift-left: w903 -> [w908]
                      tunnel: string[] ["RIGHT", "READ NAVX", "READ ENCODERS", "READ ULTRASONIC"] ("element") -> [w906] mode=indexing
                      n369 = Enqueue Element(queue=w908, element=w906) -> (queue out=w907:refnum<queue>)  [unwired: 2 in, 2 out]
                    }
                  }
                  frame True {
                    n370 = for {
                      shift-right: [w913] -> w910
                      shift-left: w909 -> [w914]
                      tunnel: string[] ["STOP", "RESET YAW", "RESET ENCODERS", "ARDUINO - ULTRASONIC"] -> [w912] mode=indexing
                      n371 = Enqueue Element(queue=w914, element=w912) -> (queue out=w913:refnum<queue>)  [unwired: 2 in, 2 out]
                    }
                  }
                }
                n372 = Select(t=State_Type_Definitions,_for_0.26g_versions_and_later_3."True Stop" ("Enum"), s=w893, f=State_Type_Definitions,_for_0.26g_versions_and_later_3."Task 4_D" ("Enum")) -> (s? t:f=w894:T18)
                n373 = Select(t=w894, s=w898, f=State_Type_Definitions,_for_0.26g_versions_and_later_3."Task 4_C" ("Enum")) -> (s? t:f=w902:T18)
              }
              frame "Exit" {
                n374 = for {
                  shift-right: [w921] -> w918
                  shift-left: w915 -> [w922]
                  tunnel: string[] ["STOP", "RESET ENCODERS", "RESET YAW", ""] -> [w920] mode=indexing
                  n375 = Enqueue Element(queue=w922, element=w920) -> (queue out=w921:refnum<queue>)  [unwired: 2 in, 2 out]
                }
              }
            }
          }
          frame "Task 4_D" {
            w945 = u8 20
            # ">>> Motor control cluster >>>"
            # ">> Line detected >>"
            # ">> yDistance travelled>>"
            # ">> Path blocked >>"
            # ">>> yStepper command>>>"
            # ">> Manual override >>"
            n376 = Less?(x=w930, y=w945) -> (x < y?=w943:bool)
            n377 = Greater?(x=w934, y=200.0) -> (0:w941:bool)
            n378 = Less?(x=w929, y=w945) -> (x < y?=w944:bool)
            n379 = And(x=w944, y=w943) -> (x .and. y?=w940:bool)
            n380 = Dequeue Element(queue=w937, timeout in ms (-1)=w936, error in (no error)=w935) -> (element=w946:T10)  [unwired: 3 out]
            n381 = Or(x=w941, y=w940) -> (x .or. y?=w924:bool)
            n382 = And(x=w925, y=w924) -> (x .and. y?=w923:bool)
            n383 = case shown="\"Start Task 1\", Default" w946 {
              tunnel: [w957 State_Type_Definitions,_for_0.26g_versions_and_later_3."True Stop" ("Enum")] -> w933
              tunnel: [w955 w973] -> w931
              tunnel: w938 -> [w954 w970]
              tunnel: w939 -> [w948 _]
              tunnel: [State_Type_Definitions,_for_0.26g_versions_and_later_3."Idle" ("t") State_Type_Definitions,_for_0.26g_versions_and_later_3."Shutdown" ("Enum")] -> w932
              tunnel: w923 -> [w947 _]
              frame "Start Task 1", Default {
                # ">> Manual override forces program to true stop >>"
                # ">>If ENABLE or Trigger is set to true>>"
                n384 = Or(x=w947, y=w948) -> (x .or. y?=w953:bool)
                n385 = case shown="False" w947 {
                  tunnel: [w960 w965] -> w955
                  tunnel: w954 -> [w958 w964]
                  frame False {
                    n386 = for {
                      shift-right: [w962] -> w960
                      shift-left: w958 -> [w963]
                      tunnel: string[] ["FORWARD", "READ NAVX", "READ ENCODERS", "READ ULTRASONIC", "READ LINE SENSOR"] ("element") -> [w961] mode=indexing
                      n387 = Enqueue Element(queue=w963, element=w961) -> (queue out=w962:refnum<queue>)  [unwired: 2 in, 2 out]
                    }
                  }
                  frame True {
                    n388 = for {
                      shift-right: [w968] -> w965
                      shift-left: w964 -> [w969]
                      tunnel: string[] ["STOP", "RESET YAW", "RESET ENCODERS", "RESET FLAGS"] -> [w967] mode=indexing
                      n389 = Enqueue Element(queue=w969, element=w967) -> (queue out=w968:refnum<queue>)  [unwired: 2 in, 2 out]
                    }
                  }
                }
                n390 = Select(t=State_Type_Definitions,_for_0.26g_versions_and_later_3."True Stop" ("Enum"), s=w948, f=State_Type_Definitions,_for_0.26g_versions_and_later_3."True Stop" ("Enum")) -> (s? t:f=w949:T18)
                n391 = Select(t=w949, s=w953, f=State_Type_Definitions,_for_0.26g_versions_and_later_3."Task 4_D" ("Enum")) -> (s? t:f=w957:T18)
              }
              frame "Exit" {
                n392 = for {
                  shift-right: [w976] -> w973
                  shift-left: w970 -> [w977]
                  tunnel: string[] ["STOP", "RESET ENCODERS", "RESET YAW", ""] -> [w975] mode=indexing
                  n393 = Enqueue Element(queue=w977, element=w975) -> (queue out=w976:refnum<queue>)  [unwired: 2 in, 2 out]
                }
              }
            }
          }
          frame "Task 5A: RAISING ARM" {
            # "Stays in Task 5_A until stepper reaches desired \nheight"
            # ">>> Motor control cluster >>>"
            # ">>> yStepper command>>>"
            # ">> Manual override >>"
            n394 = Dequeue Element(queue=w988, timeout in ms (-1)=w987, error in (no error)=w989) -> (element=w986:T10)  [unwired: 3 out]
            n395 = Equal?(x=w985, y=u8 60) -> (x = y?=w983:bool)
            n396 = case shown="\"Start Task 1\", Default" w986 {
              tunnel: [w999 State_Type_Definitions,_for_0.26g_versions_and_later_3."True Stop" ("Enum")] -> w990
              tunnel: [w1002 w1019] -> w991
              tunnel: [State_Type_Definitions,_for_0.26g_versions_and_later_3."Idle" ("Enum") State_Type_Definitions,_for_0.26g_versions_and_later_3."Shutdown" ("Enum")] -> w992
              tunnel: w983 -> [w998 _]
              tunnel: w982 -> [w997 _]
              tunnel: w981 -> [w993 w1016]
              frame "Start Task 1", Default {
                # "T: Go back to idle, F: Continue with task\""
                # ">> Manual override >>"
                n397 = case shown="True" w998 {
                  tunnel: [w1006 w1012] -> w1002
                  tunnel: w993 -> [w1004 w1010]
                  frame False {
                    n398 = for {
                      tunnel: string[] ["Z STEPPER GRAB HEIGHT", "READ STEPPER VALUES"] ("element") -> [w1007] mode=indexing
                      shift-right: [w1009] -> w1006
                      shift-left: w1004 -> [w1008]
                      n399 = Enqueue Element(queue=w1008, element=w1007) -> (queue out=w1009:refnum<queue>)  [unwired: 2 in, 2 out]
                    }
                  }
                  frame True {
                    n400 = for {
                      shift-right: [w1014] -> w1012
                      shift-left: w1010 -> [w1015]
                      tunnel: string[] ["", "", ""] -> [w1013] mode=indexing
                      n401 = Enqueue Element(queue=w1015, element=w1013) -> (queue out=w1014:refnum<queue>)  [unwired: 2 in, 2 out]
                    }
                  }
                }
                n402 = Or(x=w998, y=w997) -> (x .or. y?=w1000:bool)
                n403 = Select(t=State_Type_Definitions,_for_0.26g_versions_and_later_3."True Stop" ("Enum"), s=w997, f=State_Type_Definitions,_for_0.26g_versions_and_later_3."Task 5B: STILL WAITING" ("Enum")) -> (s? t:f=w994:T18)
                n404 = Select(t=w994, s=w1000, f=State_Type_Definitions,_for_0.26g_versions_and_later_3."Task 5A: RAISING ARM" ("Enum")) -> (s? t:f=w999:T18)
              }
              frame "Exit" {
                n405 = for {
                  shift-right: [w1022] -> w1019
                  shift-left: w1016 -> [w1023]
                  tunnel: string[] ["STOP", "RESET ENCODERS", "RESET YAW", "ARDUINO MODE 0"] -> [w1021] mode=indexing
                  n406 = Enqueue Element(queue=w1023, element=w1021) -> (queue out=w1022:refnum<queue>)  [unwired: 2 in, 2 out]
                }
              }
            }
          }
          frame "Task 5B: STILL WAITING" {
            # ">>> yStepper command>>>"
            n407 = Dequeue Element(queue=w1030, timeout in ms (-1)=w1029, error in (no error)=w1031) -> (element=w1028:T10)  [unwired: 3 out]
            n408 = local read "Rising Edge"() -> (w1024:bool)
            n409 = case shown="\"Start Task 1\", Default" w1028 {
              tunnel: [w1043 State_Type_Definitions,_for_0.26g_versions_and_later_3."True Stop" ("Enum")] -> w1033
              tunnel: [w1046 w1063] -> w1032
              tunnel: [State_Type_Definitions,_for_0.26g_versions_and_later_3."Idle" ("Enum") State_Type_Definitions,_for_0.26g_versions_and_later_3."Shutdown" ("Enum")] -> w1034
              tunnel: w1036 -> [w1042 _]
              tunnel: w1035 -> [w1038 w1060]
              tunnel: w1024 -> [w1037 _]
              frame "Start Task 1", Default {
                # "T: Go back to idle, F: Continue with task\""
                # ">> Manual override >>"
                n410 = case shown="True" w1037 {
                  tunnel: [w1050 w1056] -> w1046
                  tunnel: w1038 -> [w1048 w1054]
                  frame False {
                    n411 = for {
                      tunnel: string[] ["CLOSE CLAW", "START TIMER", ""] ("element") -> [w1051] mode=indexing
                      shift-right: [w1053] -> w1050
                      shift-left: w1048 -> [w1052]
                      n412 = Enqueue Element(queue=w1052, element=w1051) -> (queue out=w1053:refnum<queue>)  [unwired: 2 in, 2 out]
                    }
                  }
                  frame True {
                    n413 = for {
                      shift-right: [w1058] -> w1056
                      shift-left: w1054 -> [w1059]
                      tunnel: string[] ["STOP", "", "", ""] -> [w1057] mode=indexing
                      n414 = Enqueue Element(queue=w1059, element=w1057) -> (queue out=w1058:refnum<queue>)  [unwired: 2 in, 2 out]
                    }
                  }
                }
                n415 = Or(x=w1037, y=w1042) -> (x .or. y?=w1044:bool)
                n416 = Select(t=State_Type_Definitions,_for_0.26g_versions_and_later_3."True Stop" ("Enum"), s=w1042, f=State_Type_Definitions,_for_0.26g_versions_and_later_3."Task 5C: GOING DOWN" ("Enum")) -> (s? t:f=w1039:T18)
                n417 = Select(t=w1039, s=w1044, f=State_Type_Definitions,_for_0.26g_versions_and_later_3."Task 5B: STILL WAITING" ("Enum")) -> (s? t:f=w1043:T18)
              }
              frame "Exit" {
                n418 = for {
                  shift-right: [w1066] -> w1063
                  shift-left: w1060 -> [w1067]
                  tunnel: string[] ["STOP", "RESET ENCODERS", "RESET YAW", "ARDUINO MODE 0"] -> [w1065] mode=indexing
                  n419 = Enqueue Element(queue=w1067, element=w1065) -> (queue out=w1066:refnum<queue>)  [unwired: 2 in, 2 out]
                }
              }
            }
          }
          frame "Task 5C: GOING DOWN" {
            # ">>> Motor control cluster >>>"
            # ">>> yStepper command>>>"
            # ">> Manual override >>"
            n420 = Equal?(x=w1070, y=u8 1) -> (x = y?=w1068:bool)
            n421 = Dequeue Element(queue=w1080, timeout in ms (-1)=w1079, error in (no error)=w1078) -> (element=w1077:T10)  [unwired: 3 out]
            n422 = case shown="\"Start Task 1\", Default" w1077 {
              tunnel: [w1089 State_Type_Definitions,_for_0.26g_versions_and_later_3."True Stop" ("Enum")] -> w1082
              tunnel: [w1092 w1109] -> w1075
              tunnel: [State_Type_Definitions,_for_0.26g_versions_and_later_3."Idle" ("Enum") State_Type_Definitions,_for_0.26g_versions_and_later_3."Shutdown" ("Enum")] -> w1074
              tunnel: w1076 -> [w1083 _]
              tunnel: w1081 -> [w1088 w1106]
              tunnel: w1068 -> [w1087 _]
              frame "Start Task 1", Default {
                # ">> Is time up? >>"
                # "Determines if object is in range to pick up"
                # ">> Manual override >>"
                n423 = case shown="False" w1087 {
                  tunnel: [w1096 w1102] -> w1092
                  tunnel: w1088 -> [w1095 w1100]
                  frame False {
                    n424 = for {
                      tunnel: string[] ["Z STEPPER GRAB HEIGHT", "READ STEPPER VALUES", "", ""] -> [w1097] mode=indexing
                      shift-right: [w1099] -> w1096
                      shift-left: w1095 -> [w1098]
                      n425 = Enqueue Element(queue=w1098, element=w1097) -> (queue out=w1099:refnum<queue>)  [unwired: 2 in, 2 out]
                    }
                  }
                  frame True {
                    n426 = for {
                      shift-right: [w1104] -> w1102
                      shift-left: w1100 -> [w1105]
                      tunnel: string[] ["SET TIMER 5", "", ""] -> [w1103] mode=indexing
                      n427 = Enqueue Element(queue=w1105, element=w1103) -> (queue out=w1104:refnum<queue>)  [unwired: 2 in, 2 out]
                    }
                  }
                }
                n428 = Or(x=w1087, y=w1083) -> (x .or. y?=w1090:bool)
                n429 = Select(t=State_Type_Definitions,_for_0.26g_versions_and_later_3."True Stop" ("Enum"), s=w1083, f=State_Type_Definitions,_for_0.26g_versions_and_later_3."Task 5D: GRAB" ("Enum")) -> (s? t:f=w1085:T18)
                n430 = Select(t=w1085, s=w1090, f=State_Type_Definitions,_for_0.26g_versions_and_later_3."Task 5C: GOING DOWN" ("Enum")) -> (s? t:f=w1089:T18)
              }
              frame "Exit" {
                n431 = for {
                  shift-right: [w1112] -> w1109
                  shift-left: w1106 -> [w1113]
                  tunnel: string[] ["STOP", "RESET ENCODERS", "RESET YAW", "ARDUINO MODE 0"] -> [w1111] mode=indexing
                  n432 = Enqueue Element(queue=w1113, element=w1111) -> (queue out=w1112:refnum<queue>)  [unwired: 2 in, 2 out]
                }
              }
            }
          }
          frame "Task 5D: GRAB" {
            # ">>> Motor control cluster >>>"
            # ">>> yStepper command>>>"
            n433 = Dequeue Element(queue=w1121, timeout in ms (-1)=w1120, error in (no error)=w1119) -> (element=w1118:T10)  [unwired: 3 out]
            n434 = case shown="\"Start Task 1\", Default" w1118 {
              tunnel: [w1133 State_Type_Definitions,_for_0.26g_versions_and_later_3."True Stop" ("Enum")] -> w1125
              tunnel: [w1136 w1153] -> w1124
              tunnel: [State_Type_Definitions,_for_0.26g_versions_and_later_3."Idle" ("Enum") State_Type_Definitions,_for_0.26g_versions_and_later_3."Shutdown" ("Enum")] -> w1126
              tunnel: w1122 -> [w1132 _]
              tunnel: w1123 -> [w1128 w1150]
              tunnel: w1116 -> [w1127 _]
              frame "Start Task 1", Default {
                # ">> T: Breaks out of state loop; F: Stays in loop>>"
                # ">> Manual override >>"
                # ">> Checks if time is up>>"
                # "Stays in Task 5D until the object is detected"
                # "T: Go back to idle, F: Continue with task\""
                # ">> Manual override >>"
                n435 = case shown="False" w1127 {
                  tunnel: [w1140 w1146] -> w1136
                  tunnel: w1128 -> [w1138 w1144]
                  frame False {
                    n436 = for {
                      tunnel: string[] ["START TIMER", "OPEN CLAW", ""] ("element") -> [w1141] mode=indexing
                      shift-right: [w1143] -> w1140
                      shift-left: w1138 -> [w1142]
                      n437 = Enqueue Element(queue=w1142, element=w1141) -> (queue out=w1143:refnum<queue>)  [unwired: 2 in, 2 out]
                    }
                  }
                  frame True {
                    n438 = for {
                      shift-right: [w1148] -> w1146
                      shift-left: w1144 -> [w1149]
                      tunnel: string[] ["CAM CLOSE", "", ""] -> [w1147] mode=indexing
                      n439 = Enqueue Element(queue=w1149, element=w1147) -> (queue out=w1148:refnum<queue>)  [unwired: 2 in, 2 out]
                    }
                  }
                }
                n440 = Or(x=w1127, y=w1132) -> (x .or. y?=w1134:bool)
                n441 = Select(t=State_Type_Definitions,_for_0.26g_versions_and_later_3."True Stop" ("Enum"), s=w1132, f=State_Type_Definitions,_for_0.26g_versions_and_later_3."Task 5E: GOING UP" ("Enum")) -> (s? t:f=w1129:T18)
                n442 = Select(t=w1129, s=w1134, f=State_Type_Definitions,_for_0.26g_versions_and_later_3."Task 5D: GRAB" ("Enum")) -> (s? t:f=w1133:T18)
              }
              frame "Exit" {
                n443 = for {
                  shift-right: [w1156] -> w1153
                  shift-left: w1150 -> [w1157]
                  tunnel: string[] ["STOP", "RESET ENCODERS", "RESET YAW", "ARDUINO MODE 0"] -> [w1155] mode=indexing
                  n444 = Enqueue Element(queue=w1157, element=w1155) -> (queue out=w1156:refnum<queue>)  [unwired: 2 in, 2 out]
                }
              }
            }
          }
          frame "Task 5E: GOING UP" {
            # ">>> yStepper command>>>"
            n445 = Dequeue Element(queue=w1171, timeout in ms (-1)=w1172, error in (no error)=w1173) -> (element=w1175:T10)  [unwired: 3 out]
            n446 = formula code="if (pos < 100)\ny = 41;\n\nelse if (pos >= 100 && pos <= 140)\ny = 30;\n\nelse if (pos >= 141 && pos <= 170)\ny = 25;\n\nelse if (pos >= 171 &&pos <= 180) \ny = 20;\n\nelse if (pos >= 181&& pos <= 200)\ny = 15;\n\nelse if (pos >= 201 && pos <= 230)\ny = 10;\n\nelse if (pos >= 231 && pos <= 320)\ny = 8;\n\nelse if (pos > 320)\ny = 0;"("pos"=w1163) -> ("y"=w1166:dbl)
            n447 = To Unsigned Byte Integer(number=w1166) -> (unsigned 8bit integer=w1161:u8)
            n448 = Equal?(x=w1162, y=w1161) -> (x = y?=w1160:bool)
            n449 = case shown="\"Start Task 1\", Default" w1175 {
              tunnel: [w1182 State_Type_Definitions,_for_0.26g_versions_and_later_3."True Stop" ("Enum")] -> w1169
              tunnel: [w1185 w1202] -> w1167
              tunnel: [State_Type_Definitions,_for_0.26g_versions_and_later_3."Idle" ("Enum") State_Type_Definitions,_for_0.26g_versions_and_later_3."Shutdown" ("Enum")] -> w1168
              tunnel: w1174 -> [w1181 _]
              tunnel: w1170 -> [w1177 w1199]
              tunnel: w1160 -> [w1176 _]
              frame "Start Task 1", Default {
                # ">> T: Breaks out of state loop; F: Stays in loop>>"
                # ">> Manual override >>"
                # ">> Checks if time is up>>"
                # "Stays in Task 5D until the object is detected"
                # "T: Go back to idle, F: Continue with task\""
                # ">> Manual override >>"
                n450 = case shown="False" w1176 {
                  tunnel: [w1189 w1195] -> w1185
                  tunnel: w1177 -> [w1187 w1193]
                  frame False {
                    n451 = for {
                      tunnel: string[] ["READ STEPPER VALUES", "Y STEPPER CONTROL", ""] ("element") -> [w1190] mode=indexing
                      shift-right: [w1192] -> w1189
                      shift-left: w1187 -> [w1191]
                      n452 = Enqueue Element(queue=w1191, element=w1190) -> (queue out=w1192:refnum<queue>)  [unwired: 2 in, 2 out]
                    }
                  }
                  frame True {
                    n453 = for {
                      shift-right: [w1197] -> w1195
                      shift-left: w1193 -> [w1198]
                      tunnel: string[] ["CAM CLOSE", "DISPOSE BUFFERS", ""] -> [w1196] mode=indexing
                      n454 = Enqueue Element(queue=w1198, element=w1196) -> (queue out=w1197:refnum<queue>)  [unwired: 2 in, 2 out]
                    }
                  }
                }
                n455 = Or(x=w1176, y=w1181) -> (x .or. y?=w1183:bool)
                n456 = Select(t=State_Type_Definitions,_for_0.26g_versions_and_later_3."True Stop" ("Enum"), s=w1181, f=State_Type_Definitions,_for_0.26g_versions_and_later_3."Task 5F: ARM GRAB HEIGHT" ("Enum")) -> (s? t:f=w1178:T18)
                n457 = Select(t=w1178, s=w1183, f=State_Type_Definitions,_for_0.26g_versions_and_later_3."Task 5E: GOING UP" ("Enum")) -> (s? t:f=w1182:T18)
              }
              frame "Exit" {
                n458 = for {
                  shift-right: [w1205] -> w1202
                  shift-left: w1199 -> [w1206]
                  tunnel: string[] ["STOP", "RESET ENCODERS", "RESET YAW", "ARDUINO MODE 0"] -> [w1204] mode=indexing
                  n459 = Enqueue Element(queue=w1206, element=w1204) -> (queue out=w1205:refnum<queue>)  [unwired: 2 in, 2 out]
                }
              }
            }
            n460 = Bundle By Name(cluster=w1165, "yStepper desired"=w1161) -> (w1164:T20)
          }
          frame "Task 5F: ARM GRAB HEIGHT" {
            # ">>> Motor control cluster >>>"
            # ">>> yStepper command>>>"
            # ">> Manual override >>"
            n461 = Dequeue Element(queue=w1217, timeout in ms (-1)=w1216, error in (no error)=w1218) -> (element=w1215:T10)  [unwired: 3 out]
            n462 = Equal?(x=w1214, y=u8 1) -> (x = y?=w1212:bool)
            n463 = case shown="\"Start Task 1\", Default" w1215 {
              tunnel: [w1228 State_Type_Definitions,_for_0.26g_versions_and_later_3."True Stop" ("Enum")] -> w1219
              tunnel: [w1231 w1248] -> w1220
              tunnel: [State_Type_Definitions,_for_0.26g_versions_and_later_3."Idle" ("Enum") State_Type_Definitions,_for_0.26g_versions_and_later_3."Shutdown" ("Enum")] -> w1221
              tunnel: w1212 -> [w1227 _]
              tunnel: w1211 -> [w1226 _]
              tunnel: w1210 -> [w1222 w1245]
              frame "Start Task 1", Default {
                # "Stays in Task 5F until stepper reaches desired \nheight"
                # "T: Go back to idle, F: Continue with task\""
                # ">> Manual override >>"
                n464 = case shown="True" w1227 {
                  tunnel: [w1235 w1241] -> w1231
                  tunnel: w1222 -> [w1233 w1239]
                  frame False {
                    n465 = for {
                      tunnel: string[] ["Z STEPPER GRAB HEIGHT", "READ STEPPER VALUES"] ("element") -> [w1236] mode=indexing
                      shift-right: [w1238] -> w1235
                      shift-left: w1233 -> [w1237]
                      n466 = Enqueue Element(queue=w1237, element=w1236) -> (queue out=w1238:refnum<queue>)  [unwired: 2 in, 2 out]
                    }
                  }
                  frame True {
                    n467 = for {
                      shift-right: [w1243] -> w1241
                      shift-left: w1239 -> [w1244]
                      tunnel: string[] ["SET TIMER 5", "CLOSE CLAW", ""] -> [w1242] mode=indexing
                      n468 = Enqueue Element(queue=w1244, element=w1242) -> (queue out=w1243:refnum<queue>)  [unwired: 2 in, 2 out]
                    }
                  }
                }
                n469 = Or(x=w1227, y=w1226) -> (x .or. y?=w1229:bool)
                n470 = Select(t=State_Type_Definitions,_for_0.26g_versions_and_later_3."True Stop" ("Enum"), s=w1226, f=State_Type_Definitions,_for_0.26g_versions_and_later_3."Task 5G: CLOSE CLAW" ("Enum")) -> (s? t:f=w1223:T18)
                n471 = Select(t=w1223, s=w1229, f=State_Type_Definitions,_for_0.26g_versions_and_later_3."Task 5F: ARM GRAB HEIGHT" ("Enum")) -> (s? t:f=w1228:T18)
              }
              frame "Exit" {
                n472 = for {
                  shift-right: [w1251] -> w1248
                  shift-left: w1245 -> [w1252]
                  tunnel: string[] ["STOP", "RESET ENCODERS", "RESET YAW", "ARDUINO MODE 0"] -> [w1250] mode=indexing
                  n473 = Enqueue Element(queue=w1252, element=w1250) -> (queue out=w1251:refnum<queue>)  [unwired: 2 in, 2 out]
                }
              }
            }
          }
          frame "Task 5G: CLOSE CLAW" {
            # ">>> yStepper command>>>"
            # ">> Manual override >>"
            n474 = Dequeue Element(queue=w1263, timeout in ms (-1)=w1262, error in (no error)=w1261) -> (element=w1260:T10)  [unwired: 3 out]
            n475 = case shown="\"Start Task 1\", Default" w1260 {
              tunnel: [w1272 State_Type_Definitions,_for_0.26g_versions_and_later_3."True Stop" ("Enum")] -> w1265
              tunnel: [w1275 w1292] -> w1258
              tunnel: [State_Type_Definitions,_for_0.26g_versions_and_later_3."Idle" ("Enum") State_Type_Definitions,_for_0.26g_versions_and_later_3."Shutdown" ("Enum")] -> w1257
              tunnel: w1259 -> [w1266 _]
              tunnel: w1264 -> [w1271 w1289]
              tunnel: w1255 -> [w1270 _]
              frame "Start Task 1", Default {
                # ">> Is time up? >>"
                # "Determines if object is in range to pick up"
                # ">> Manual override >>"
                n476 = case shown="True" w1270 {
                  tunnel: [w1279 w1285] -> w1275
                  tunnel: w1271 -> [w1277 w1283]
                  frame False {
                    n477 = for {
                      tunnel: string[] ["CLOSE CLAW", "START TIMER"] ("element") -> [w1280] mode=indexing
                      shift-right: [w1282] -> w1279
                      shift-left: w1277 -> [w1281]
                      n478 = Enqueue Element(queue=w1281, element=w1280) -> (queue out=w1282:refnum<queue>)  [unwired: 2 in, 2 out]
                    }
                  }
                  frame True {
                    n479 = for {
                      shift-right: [w1287] -> w1285
                      shift-left: w1283 -> [w1288]
                      tunnel: string[] ["READ STEPPER VALUES", "", ""] -> [w1286] mode=indexing
                      n480 = Enqueue Element(queue=w1288, element=w1286) -> (queue out=w1287:refnum<queue>)  [unwired: 2 in, 2 out]
                    }
                  }
                }
                n481 = Or(x=w1270, y=w1266) -> (x .or. y?=w1273:bool)
                n482 = Select(t=State_Type_Definitions,_for_0.26g_versions_and_later_3."True Stop" ("Enum"), s=w1266, f=State_Type_Definitions,_for_0.26g_versions_and_later_3."Task 5H: RAISE ARM" ("Enum")) -> (s? t:f=w1268:T18)
                n483 = Select(t=w1268, s=w1273, f=State_Type_Definitions,_for_0.26g_versions_and_later_3."Task 5G: CLOSE CLAW" ("Enum")) -> (s? t:f=w1272:T18)
              }
              frame "Exit" {
                n484 = for {
                  shift-right: [w1295] -> w1292
                  shift-left: w1289 -> [w1296]
                  tunnel: string[] ["STOP", "RESET ENCODERS", "RESET YAW", "ARDUINO MODE 0"] -> [w1294] mode=indexing
                  n485 = Enqueue Element(queue=w1296, element=w1294) -> (queue out=w1295:refnum<queue>)  [unwired: 2 in, 2 out]
                }
              }
            }
          }
          frame "Task 5H: RAISE ARM" {
            # ">>> yStepper command>>>"
            # ">> Manual override >>"
            n486 = Dequeue Element(queue=w1307, timeout in ms (-1)=w1306, error in (no error)=w1308) -> (element=w1305:T10)  [unwired: 3 out]
            n487 = Equal?(x=w1304, y=u8 60) -> (x = y?=w1302:bool)
            n488 = case shown="\"Start Task 1\", Default" w1305 {
              tunnel: [w1318 State_Type_Definitions,_for_0.26g_versions_and_later_3."True Stop" ("Enum")] -> w1309
              tunnel: [w1321 w1338] -> w1310
              tunnel: [State_Type_Definitions,_for_0.26g_versions_and_later_3."Idle" ("Enum") State_Type_Definitions,_for_0.26g_versions_and_later_3."Shutdown" ("Enum")] -> w1311
              tunnel: w1302 -> [w1317 _]
              tunnel: w1301 -> [w1316 _]
              tunnel: w1300 -> [w1312 w1335]
              frame "Start Task 1", Default {
                # "Stays in Task 5_A until stepper reaches desired \nheight"
                # "T: Go back to idle, F: Continue with task\""
                # ">> Manual override >>"
                n489 = case shown="False" w1317 {
                  tunnel: [w1325 w1331] -> w1321
                  tunnel: w1312 -> [w1323 w1329]
                  frame False {
                    n490 = for {
                      tunnel: string[] ["Z STEPPER CAM HEIGHT", "READ STEPPER VALUES"] ("element") -> [w1326] mode=indexing
                      shift-right: [w1328] -> w1325
                      shift-left: w1323 -> [w1327]
                      n491 = Enqueue Element(queue=w1327, element=w1326) -> (queue out=w1328:refnum<queue>)  [unwired: 2 in, 2 out]
                    }
                  }
                  frame True {
                    n492 = for {
                      shift-right: [w1333] -> w1331
                      shift-left: w1329 -> [w1334]
                      tunnel: string[] ["ARDUINO - ULTRASONIC", "READ ULTRASONIC", ""] -> [w1332] mode=indexing
                      n493 = Enqueue Element(queue=w1334, element=w1332) -> (queue out=w1333:refnum<queue>)  [unwired: 2 in, 2 out]
                    }
                  }
                }
                n494 = Or(x=w1317, y=w1316) -> (x .or. y?=w1319:bool)
                n495 = Select(t=State_Type_Definitions,_for_0.26g_versions_and_later_3."True Stop" ("Enum"), s=w1316, f=State_Type_Definitions,_for_0.26g_versions_and_later_3."True Stop" ("Enum")) -> (s? t:f=w1313:T18)
                n496 = Select(t=w1313, s=w1319, f=State_Type_Definitions,_for_0.26g_versions_and_later_3."Task 5H: RAISE ARM" ("Enum")) -> (s? t:f=w1318:T18)
              }
              frame "Exit" {
                n497 = for {
                  shift-right: [w1341] -> w1338
                  shift-left: w1335 -> [w1342]
                  tunnel: string[] ["STOP", "RESET ENCODERS", "RESET YAW", "ARDUINO MODE 0"] -> [w1340] mode=indexing
                  n498 = Enqueue Element(queue=w1342, element=w1340) -> (queue out=w1341:refnum<queue>)  [unwired: 2 in, 2 out]
                }
              }
            }
          }
          frame "Task 6A: RAISE ARM" {
            # ">>> Motor control cluster >>>"
            # ">>> yStepper command>>>"
            n499 = Equal?(x=w1350, y=u8 60) -> (x = y?=w1344:bool)
            n500 = Dequeue Element(queue=w1354, timeout in ms (-1)=w1353, error in (no error)=w1352) -> (element=w1359:T10)  [unwired: 3 out]
            n501 = local read "Rising Edge"() -> (w1345:bool)
            n502 = And(x=w1345, y=w1344) -> (x .and. y?=w1343:bool)
            n503 = case shown="\"Start Task 1\", Default" w1359 {
              tunnel: [w1369 State_Type_Definitions,_for_0.26g_versions_and_later_3."True Stop" ("Enum")] -> w1357
              tunnel: [w1368 w1385] -> w1356
              tunnel: [State_Type_Definitions,_for_0.26g_versions_and_later_3."Idle" ("Enum") State_Type_Definitions,_for_0.26g_versions_and_later_3."Shutdown" ("Enum")] -> w1358
              tunnel: w1355 -> [w1365 _]
              tunnel: w1351 -> [w1366 _]
              tunnel: w1343 -> [w1363 _]
              frame "Start Task 1", Default {
                n504 = Or(x=w1363, y=w1365) -> (x .or. y?=w1360:bool)
                n505 = case shown="False" w1360 {
                  tunnel: [w1373 w1379] -> w1368
                  tunnel: w1366 -> [w1371 w1378]
                  frame False {
                    n506 = for {
                      tunnel: string[] ["Z STEPPER CAM HEIGHT", "READ STEPPER VALUES"] ("element") -> [w1374] mode=indexing
                      shift-right: [w1376] -> w1373
                      shift-left: w1371 -> [w1375]
                      n507 = Enqueue Element(queue=w1375, element=w1374) -> (queue out=w1376:refnum<queue>)  [unwired: 2 in, 2 out]
                    }
                  }
                  frame True {
                    n508 = for {
                      shift-right: [w1381] -> w1379
                      shift-left: w1378 -> [w1382]
                      tunnel: string[] ["OPEN LOG CAM", "SET TIMER 2", "OPEN IMAQ REF", "", ""] -> [w1380] mode=indexing
                      n509 = Enqueue Element(queue=w1382, element=w1380) -> (queue out=w1381:refnum<queue>)  [unwired: 2 in, 2 out]
                    }
                  }
                }
                n510 = Select(t=State_Type_Definitions,_for_0.26g_versions_and_later_3."Task 6B: CAM BURST" ("Enum"), s=w1363, f=State_Type_Definitions,_for_0.26g_versions_and_later_3."True Stop" ("Enum")) -> (s? t:f=w1361:T18)
                n511 = Select(t=w1361, s=w1360, f=State_Type_Definitions,_for_0.26g_versions_and_later_3."Task 6A: RAISE ARM" ("Enum")) -> (s? t:f=w1369:T18)
              }
              frame "Exit" {
                n512 = for {
                  shift-right: [w1388] -> w1385
                  shift-left: _ -> [w1389]
                  tunnel: string[] ["STOP", "RESET ENCODERS", "RESET YAW", "ARDUINO MODE 0"] -> [w1387] mode=indexing
                  n513 = Enqueue Element(queue=w1389, element=w1387) -> (queue out=w1388:refnum<queue>)  [unwired: 2 in, 2 out]
                }
              }
            }
          }
          frame "Task 6B: CAM BURST" {
            # ">> Manual override >>"
            # ">>> Motor control cluster >>>"
            # ">>> yStepper command>>>"
            n514 = Dequeue Element(queue=w1401, timeout in ms (-1)=w1399, error in (no error)=w1400) -> (element=w1398:T10)  [unwired: 3 out]
            n515 = case shown="\"Start Task 1\", Default" w1398 {
              tunnel: [w1409 State_Type_Definitions,_for_0.26g_versions_and_later_3."True Stop" ("Enum")] -> w1395
              tunnel: [w1407 w1427] -> w1402
              tunnel: [State_Type_Definitions,_for_0.26g_versions_and_later_3."Idle" ("Enum") State_Type_Definitions,_for_0.26g_versions_and_later_3."Shutdown" ("Enum")] -> w1396
              tunnel: w1397 -> [w1405 _]
              tunnel: w1394 -> [w1406 w1424]
              tunnel: w1390 -> [w1403 _]
              frame "Start Task 1", Default {
                n516 = Or(x=w1403, y=w1405) -> (x .or. y?=w1404:bool)
                n517 = case shown="True" w1404 {
                  tunnel: [w1414 w1420] -> w1407
                  tunnel: w1406 -> [w1412 w1418]
                  frame False {
                    n518 = for {
                      tunnel: string[] ["CAM ACQ", "START TIMER"] ("element") -> [w1415] mode=indexing
                      shift-right: [w1417] -> w1414
                      shift-left: w1412 -> [w1416]
                      n519 = Enqueue Element(queue=w1416, element=w1415) -> (queue out=w1417:refnum<queue>)  [unwired: 2 in, 2 out]
                    }
                  }
                  frame True {
                    n520 = for {
                      shift-right: [w1422] -> w1420
                      shift-left: w1418 -> [w1423]
                      tunnel: string[] ["CAM CLOSE", "PROCESS IMAGE", "SET TIMER 2", "RESET ENCODERS"] -> [w1421] mode=indexing
                      n521 = Enqueue Element(queue=w1423, element=w1421) -> (queue out=w1422:refnum<queue>)  [unwired: 2 in, 2 out]
                    }
                  }
                }
                n522 = Select(t=State_Type_Definitions,_for_0.26g_versions_and_later_3."Task 6C: PROCESS IMAGE" ("Enum"), s=w1404, f=State_Type_Definitions,_for_0.26g_versions_and_later_3."Task 6B: CAM BURST" ("Enum")) -> (s? t:f=w1409:T18)
              }
              frame "Exit" {
                # ">> State after true stop >>"
                # ">> Goes to true stop >>"
                n523 = for {
                  shift-right: [w1430] -> w1427
                  shift-left: w1424 -> [w1431]
                  tunnel: string[] ["STOP", "RESET ENCODERS", "RESET YAW", ""] -> [w1429] mode=indexing
                  n524 = Enqueue Element(queue=w1431, element=w1429) -> (queue out=w1430:refnum<queue>)  [unwired: 2 in, 2 out]
                }
              }
            }
          }
          frame "Task 6C: PROCESS IMAGE" {
            # "Ball > Soap > Gel > Pipe"
            # ">>> Motor control cluster >>>"
            # ">>> yStepper command>>>"
            n525 = Dequeue Element(queue=w1440, timeout in ms (-1)=w1439, error in (no error)=w1438) -> (element=w1437:T10)  [unwired: 3 out]
            n526 = case shown="\"Start Task 1\", Default" w1437 {
              tunnel: [w1456 State_Type_Definitions,_for_0.26g_versions_and_later_3."True Stop" ("Enum")] -> w1444
              tunnel: [w1458 w1475] -> w1443
              tunnel: [State_Type_Definitions,_for_0.26g_versions_and_later_3."Idle" ("Enum") State_Type_Definitions,_for_0.26g_versions_and_later_3."Shutdown" ("Enum")] -> w1445
              tunnel: w1441 -> [w1447 _]
              tunnel: w1442 -> [w1453 w1472]
              tunnel: w1433 -> [w1451 _]
              tunnel: w1432 -> [w1452 _]
              frame "Start Task 1", Default {
                # "Stays in Task 5D until the object is detected"
                n527 = Or(x=w1451, y=w1447) -> (x .or. y?=w1450:bool)
                n528 = case shown="True" w1450 {
                  tunnel: [w1462 w1468] -> w1458
                  tunnel: w1453 -> [w1460 w1466]
                  frame False {
                    n529 = for {
                      tunnel: string[] ["START TIMER", "PROCESS IMAGE", ""] ("element") -> [w1463] mode=indexing
                      shift-right: [w1465] -> w1462
                      shift-left: w1460 -> [w1464]
                      n530 = Enqueue Element(queue=w1464, element=w1463) -> (queue out=w1465:refnum<queue>)  [unwired: 2 in, 2 out]
                    }
                  }
                  frame True {
                    n531 = for {
                      shift-right: [w1470] -> w1468
                      shift-left: w1466 -> [w1471]
                      tunnel: string[] ["RESET ENCODERS", "RESET YAW", ""] -> [w1469] mode=indexing
                      n532 = Enqueue Element(queue=w1471, element=w1469) -> (queue out=w1470:refnum<queue>)  [unwired: 2 in, 2 out]
                    }
                  }
                }
                n533 = Select(t=State_Type_Definitions,_for_0.26g_versions_and_later_3."Task 6D: BALL BUSTER" ("Enum"), s=w1452, f=State_Type_Definitions,_for_0.26g_versions_and_later_3."Task 6F: CAM BURST 2" ("Enum")) -> (s? t:f=w1448:T18)
                n534 = Select(t=State_Type_Definitions,_for_0.26g_versions_and_later_3."True Stop" ("Enum"), s=w1447, f=w1448) -> (s? t:f=w1454:T18)
                n535 = Select(t=w1454, s=w1450, f=State_Type_Definitions,_for_0.26g_versions_and_later_3."Task 6C: PROCESS IMAGE" ("Enum")) -> (s? t:f=w1456:T18)
              }
              frame "Exit" {
                n536 = for {
                  shift-right: [w1478] -> w1475
                  shift-left: w1472 -> [w1479]
                  tunnel: string[] ["STOP", "RESET ENCODERS", "RESET YAW", "ARDUINO MODE 0"] -> [w1477] mode=indexing
                  n537 = Enqueue Element(queue=w1479, element=w1477) -> (queue out=w1478:refnum<queue>)  [unwired: 2 in, 2 out]
                }
              }
            }
          }
          frame "Task 6D: BALL BUSTER" {
            # "Ball > Soap > Gel > Pipe"
            # ">>> Motor control cluster >>>"
            # ">>> yStepper command>>>"
            n538 = Greater Or Equal?(x=w1480, y=20.0) -> (x >= y?=w1481:bool)
            n539 = Dequeue Element(queue=w1489, timeout in ms (-1)=w1488, error in (no error)=w1487) -> (element=w1486:T10)  [unwired: 3 out]
            n540 = case shown="\"Start Task 1\", Default" w1486 {
              tunnel: [w1502 State_Type_Definitions,_for_0.26g_versions_and_later_3."True Stop" ("Enum")] -> w1493
              tunnel: [w1504 w1521] -> w1492
              tunnel: [State_Type_Definitions,_for_0.26g_versions_and_later_3."Idle" ("Enum") State_Type_Definitions,_for_0.26g_versions_and_later_3."Shutdown" ("Enum")] -> w1494
              tunnel: w1490 -> [w1497 _]
              tunnel: w1491 -> [w1499 w1518]
              tunnel: w1481 -> [w1496 _]
              frame "Start Task 1", Default {
                # "Stays in Task 5D until the object is detected"
                n541 = Or(x=w1496, y=w1497) -> (x .or. y?=w1498:bool)
                n542 = case shown="False" w1498 {
                  tunnel: [w1508 w1514] -> w1504
                  tunnel: w1499 -> [w1506 w1512]
                  frame False {
                    n543 = for {
                      tunnel: string[] ["RIGHT", "READ NAVX", "READ ENCODERS"] ("element") -> [w1509] mode=indexing
                      shift-right: [w1511] -> w1508
                      shift-left: w1506 -> [w1510]
                      n544 = Enqueue Element(queue=w1510, element=w1509) -> (queue out=w1511:refnum<queue>)  [unwired: 2 in, 2 out]
                    }
                  }
                  frame True {
                    n545 = for {
                      shift-right: [w1516] -> w1514
                      shift-left: w1512 -> [w1517]
                      tunnel: string[] ["RESET ENCODERS", "RESET YAW", "RESET FLAGS"] -> [w1515] mode=indexing
                      n546 = Enqueue Element(queue=w1517, element=w1515) -> (queue out=w1516:refnum<queue>)  [unwired: 2 in, 2 out]
                    }
                  }
                }
                n547 = Select(t=State_Type_Definitions,_for_0.26g_versions_and_later_3."True Stop" ("Enum"), s=w1497, f=State_Type_Definitions,_for_0.26g_versions_and_later_3."Task 6E: STILL WAITING" ("Enum")) -> (s? t:f=w1500:T18)
                n548 = Select(t=w1500, s=w1498, f=State_Type_Definitions,_for_0.26g_versions_and_later_3."Task 6D: BALL BUSTER" ("Enum")) -> (s? t:f=w1502:T18)
              }
              frame "Exit" {
                n549 = for {
                  shift-right: [w1524] -> w1521
                  shift-left: w1518 -> [w1525]
                  tunnel: string[] ["STOP", "RESET ENCODERS", "RESET YAW", "ARDUINO MODE 0"] -> [w1523] mode=indexing
                  n550 = Enqueue Element(queue=w1525, element=w1523) -> (queue out=w1524:refnum<queue>)  [unwired: 2 in, 2 out]
                }
              }
            }
          }
          frame "Task 6E: STILL WAITING" {
            # "Ball > Soap > Gel > Pipe"
            # ">>> Motor control cluster >>>"
            # ">>> yStepper command>>>"
            n551 = local read "Rising Edge"() -> (w1527:bool)
            n552 = Dequeue Element(queue=w1533, timeout in ms (-1)=w1532, error in (no error)=w1531) -> (element=w1530:T10)  [unwired: 3 out]
            n553 = case shown="\"Start Task 1\", Default" w1530 {
              tunnel: [w1547 State_Type_Definitions,_for_0.26g_versions_and_later_3."True Stop" ("Enum")] -> w1537
              tunnel: [w1540 w1565] -> w1536
              tunnel: [State_Type_Definitions,_for_0.26g_versions_and_later_3."Idle" ("Enum") State_Type_Definitions,_for_0.26g_versions_and_later_3."Shutdown" ("Enum")] -> w1538
              tunnel: w1534 -> [w1544 _]
              tunnel: w1535 -> [w1541 w1562]
              tunnel: w1527 -> [w1542 _]
              frame "Start Task 1", Default {
                # "Stays in Task 5D until the object is detected"
                n554 = Or(x=w1542, y=w1544) -> (x .or. y?=w1539:bool)
                n555 = case shown="False" w1539 {
                  tunnel: [w1552 w1558] -> w1540
                  tunnel: w1541 -> [w1550 w1557]
                  frame False {
                    n556 = for {
                      tunnel: string[] ["Z STEPPER CAM HEIGHT", "READ STEPPER VALUES"] ("element") -> [w1553] mode=indexing
                      shift-right: [w1555] -> w1552
                      shift-left: w1550 -> [w1554]
                      n557 = Enqueue Element(queue=w1554, element=w1553) -> (queue out=w1555:refnum<queue>)  [unwired: 2 in, 2 out]
                    }
                  }
                  frame True {
                    n558 = for {
                      shift-right: [w1560] -> w1558
                      shift-left: w1557 -> [w1561]
                      tunnel: string[] ["OPEN LOG CAM", "SET TIMER 2", "OPEN IMAQ REF", "", ""] -> [w1559] mode=indexing
                      n559 = Enqueue Element(queue=w1561, element=w1559) -> (queue out=w1560:refnum<queue>)  [unwired: 2 in, 2 out]
                    }
                  }
                }
                n560 = Select(t=State_Type_Definitions,_for_0.26g_versions_and_later_3."True Stop" ("Enum"), s=w1544, f=State_Type_Definitions,_for_0.26g_versions_and_later_3."Task 6F: CAM BURST 2" ("Enum")) -> (s? t:f=w1545:T18)
                n561 = Select(t=w1545, s=w1539, f=State_Type_Definitions,_for_0.26g_versions_and_later_3."Task 6E: STILL WAITING" ("Enum")) -> (s? t:f=w1547:T18)
              }
              frame "Exit" {
                n562 = for {
                  shift-right: [w1568] -> w1565
                  shift-left: w1562 -> [w1569]
                  tunnel: string[] ["STOP", "RESET ENCODERS", "RESET YAW", "ARDUINO MODE 0"] -> [w1567] mode=indexing
                  n563 = Enqueue Element(queue=w1569, element=w1567) -> (queue out=w1568:refnum<queue>)  [unwired: 2 in, 2 out]
                }
              }
            }
          }
          frame "Task 6F: CAM BURST 2" {
            # ">> Manual override >>"
            # ">>> Motor control cluster >>>"
            # ">>> yStepper command>>>"
            n564 = Dequeue Element(queue=w1581, timeout in ms (-1)=w1579, error in (no error)=w1580) -> (element=w1578:T10)  [unwired: 3 out]
            n565 = case shown="\"Start Task 1\", Default" w1578 {
              tunnel: [w1589 State_Type_Definitions,_for_0.26g_versions_and_later_3."True Stop" ("Enum")] -> w1575
              tunnel: [w1587 w1607] -> w1582
              tunnel: [State_Type_Definitions,_for_0.26g_versions_and_later_3."Idle" ("Enum") State_Type_Definitions,_for_0.26g_versions_and_later_3."Shutdown" ("Enum")] -> w1576
              tunnel: w1577 -> [w1585 _]
              tunnel: w1574 -> [w1586 w1604]
              tunnel: w1570 -> [w1583 _]
              frame "Start Task 1", Default {
                n566 = Or(x=w1583, y=w1585) -> (x .or. y?=w1584:bool)
                n567 = case shown="True" w1584 {
                  tunnel: [w1594 w1600] -> w1587
                  tunnel: w1586 -> [w1592 w1598]
                  frame False {
                    n568 = for {
                      tunnel: string[] ["CAM ACQ", "START TIMER"] ("element") -> [w1595] mode=indexing
                      shift-right: [w1597] -> w1594
                      shift-left: w1592 -> [w1596]
                      n569 = Enqueue Element(queue=w1596, element=w1595) -> (queue out=w1597:refnum<queue>)  [unwired: 2 in, 2 out]
                    }
                  }
                  frame True {
                    n570 = for {
                      shift-right: [w1602] -> w1600
                      shift-left: w1598 -> [w1603]
                      tunnel: string[] ["CAM CLOSE", "PROCESS IMAGE", "SET TIMER 2", "RESET ENCODERS"] -> [w1601] mode=indexing
                      n571 = Enqueue Element(queue=w1603, element=w1601) -> (queue out=w1602:refnum<queue>)  [unwired: 2 in, 2 out]
                    }
                  }
                }
                n572 = Select(t=State_Type_Definitions,_for_0.26g_versions_and_later_3."Task 6G: PROCESS IMAGE 2" ("Enum"), s=w1584, f=State_Type_Definitions,_for_0.26g_versions_and_later_3."Task 6F: CAM BURST 2" ("Enum")) -> (s? t:f=w1589:T18)
              }
              frame "Exit" {
                # ">> State after true stop >>"
                # ">> Goes to true stop >>"
                n573 = for {
                  shift-right: [w1610] -> w1607
                  shift-left: w1604 -> [w1611]
                  tunnel: string[] ["STOP", "RESET ENCODERS", "RESET YAW", ""] -> [w1609] mode=indexing
                  n574 = Enqueue Element(queue=w1611, element=w1609) -> (queue out=w1610:refnum<queue>)  [unwired: 2 in, 2 out]
                }
              }
            }
          }
          frame "Task 6G: PROCESS IMAGE 2" {
            # "Ball > Soap > Gel > Pipe"
            # ">>> Motor control cluster >>>"
            # ">>> yStepper command>>>"
            n575 = Dequeue Element(queue=w1620, timeout in ms (-1)=w1619, error in (no error)=w1618) -> (element=w1617:T10)  [unwired: 3 out]
            n576 = case shown="\"Start Task 1\", Default" w1617 {
              tunnel: [w1636 State_Type_Definitions,_for_0.26g_versions_and_later_3."True Stop" ("Enum")] -> w1624
              tunnel: [w1638 w1655] -> w1623
              tunnel: [State_Type_Definitions,_for_0.26g_versions_and_later_3."Idle" ("Enum") State_Type_Definitions,_for_0.26g_versions_and_later_3."Shutdown" ("Enum")] -> w1625
              tunnel: w1621 -> [w1627 _]
              tunnel: w1622 -> [w1633 w1652]
              tunnel: w1613 -> [w1631 _]
              tunnel: w1612 -> [w1632 _]
              frame "Start Task 1", Default {
                # "Stays in Task 5D until the object is detected"
                n577 = Or(x=w1631, y=w1627) -> (x .or. y?=w1630:bool)
                n578 = case shown="True" w1630 {
                  tunnel: [w1642 w1648] -> w1638
                  tunnel: w1633 -> [w1640 w1646]
                  frame False {
                    n579 = for {
                      tunnel: string[] ["START TIMER", "PROCESS IMAGE", ""] ("element") -> [w1643] mode=indexing
                      shift-right: [w1645] -> w1642
                      shift-left: w1640 -> [w1644]
                      n580 = Enqueue Element(queue=w1644, element=w1643) -> (queue out=w1645:refnum<queue>)  [unwired: 2 in, 2 out]
                    }
                  }
                  frame True {
                    n581 = for {
                      shift-right: [w1650] -> w1648
                      shift-left: w1646 -> [w1651]
                      tunnel: string[] ["RESET ENCODERS", "RESET YAW", ""] -> [w1649] mode=indexing
                      n582 = Enqueue Element(queue=w1651, element=w1649) -> (queue out=w1650:refnum<queue>)  [unwired: 2 in, 2 out]
                    }
                  }
                }
                n583 = Select(t=State_Type_Definitions,_for_0.26g_versions_and_later_3."Task 6H: SKADI SOAPS" ("Enum"), s=w1632, f=State_Type_Definitions,_for_0.26g_versions_and_later_3."Task 6J: CAM BURST 3" ("Enum")) -> (s? t:f=w1628:T18)
                n584 = Select(t=State_Type_Definitions,_for_0.26g_versions_and_later_3."True Stop" ("Enum"), s=w1627, f=w1628) -> (s? t:f=w1634:T18)
                n585 = Select(t=w1634, s=w1630, f=State_Type_Definitions,_for_0.26g_versions_and_later_3."Task 6G: PROCESS IMAGE 2" ("Enum")) -> (s? t:f=w1636:T18)
              }
              frame "Exit" {
                n586 = for {
                  shift-right: [w1658] -> w1655
                  shift-left: w1652 -> [w1659]
                  tunnel: string[] ["STOP", "RESET ENCODERS", "RESET YAW", "ARDUINO MODE 0"] -> [w1657] mode=indexing
                  n587 = Enqueue Element(queue=w1659, element=w1657) -> (queue out=w1658:refnum<queue>)  [unwired: 2 in, 2 out]
                }
              }
            }
          }
          frame "Task 6H: SKADI SOAPS" {
            # "Ball > Soap > Gel > Pipe"
            # ">>> Motor control cluster >>>"
            # ">>> yStepper command>>>"
            n588 = Less Or Equal?(x=w1660, y=-20.0) -> (x <= y?=w1661:bool)
            n589 = Dequeue Element(queue=w1669, timeout in ms (-1)=w1668, error in (no error)=w1667) -> (element=w1666:T10)  [unwired: 3 out]
            n590 = case shown="\"Start Task 1\", Default" w1666 {
              tunnel: [w1682 State_Type_Definitions,_for_0.26g_versions_and_later_3."True Stop" ("Enum")] -> w1673
              tunnel: [w1684 w1701] -> w1672
              tunnel: [State_Type_Definitions,_for_0.26g_versions_and_later_3."Idle" ("Enum") State_Type_Definitions,_for_0.26g_versions_and_later_3."Shutdown" ("Enum")] -> w1674
              tunnel: w1670 -> [w1677 _]
              tunnel: w1671 -> [w1679 w1698]
              tunnel: w1661 -> [w1676 _]
              frame "Start Task 1", Default {
                # "Stays in Task 5D until the object is detected"
                n591 = Or(x=w1676, y=w1677) -> (x .or. y?=w1678:bool)
                n592 = case shown="False" w1678 {
                  tunnel: [w1688 w1694] -> w1684
                  tunnel: w1679 -> [w1686 w1692]
                  frame False {
                    n593 = for {
                      tunnel: string[] ["LEFT", "READ NAVX", "READ ENCODERS"] ("element") -> [w1689] mode=indexing
                      shift-right: [w1691] -> w1688
                      shift-left: w1686 -> [w1690]
                      n594 = Enqueue Element(queue=w1690, element=w1689) -> (queue out=w1691:refnum<queue>)  [unwired: 2 in, 2 out]
                    }
                  }
                  frame True {
                    n595 = for {
                      shift-right: [w1696] -> w1694
                      shift-left: w1692 -> [w1697]
                      tunnel: string[] ["RESET ENCODERS", "RESET YAW", "RESET FLAGS"] -> [w1695] mode=indexing
                      n596 = Enqueue Element(queue=w1697, element=w1695) -> (queue out=w1696:refnum<queue>)  [unwired: 2 in, 2 out]
                    }
                  }
                }
                n597 = Select(t=State_Type_Definitions,_for_0.26g_versions_and_later_3."True Stop" ("Enum"), s=w1677, f=State_Type_Definitions,_for_0.26g_versions_and_later_3."Task 6I: STILL WAITING 2" ("Enum")) -> (s? t:f=w1680:T18)
                n598 = Select(t=w1680, s=w1678, f=State_Type_Definitions,_for_0.26g_versions_and_later_3."Task 6H: SKADI SOAPS" ("Enum")) -> (s? t:f=w1682:T18)
              }
              frame "Exit" {
                n599 = for {
                  shift-right: [w1704] -> w1701
                  shift-left: w1698 -> [w1705]
                  tunnel: string[] ["STOP", "RESET ENCODERS", "RESET YAW", "ARDUINO MODE 0"] -> [w1703] mode=indexing
                  n600 = Enqueue Element(queue=w1705, element=w1703) -> (queue out=w1704:refnum<queue>)  [unwired: 2 in, 2 out]
                }
              }
            }
          }
          frame "Task 6I: STILL WAITING 2" {
            # "Ball > Soap > Gel > Pipe"
            # ">>> Motor control cluster >>>"
            # ">>> yStepper command>>>"
            n601 = local read "Rising Edge"() -> (w1707:bool)
            n602 = Dequeue Element(queue=w1713, timeout in ms (-1)=w1712, error in (no error)=w1711) -> (element=w1710:T10)  [unwired: 3 out]
            n603 = case shown="\"Start Task 1\", Default" w1710 {
              tunnel: [w1727 State_Type_Definitions,_for_0.26g_versions_and_later_3."True Stop" ("Enum")] -> w1717
              tunnel: [w1720 w1745] -> w1716
              tunnel: [State_Type_Definitions,_for_0.26g_versions_and_later_3."Idle" ("Enum") State_Type_Definitions,_for_0.26g_versions_and_later_3."Shutdown" ("Enum")] -> w1718
              tunnel: w1714 -> [w1724 _]
              tunnel: w1715 -> [w1721 w1742]
              tunnel: w1707 -> [w1722 _]
              frame "Start Task 1", Default {
                # "Stays in Task 5D until the object is detected"
                n604 = Or(x=w1722, y=w1724) -> (x .or. y?=w1719:bool)
                n605 = case shown="False" w1719 {
                  tunnel: [w1732 w1738] -> w1720
                  tunnel: w1721 -> [w1730 w1737]
                  frame False {
                    n606 = for {
                      tunnel: string[] ["Z STEPPER CAM HEIGHT", "READ STEPPER VALUES"] ("element") -> [w1733] mode=indexing
                      shift-right: [w1735] -> w1732
                      shift-left: w1730 -> [w1734]
                      n607 = Enqueue Element(queue=w1734, element=w1733) -> (queue out=w1735:refnum<queue>)  [unwired: 2 in, 2 out]
                    }
                  }
                  frame True {
                    n608 = for {
                      shift-right: [w1740] -> w1738
                      shift-left: w1737 -> [w1741]
                      tunnel: string[] ["OPEN LOG CAM", "SET TIMER 2", "OPEN IMAQ REF", "", ""] -> [w1739] mode=indexing
                      n609 = Enqueue Element(queue=w1741, element=w1739) -> (queue out=w1740:refnum<queue>)  [unwired: 2 in, 2 out]
                    }
                  }
                }
                n610 = Select(t=State_Type_Definitions,_for_0.26g_versions_and_later_3."True Stop" ("Enum"), s=w1724, f=State_Type_Definitions,_for_0.26g_versions_and_later_3."Task 6J: CAM BURST 3" ("Enum")) -> (s? t:f=w1725:T18)
                n611 = Select(t=w1725, s=w1719, f=State_Type_Definitions,_for_0.26g_versions_and_later_3."Task 6I: STILL WAITING 2" ("Enum")) -> (s? t:f=w1727:T18)
              }
              frame "Exit" {
                n612 = for {
                  shift-right: [w1748] -> w1745
                  shift-left: w1742 -> [w1749]
                  tunnel: string[] ["STOP", "RESET ENCODERS", "RESET YAW", "ARDUINO MODE 0"] -> [w1747] mode=indexing
                  n613 = Enqueue Element(queue=w1749, element=w1747) -> (queue out=w1748:refnum<queue>)  [unwired: 2 in, 2 out]
                }
              }
            }
          }
          frame "Task 6J: CAM BURST 3" {
            # ">> Manual override >>"
            # ">>> Motor control cluster >>>"
            # ">>> yStepper command>>>"
            n614 = Dequeue Element(queue=w1761, timeout in ms (-1)=w1759, error in (no error)=w1760) -> (element=w1758:T10)  [unwired: 3 out]
            n615 = case shown="\"Start Task 1\", Default" w1758 {
              tunnel: [w1769 State_Type_Definitions,_for_0.26g_versions_and_later_3."True Stop" ("Enum")] -> w1755
              tunnel: [w1767 w1787] -> w1762
              tunnel: [State_Type_Definitions,_for_0.26g_versions_and_later_3."Idle" ("Enum") State_Type_Definitions,_for_0.26g_versions_and_later_3."Shutdown" ("Enum")] -> w1756
              tunnel: w1757 -> [w1765 _]
              tunnel: w1754 -> [w1766 w1784]
              tunnel: w1750 -> [w1763 _]
              frame "Start Task 1", Default {
                n616 = Or(x=w1763, y=w1765) -> (x .or. y?=w1764:bool)
                n617 = case shown="True" w1764 {
                  tunnel: [w1774 w1780] -> w1767
                  tunnel: w1766 -> [w1772 w1778]
                  frame False {
                    n618 = for {
                      tunnel: string[] ["CAM ACQ", "START TIMER"] ("element") -> [w1775] mode=indexing
                      shift-right: [w1777] -> w1774
                      shift-left: w1772 -> [w1776]
                      n619 = Enqueue Element(queue=w1776, element=w1775) -> (queue out=w1777:refnum<queue>)  [unwired: 2 in, 2 out]
                    }
                  }
                  frame True {
                    n620 = for {
                      shift-right: [w1782] -> w1780
                      shift-left: w1778 -> [w1783]
                      tunnel: string[] ["CAM CLOSE", "PROCESS IMAGE", "SET TIMER 2", "RESET ENCODERS"] -> [w1781] mode=indexing
                      n621 = Enqueue Element(queue=w1783, element=w1781) -> (queue out=w1782:refnum<queue>)  [unwired: 2 in, 2 out]
                    }
                  }
                }
                n622 = Select(t=State_Type_Definitions,_for_0.26g_versions_and_later_3."Task 6K: PROCESS IMAGE 3" ("Enum"), s=w1764, f=State_Type_Definitions,_for_0.26g_versions_and_later_3."Task 6J: CAM BURST 3" ("Enum")) -> (s? t:f=w1769:T18)
              }
              frame "Exit" {
                # ">> State after true stop >>"
                # ">> Goes to true stop >>"
                n623 = for {
                  shift-right: [w1790] -> w1787
                  shift-left: w1784 -> [w1791]
                  tunnel: string[] ["STOP", "RESET ENCODERS", "RESET YAW", ""] -> [w1789] mode=indexing
                  n624 = Enqueue Element(queue=w1791, element=w1789) -> (queue out=w1790:refnum<queue>)  [unwired: 2 in, 2 out]
                }
              }
            }
          }
          frame "Task 6K: PROCESS IMAGE 3" {
            # "Ball > Soap > Gel > Pipe"
            # ">>> Motor control cluster >>>"
            # ">>> yStepper command>>>"
            n625 = Dequeue Element(queue=w1800, timeout in ms (-1)=w1799, error in (no error)=w1798) -> (element=w1797:T10)  [unwired: 3 out]
            n626 = case shown="\"Start Task 1\", Default" w1797 {
              tunnel: [w1816 State_Type_Definitions,_for_0.26g_versions_and_later_3."True Stop" ("Enum")] -> w1804
              tunnel: [w1818 w1835] -> w1803
              tunnel: [State_Type_Definitions,_for_0.26g_versions_and_later_3."Idle" ("Enum") State_Type_Definitions,_for_0.26g_versions_and_later_3."Shutdown" ("Enum")] -> w1805
              tunnel: w1801 -> [w1807 _]
              tunnel: w1802 -> [w1813 w1832]
              tunnel: w1793 -> [w1811 _]
              tunnel: w1792 -> [w1812 _]
              frame "Start Task 1", Default {
                # "Stays in Task 5D until the object is detected"
                n627 = Or(x=w1811, y=w1807) -> (x .or. y?=w1810:bool)
                n628 = case shown="True" w1810 {
                  tunnel: [w1822 w1828] -> w1818
                  tunnel: w1813 -> [w1820 w1826]
                  frame False {
                    n629 = for {
                      tunnel: string[] ["START TIMER", "PROCESS IMAGE", ""] ("element") -> [w1823] mode=indexing
                      shift-right: [w1825] -> w1822
                      shift-left: w1820 -> [w1824]
                      n630 = Enqueue Element(queue=w1824, element=w1823) -> (queue out=w1825:refnum<queue>)  [unwired: 2 in, 2 out]
                    }
                  }
                  frame True {
                    n631 = for {
                      shift-right: [w1830] -> w1828
                      shift-left: w1826 -> [w1831]
                      tunnel: string[] ["RESET ENCODERS", "RESET YAW", ""] -> [w1829] mode=indexing
                      n632 = Enqueue Element(queue=w1831, element=w1829) -> (queue out=w1830:refnum<queue>)  [unwired: 2 in, 2 out]
                    }
                  }
                }
                n633 = Select(t=State_Type_Definitions,_for_0.26g_versions_and_later_3."Task 6L: JAM IT IN" ("Enum"), s=w1812, f=State_Type_Definitions,_for_0.26g_versions_and_later_3."Task 6N: CAM BURST 4" ("Enum")) -> (s? t:f=w1808:T18)
                n634 = Select(t=State_Type_Definitions,_for_0.26g_versions_and_later_3."True Stop" ("Enum"), s=w1807, f=w1808) -> (s? t:f=w1814:T18)
                n635 = Select(t=w1814, s=w1810, f=State_Type_Definitions,_for_0.26g_versions_and_later_3."Task 6K: PROCESS IMAGE 3" ("Enum")) -> (s? t:f=w1816:T18)
              }
              frame "Exit" {
                n636 = for {
                  shift-right: [w1838] -> w1835
                  shift-left: w1832 -> [w1839]
                  tunnel: string[] ["STOP", "RESET ENCODERS", "RESET YAW", "ARDUINO MODE 0"] -> [w1837] mode=indexing
                  n637 = Enqueue Element(queue=w1839, element=w1837) -> (queue out=w1838:refnum<queue>)  [unwired: 2 in, 2 out]
                }
              }
            }
          }
          frame "Task 6L: JAM IT IN" {
            # "Ball > Soap > Gel > Pipe"
            # ">>> Motor control cluster >>>"
            # ">>> yStepper command>>>"
            n638 = Less Or Equal?(x=w1840, y=-20.0) -> (x <= y?=w1841:bool)
            n639 = Dequeue Element(queue=w1849, timeout in ms (-1)=w1848, error in (no error)=w1847) -> (element=w1846:T10)  [unwired: 3 out]
            n640 = case shown="\"Start Task 1\", Default" w1846 {
              tunnel: [w1862 State_Type_Definitions,_for_0.26g_versions_and_later_3."True Stop" ("Enum")] -> w1853
              tunnel: [w1864 w1881] -> w1852
              tunnel: [State_Type_Definitions,_for_0.26g_versions_and_later_3."Idle" ("Enum") State_Type_Definitions,_for_0.26g_versions_and_later_3."Shutdown" ("Enum")] -> w1854
              tunnel: w1850 -> [w1857 _]
              tunnel: w1851 -> [w1859 w1878]
              tunnel: w1841 -> [w1856 _]
              frame "Start Task 1", Default {
                # "Stays in Task 5D until the object is detected"
                n641 = Or(x=w1856, y=w1857) -> (x .or. y?=w1858:bool)
                n642 = case shown="False" w1858 {
                  tunnel: [w1868 w1874] -> w1864
                  tunnel: w1859 -> [w1866 w1872]
                  frame False {
                    n643 = for {
                      tunnel: string[] ["REVERSE", "READ NAVX", "READ ENCODERS"] ("element") -> [w1869] mode=indexing
                      shift-right: [w1871] -> w1868
                      shift-left: w1866 -> [w1870]
                      n644 = Enqueue Element(queue=w1870, element=w1869) -> (queue out=w1871:refnum<queue>)  [unwired: 2 in, 2 out]
                    }
                  }
                  frame True {
                    n645 = for {
                      shift-right: [w1876] -> w1874
                      shift-left: w1872 -> [w1877]
                      tunnel: string[] ["RESET ENCODERS", "RESET YAW", "RESET FLAGS"] -> [w1875] mode=indexing
                      n646 = Enqueue Element(queue=w1877, element=w1875) -> (queue out=w1876:refnum<queue>)  [unwired: 2 in, 2 out]
                    }
                  }
                }
                n647 = Select(t=State_Type_Definitions,_for_0.26g_versions_and_later_3."True Stop" ("Enum"), s=w1857, f=State_Type_Definitions,_for_0.26g_versions_and_later_3."Task 6M: STILL WAITING 3" ("Enum")) -> (s? t:f=w1860:T18)
                n648 = Select(t=w1860, s=w1858, f=State_Type_Definitions,_for_0.26g_versions_and_later_3."Task 6L: JAM IT IN" ("Enum")) -> (s? t:f=w1862:T18)
              }
              frame "Exit" {
                n649 = for {
                  shift-right: [w1884] -> w1881
                  shift-left: w1878 -> [w1885]
                  tunnel: string[] ["STOP", "RESET ENCODERS", "RESET YAW", "ARDUINO MODE 0"] -> [w1883] mode=indexing
                  n650 = Enqueue Element(queue=w1885, element=w1883) -> (queue out=w1884:refnum<queue>)  [unwired: 2 in, 2 out]
                }
              }
            }
          }
          frame "Task 6M: STILL WAITING 3" {
            # "Ball > Soap > Gel > Pipe"
            # ">>> Motor control cluster >>>"
            # ">>> yStepper command>>>"
            n651 = local read "Rising Edge"() -> (w1887:bool)
            n652 = Dequeue Element(queue=w1893, timeout in ms (-1)=w1892, error in (no error)=w1891) -> (element=w1890:T10)  [unwired: 3 out]
            n653 = case shown="\"Start Task 1\", Default" w1890 {
              tunnel: [w1907 State_Type_Definitions,_for_0.26g_versions_and_later_3."True Stop" ("Enum")] -> w1897
              tunnel: [w1900 w1925] -> w1896
              tunnel: [State_Type_Definitions,_for_0.26g_versions_and_later_3."Idle" ("Enum") State_Type_Definitions,_for_0.26g_versions_and_later_3."Shutdown" ("Enum")] -> w1898
              tunnel: w1894 -> [w1904 _]
              tunnel: w1895 -> [w1901 w1922]
              tunnel: w1887 -> [w1902 _]
              frame "Start Task 1", Default {
                # "Stays in Task 5D until the object is detected"
                n654 = Or(x=w1902, y=w1904) -> (x .or. y?=w1899:bool)
                n655 = case shown="False" w1899 {
                  tunnel: [w1912 w1918] -> w1900
                  tunnel: w1901 -> [w1910 w1917]
                  frame False {
                    n656 = for {
                      tunnel: string[] ["Z STEPPER CAM HEIGHT", "READ STEPPER VALUES"] ("element") -> [w1913] mode=indexing
                      shift-right: [w1915] -> w1912
                      shift-left: w1910 -> [w1914]
                      n657 = Enqueue Element(queue=w1914, element=w1913) -> (queue out=w1915:refnum<queue>)  [unwired: 2 in, 2 out]
                    }
                  }
                  frame True {
                    n658 = for {
                      shift-right: [w1920] -> w1918
                      shift-left: w1917 -> [w1921]
                      tunnel: string[] ["OPEN LOG CAM", "SET TIMER 2", "OPEN IMAQ REF", "", ""] -> [w1919] mode=indexing
                      n659 = Enqueue Element(queue=w1921, element=w1919) -> (queue out=w1920:refnum<queue>)  [unwired: 2 in, 2 out]
                    }
                  }
                }
                n660 = Select(t=State_Type_Definitions,_for_0.26g_versions_and_later_3."True Stop" ("Enum"), s=w1904, f=State_Type_Definitions,_for_0.26g_versions_and_later_3."Task 6N: CAM BURST 4" ("Enum")) -> (s? t:f=w1905:T18)
                n661 = Select(t=w1905, s=w1899, f=State_Type_Definitions,_for_0.26g_versions_and_later_3."Task 6M: STILL WAITING 3" ("Enum")) -> (s? t:f=w1907:T18)
              }
              frame "Exit" {
                n662 = for {
                  shift-right: [w1928] -> w1925
                  shift-left: w1922 -> [w1929]
                  tunnel: string[] ["STOP", "RESET ENCODERS", "RESET YAW", "ARDUINO MODE 0"] -> [w1927] mode=indexing
                  n663 = Enqueue Element(queue=w1929, element=w1927) -> (queue out=w1928:refnum<queue>)  [unwired: 2 in, 2 out]
                }
              }
            }
          }
          frame "Task 6N: CAM BURST 4" {
            # ">> Manual override >>"
            # ">>> Motor control cluster >>>"
            # ">>> yStepper command>>>"
            n664 = Dequeue Element(queue=w1941, timeout in ms (-1)=w1939, error in (no error)=w1940) -> (element=w1938:T10)  [unwired: 3 out]
            n665 = case shown="\"Start Task 1\", Default" w1938 {
              tunnel: [w1949 State_Type_Definitions,_for_0.26g_versions_and_later_3."True Stop" ("Enum")] -> w1935
              tunnel: [w1947 w1967] -> w1942
              tunnel: [State_Type_Definitions,_for_0.26g_versions_and_later_3."Idle" ("Enum") State_Type_Definitions,_for_0.26g_versions_and_later_3."Shutdown" ("Enum")] -> w1936
              tunnel: w1937 -> [w1945 _]
              tunnel: w1934 -> [w1946 w1964]
              tunnel: w1930 -> [w1943 _]
              frame "Start Task 1", Default {
                n666 = Or(x=w1943, y=w1945) -> (x .or. y?=w1944:bool)
                n667 = case shown="True" w1944 {
                  tunnel: [w1954 w1960] -> w1947
                  tunnel: w1946 -> [w1952 w1958]
                  frame False {
                    n668 = for {
                      tunnel: string[] ["CAM ACQ", "START TIMER"] ("element") -> [w1955] mode=indexing
                      shift-right: [w1957] -> w1954
                      shift-left: w1952 -> [w1956]
                      n669 = Enqueue Element(queue=w1956, element=w1955) -> (queue out=w1957:refnum<queue>)  [unwired: 2 in, 2 out]
                    }
                  }
                  frame True {
                    n670 = for {
                      shift-right: [w1962] -> w1960
                      shift-left: w1958 -> [w1963]
                      tunnel: string[] ["CAM CLOSE", "PROCESS IMAGE", "SET TIMER 2", "RESET ENCODERS"] -> [w1961] mode=indexing
                      n671 = Enqueue Element(queue=w1963, element=w1961) -> (queue out=w1962:refnum<queue>)  [unwired: 2 in, 2 out]
                    }
                  }
                }
                n672 = Select(t=State_Type_Definitions,_for_0.26g_versions_and_later_3."Task 6O: PROCESS IMAGE 4" ("Enum"), s=w1944, f=State_Type_Definitions,_for_0.26g_versions_and_later_3."Task 6N: CAM BURST 4" ("Enum")) -> (s? t:f=w1949:T18)
              }
              frame "Exit" {
                # ">> State after true stop >>"
                # ">> Goes to true stop >>"
                n673 = for {
                  shift-right: [w1970] -> w1967
                  shift-left: w1964 -> [w1971]
                  tunnel: string[] ["STOP", "RESET ENCODERS", "RESET YAW", ""] -> [w1969] mode=indexing
                  n674 = Enqueue Element(queue=w1971, element=w1969) -> (queue out=w1970:refnum<queue>)  [unwired: 2 in, 2 out]
                }
              }
            }
          }
          frame "Task 6O: PROCESS IMAGE 4" {
            # "Ball > Soap > Gel > Pipe"
            # ">>> Motor control cluster >>>"
            # ">>> yStepper command>>>"
            n675 = Dequeue Element(queue=w1980, timeout in ms (-1)=w1979, error in (no error)=w1978) -> (element=w1977:T10)  [unwired: 3 out]
            n676 = case shown="\"Start Task 1\", Default" w1977 {
              tunnel: [w1996 State_Type_Definitions,_for_0.26g_versions_and_later_3."True Stop" ("Enum")] -> w1984
              tunnel: [w1998 w2015] -> w1983
              tunnel: [State_Type_Definitions,_for_0.26g_versions_and_later_3."Idle" ("Enum") State_Type_Definitions,_for_0.26g_versions_and_later_3."Shutdown" ("Enum")] -> w1985
              tunnel: w1981 -> [w1987 _]
              tunnel: w1982 -> [w1993 w2012]
              tunnel: w1973 -> [w1991 _]
              tunnel: w1972 -> [w1992 _]
              frame "Start Task 1", Default {
                # "Stays in Task 5D until the object is detected"
                n677 = Or(x=w1991, y=w1987) -> (x .or. y?=w1990:bool)
                n678 = case shown="True" w1990 {
                  tunnel: [w2002 w2008] -> w1998
                  tunnel: w1993 -> [w2000 w2006]
                  frame False {
                    n679 = for {
                      tunnel: string[] ["START TIMER", "PROCESS IMAGE", ""] ("element") -> [w2003] mode=indexing
                      shift-right: [w2005] -> w2002
                      shift-left: w2000 -> [w2004]
                      n680 = Enqueue Element(queue=w2004, element=w2003) -> (queue out=w2005:refnum<queue>)  [unwired: 2 in, 2 out]
                    }
                  }
                  frame True {
                    n681 = for {
                      shift-right: [w2010] -> w2008
                      shift-left: w2006 -> [w2011]
                      tunnel: string[] ["RESET ENCODERS", "RESET YAW", ""] -> [w2009] mode=indexing
                      n682 = Enqueue Element(queue=w2011, element=w2009) -> (queue out=w2010:refnum<queue>)  [unwired: 2 in, 2 out]
                    }
                  }
                }
                n683 = Select(t=State_Type_Definitions,_for_0.26g_versions_and_later_3."Task 6P: PIPE BOMB" ("Enum"), s=w1992, f=State_Type_Definitions,_for_0.26g_versions_and_later_3."Task 6B: CAM BURST" ("Enum")) -> (s? t:f=w1988:T18)
                n684 = Select(t=State_Type_Definitions,_for_0.26g_versions_and_later_3."True Stop" ("Enum"), s=w1987, f=w1988) -> (s? t:f=w1994:T18)
                n685 = Select(t=w1994, s=w1990, f=State_Type_Definitions,_for_0.26g_versions_and_later_3."Task 6O: PROCESS IMAGE 4" ("Enum")) -> (s? t:f=w1996:T18)
              }
              frame "Exit" {
                n686 = for {
                  shift-right: [w2018] -> w2015
                  shift-left: w2012 -> [w2019]
                  tunnel: string[] ["STOP", "RESET ENCODERS", "RESET YAW", "ARDUINO MODE 0"] -> [w2017] mode=indexing
                  n687 = Enqueue Element(queue=w2019, element=w2017) -> (queue out=w2018:refnum<queue>)  [unwired: 2 in, 2 out]
                }
              }
            }
          }
          frame "Task 6P: PIPE BOMB" {
            # "Ball > Soap > Gel > Pipe"
            # ">>> Motor control cluster >>>"
            # ">>> yStepper command>>>"
            n688 = Greater Or Equal?(x=w2020, y=20.0) -> (x >= y?=w2021:bool)
            n689 = Dequeue Element(queue=w2029, timeout in ms (-1)=w2028, error in (no error)=w2027) -> (element=w2026:T10)  [unwired: 3 out]
            n690 = case shown="\"Start Task 1\", Default" w2026 {
              tunnel: [w2042 State_Type_Definitions,_for_0.26g_versions_and_later_3."True Stop" ("Enum")] -> w2033
              tunnel: [w2044 w2061] -> w2032
              tunnel: [State_Type_Definitions,_for_0.26g_versions_and_later_3."Idle" ("Enum") State_Type_Definitions,_for_0.26g_versions_and_later_3."Shutdown" ("Enum")] -> w2034
              tunnel: w2030 -> [w2037 _]
              tunnel: w2031 -> [w2039 w2058]
              tunnel: w2021 -> [w2036 _]
              frame "Start Task 1", Default {
                # "Stays in Task 5D until the object is detected"
                n691 = Or(x=w2036, y=w2037) -> (x .or. y?=w2038:bool)
                n692 = case shown="False" w2038 {
                  tunnel: [w2048 w2054] -> w2044
                  tunnel: w2039 -> [w2046 w2052]
                  frame False {
                    n693 = for {
                      tunnel: string[] ["FORWARD", "READ NAVX", "READ ENCODERS"] ("element") -> [w2049] mode=indexing
                      shift-right: [w2051] -> w2048
                      shift-left: w2046 -> [w2050]
                      n694 = Enqueue Element(queue=w2050, element=w2049) -> (queue out=w2051:refnum<queue>)  [unwired: 2 in, 2 out]
                    }
                  }
                  frame True {
                    n695 = for {
                      shift-right: [w2056] -> w2054
                      shift-left: w2052 -> [w2057]
                      tunnel: string[] ["RESET ENCODERS", "RESET YAW", "RESET FLAGS"] -> [w2055] mode=indexing
                      n696 = Enqueue Element(queue=w2057, element=w2055) -> (queue out=w2056:refnum<queue>)  [unwired: 2 in, 2 out]
                    }
                  }
                }
                n697 = Select(t=State_Type_Definitions,_for_0.26g_versions_and_later_3."True Stop" ("Enum"), s=w2037, f=State_Type_Definitions,_for_0.26g_versions_and_later_3."Task 5F: ARM GRAB HEIGHT" ("Enum")) -> (s? t:f=w2040:T18)
                n698 = Select(t=w2040, s=w2038, f=State_Type_Definitions,_for_0.26g_versions_and_later_3."Task 6P: PIPE BOMB" ("Enum")) -> (s? t:f=w2042:T18)
              }
              frame "Exit" {
                n699 = for {
                  shift-right: [w2064] -> w2061
                  shift-left: w2058 -> [w2065]
                  tunnel: string[] ["STOP", "RESET ENCODERS", "RESET YAW", "ARDUINO MODE 0"] -> [w2063] mode=indexing
                  n700 = Enqueue Element(queue=w2065, element=w2063) -> (queue out=w2064:refnum<queue>)  [unwired: 2 in, 2 out]
                }
              }
            }
          }
          frame "Task 7" {
          }
          frame "Task 8A: RAISE ARM" {
            # ">>> Motor control cluster >>>"
            # ">>> yStepper command>>>"
            # ">> Manual override >>"
            n701 = Dequeue Element(queue=w2082, timeout in ms (-1)=w2081, error in (no error)=w2083) -> (element=w2080:T10)  [unwired: 3 out]
            n702 = Equal?(x=w2079, y=u8 60) -> (x = y?=w2077:bool)
            n703 = case shown="\"Start Task 1\", Default" w2080 {
              tunnel: [w2093 State_Type_Definitions,_for_0.26g_versions_and_later_3."True Stop" ("Enum")] -> w2084
              tunnel: [w2096 w2113] -> w2085
              tunnel: [State_Type_Definitions,_for_0.26g_versions_and_later_3."Idle" ("Enum") State_Type_Definitions,_for_0.26g_versions_and_later_3."Shutdown" ("Enum")] -> w2086
              tunnel: w2077 -> [w2092 _]
              tunnel: w2076 -> [w2091 _]
              tunnel: w2075 -> [w2087 w2110]
              frame "Start Task 1", Default {
                # "Stays in Task 5_A until stepper reaches desired \nheight"
                # "T: Go back to idle, F: Continue with task\""
                # ">> Manual override >>"
                n704 = case shown="False" w2092 {
                  tunnel: [w2100 w2106] -> w2096
                  tunnel: w2087 -> [w2098 w2104]
                  frame False {
                    n705 = for {
                      tunnel: string[] ["Z STEPPER CAM HEIGHT", "READ STEPPER VALUES", "READ IR"] ("element") -> [w2101] mode=indexing
                      shift-right: [w2103] -> w2100
                      shift-left: w2098 -> [w2102]
                      n706 = Enqueue Element(queue=w2102, element=w2101) -> (queue out=w2103:refnum<queue>)  [unwired: 2 in, 2 out]
                    }
                  }
                  frame True {
                    n707 = for {
                      shift-right: [w2108] -> w2106
                      shift-left: w2104 -> [w2109]
                      tunnel: string[] ["RESET YAW", "RESET ENCODERS", "READ IR"] -> [w2107] mode=indexing
                      n708 = Enqueue Element(queue=w2109, element=w2107) -> (queue out=w2108:refnum<queue>)  [unwired: 2 in, 2 out]
                    }
                  }
                }
                n709 = Or(x=w2092, y=w2091) -> (x .or. y?=w2094:bool)
                n710 = Select(t=State_Type_Definitions,_for_0.26g_versions_and_later_3."True Stop" ("Enum"), s=w2091, f=State_Type_Definitions,_for_0.26g_versions_and_later_3."Task 8B: MOVE TO BOX" ("Enum")) -> (s? t:f=w2088:T18)
                n711 = Select(t=w2088, s=w2094, f=State_Type_Definitions,_for_0.26g_versions_and_later_3."Task 8A: RAISE ARM" ("Enum")) -> (s? t:f=w2093:T18)
              }
              frame "Exit" {
                n712 = for {
                  shift-right: [w2116] -> w2113
                  shift-left: w2110 -> [w2117]
                  tunnel: string[] ["STOP", "RESET ENCODERS", "RESET YAW", "ARDUINO MODE 0"] -> [w2115] mode=indexing
                  n713 = Enqueue Element(queue=w2117, element=w2115) -> (queue out=w2116:refnum<queue>)  [unwired: 2 in, 2 out]
                }
              }
            }
          }
          frame "Task 8B: MOVE TO BOX" {
            w2127 = u8 15 ("y")
            # "High voltage: 70"
            # ">>> yStepper command>>>"
            n714 = Less?(x=w2124, y=w2127) -> (x < y?=w2125:bool)
            n715 = Less?(x=w2123, y=w2127) -> (x < y?=w2126:bool)
            n716 = And(x=w2126, y=w2125) -> ()  [unwired: 1 out]
            n717 = Dequeue Element(queue=w2131, timeout in ms (-1)=w2130, error in (no error)=w2132) -> (element=w2129:T10)  [unwired: 3 out]
            n718 = Less?(x=w2120, y=40.0) -> (x < y?=w2118:bool)
            n719 = case shown="\"Start Task 1\", Default" w2129 {
              tunnel: [w2144 State_Type_Definitions,_for_0.26g_versions_and_later_3."True Stop" ("Enum")] -> w2134
              tunnel: [w2147 w2164] -> w2133
              tunnel: [State_Type_Definitions,_for_0.26g_versions_and_later_3."Idle" ("Enum") State_Type_Definitions,_for_0.26g_versions_and_later_3."Shutdown" ("Enum")] -> w2135
              tunnel: w2137 -> [w2143 _]
              tunnel: w2136 -> [w2139 w2161]
              tunnel: w2118 -> [w2138 _]
              frame "Start Task 1", Default {
                # "Stays in Task 5_B to capture image over 5 seconds"
                # "T: Go back to idle, F: Continue with task\""
                # ">> Manual override >>"
                n720 = case shown="True" w2138 {
                  tunnel: [w2151 w2157] -> w2147
                  tunnel: w2139 -> [w2149 w2155]
                  frame False {
                    n721 = for {
                      tunnel: string[] ["FORWARD", "READ IR", "READ NAVX"] ("element") -> [w2152] mode=indexing
                      shift-right: [w2154] -> w2151
                      shift-left: w2149 -> [w2153]
                      n722 = Enqueue Element(queue=w2153, element=w2152) -> (queue out=w2154:refnum<queue>)  [unwired: 2 in, 2 out]
                    }
                  }
                  frame True {
                    n723 = for {
                      shift-right: [w2159] -> w2157
                      shift-left: w2155 -> [w2160]
                      tunnel: string[] ["STOP", "RESET ENCODERS", "OPEN LOG CAM", "SET TIMER 2", "OPEN IMAQ REF"] -> [w2158] mode=indexing
                      n724 = Enqueue Element(queue=w2160, element=w2158) -> (queue out=w2159:refnum<queue>)  [unwired: 2 in, 2 out]
                    }
                  }
                }
                n725 = Or(x=w2138, y=w2143) -> (x .or. y?=w2145:bool)
                n726 = Select(t=State_Type_Definitions,_for_0.26g_versions_and_later_3."True Stop" ("Enum"), s=w2143, f=State_Type_Definitions,_for_0.26g_versions_and_later_3."Task 8C: CAM BURST" ("Enum")) -> (s? t:f=w2140:T18)
                n727 = Select(t=w2140, s=w2145, f=State_Type_Definitions,_for_0.26g_versions_and_later_3."Task 8B: MOVE TO BOX" ("Enum")) -> (s? t:f=w2144:T18)
              }
              frame "Exit" {
                n728 = for {
                  shift-right: [w2167] -> w2164
                  shift-left: w2161 -> [w2168]
                  tunnel: string[] ["STOP", "RESET ENCODERS", "RESET YAW", "ARDUINO MODE 0"] -> [w2166] mode=indexing
                  n729 = Enqueue Element(queue=w2168, element=w2166) -> (queue out=w2167:refnum<queue>)  [unwired: 2 in, 2 out]
                }
              }
            }
          }
          frame "Task 8C: CAM BURST" {
            # ">>> Motor control cluster >>>"
            # ">>> yStepper command>>>"
            # ">> Manual override >>"
            n730 = Dequeue Element(queue=w2179, timeout in ms (-1)=w2178, error in (no error)=w2177) -> (element=w2176:T10)  [unwired: 3 out]
            n731 = case shown="\"Start Task 1\", Default" w2176 {
              tunnel: [w2188 State_Type_Definitions,_for_0.26g_versions_and_later_3."True Stop" ("Enum")] -> w2181
              tunnel: [w2191 w2208] -> w2174
              tunnel: [State_Type_Definitions,_for_0.26g_versions_and_later_3."Idle" ("Enum") State_Type_Definitions,_for_0.26g_versions_and_later_3."Shutdown" ("Enum")] -> w2173
              tunnel: w2175 -> [w2182 _]
              tunnel: w2180 -> [w2187 w2205]
              tunnel: w2171 -> [w2186 _]
              frame "Start Task 1", Default {
                # ">> Is time up? >>"
                # "Determines if object is in range to pick up"
                # ">> Manual override >>"
                n732 = case shown="True" w2186 {
                  tunnel: [w2195 w2201] -> w2191
                  tunnel: w2187 -> [w2193 w2199]
                  frame False {
                    n733 = for {
                      tunnel: string[] ["CAM ACQ", "START TIMER"] ("element") -> [w2196] mode=indexing
                      shift-right: [w2198] -> w2195
                      shift-left: w2193 -> [w2197]
                      n734 = Enqueue Element(queue=w2197, element=w2196) -> (queue out=w2198:refnum<queue>)  [unwired: 2 in, 2 out]
                    }
                  }
                  frame True {
                    n735 = for {
                      shift-right: [w2203] -> w2201
                      shift-left: w2199 -> [w2204]
                      tunnel: string[] ["CAM CLOSE", "PROCESS IMAGE", "SET TIMER 2"] -> [w2202] mode=indexing
                      n736 = Enqueue Element(queue=w2204, element=w2202) -> (queue out=w2203:refnum<queue>)  [unwired: 2 in, 2 out]
                    }
                  }
                }
                n737 = Or(x=w2186, y=w2182) -> (x .or. y?=w2189:bool)
                n738 = Select(t=State_Type_Definitions,_for_0.26g_versions_and_later_3."True Stop" ("Enum"), s=w2182, f=State_Type_Definitions,_for_0.26g_versions_and_later_3."Task 8D: PROCESS IMAGE" ("Enum")) -> (s? t:f=w2184:T18)
                n739 = Select(t=w2184, s=w2189, f=State_Type_Definitions,_for_0.26g_versions_and_later_3."Task 8C: CAM BURST" ("Enum")) -> (s? t:f=w2188:T18)
              }
              frame "Exit" {
                n740 = for {
                  shift-right: [w2211] -> w2208
                  shift-left: w2205 -> [w2212]
                  tunnel: string[] ["STOP", "RESET ENCODERS", "RESET YAW", "ARDUINO MODE 0"] -> [w2210] mode=indexing
                  n741 = Enqueue Element(queue=w2212, element=w2210) -> (queue out=w2211:refnum<queue>)  [unwired: 2 in, 2 out]
                }
              }
            }
          }
          frame "Task 8D: PROCESS IMAGE" {
            # ">>> Motor control cluster >>>"
            # ">>> yStepper command>>>"
            n742 = Dequeue Element(queue=w2221, timeout in ms (-1)=w2220, error in (no error)=w2219) -> (element=w2218:T10)  [unwired: 3 out]
            n743 = case shown="\"Start Task 1\", Default" w2218 {
              tunnel: [w2236 State_Type_Definitions,_for_0.26g_versions_and_later_3."True Stop" ("Enum")] -> w2225
              tunnel: [w2239 w2256] -> w2224
              tunnel: [State_Type_Definitions,_for_0.26g_versions_and_later_3."Idle" ("Enum") State_Type_Definitions,_for_0.26g_versions_and_later_3."Shutdown" ("Enum")] -> w2226
              tunnel: w2222 -> [w2235 _]
              tunnel: w2223 -> [w2232 w2253]
              tunnel: w2213 -> [w2231 _]
              tunnel: w2214 -> [w2230 _]
              frame "Start Task 1", Default {
                # ">> T: Breaks out of state loop; F: Stays in loop>>"
                # ">> Manual override >>"
                # ">> Checks if time is up>>"
                # "Stays in Task 5D until the object is detected"
                # "T: Go back to idle, F: Continue with task\""
                # ">> Manual override >>"
                n744 = case shown="False" w2231 {
                  tunnel: [w2243 w2249] -> w2239
                  tunnel: w2232 -> [w2241 w2247]
                  frame False {
                    n745 = for {
                      tunnel: string[] ["START TIMER", "PROCESS IMAGE", ""] ("element") -> [w2244] mode=indexing
                      shift-right: [w2246] -> w2243
                      shift-left: w2241 -> [w2245]
                      n746 = Enqueue Element(queue=w2245, element=w2244) -> (queue out=w2246:refnum<queue>)  [unwired: 2 in, 2 out]
                    }
                  }
                  frame True {
                    n747 = for {
                      shift-right: [w2251] -> w2249
                      shift-left: w2247 -> [w2252]
                      tunnel: string[] ["RESET ENCODERS", "", ""] -> [w2250] mode=indexing
                      n748 = Enqueue Element(queue=w2252, element=w2250) -> (queue out=w2251:refnum<queue>)  [unwired: 2 in, 2 out]
                    }
                  }
                }
                n749 = Or(x=w2231, y=w2235) -> (x .or. y?=w2237:bool)
                n750 = Select(t=State_Type_Definitions,_for_0.26g_versions_and_later_3."Task 8E: ROBOT ADJUST" ("Enum"), s=w2230, f=State_Type_Definitions,_for_0.26g_versions_and_later_3."True Stop" ("Enum")) -> (s? t:f=w2227:T18)
                n751 = Select(t=State_Type_Definitions,_for_0.26g_versions_and_later_3."True Stop" ("Enum"), s=w2235, f=w2227) -> (s? t:f=w2233:T18)
                n752 = Select(t=w2233, s=w2237, f=State_Type_Definitions,_for_0.26g_versions_and_later_3."Task 8D: PROCESS IMAGE" ("Enum")) -> (s? t:f=w2236:T18)
              }
              frame "Exit" {
                n753 = for {
                  shift-right: [w2259] -> w2256
                  shift-left: w2253 -> [w2260]
                  tunnel: string[] ["STOP", "RESET ENCODERS", "RESET YAW", "ARDUINO MODE 0"] -> [w2258] mode=indexing
                  n754 = Enqueue Element(queue=w2260, element=w2258) -> (queue out=w2259:refnum<queue>)  [unwired: 2 in, 2 out]
                }
              }
            }
          }
          frame "Task 8E: ROBOT ADJUST" {
            # ">>> Motor control cluster >>>"
            # ">>> yStepper command>>>"
            n755 = Dequeue Element(queue=w2277, timeout in ms (-1)=w2276, error in (no error)=w2275) -> (element=w2274:T10)  [unwired: 3 out]
            n756 = Subtract(x=w2272, y=150.0) -> (x-y=w2270:dbl)
            n757 = formula code="if (error >= -100 && error < -80){\n    distance = -25;\n    xSpeed = -30;\n}\n\nelse if (error >= -80 && error < -60){\n    distance = -20;\n    xSpeed = -30;\n}\n\nelse if (error >= -60 && error < -40){\n    distance = -15;\n    xSpeed = -30;\n}\n\nelse if (error >= -40 && error < -20){\n    distance = -10;\n    xSpeed = -30;\n}\n\nelse if (error >= -20 && error < -10){\n    distance = 5;\n    xSpeed = -30;\n}\n\nelse if (error >= -10 && error <= 10){\n    distance = 0;\n    xSpeed = 0;\n}\n\nelse if (error >= 20 && error < 40){\n    distance = 5;\n    xSpeed = 30;\n}\n\nelse if (error >= 40 && error < 60){\n    distance = 10;\n    xSpeed = 30;\n}\n\nelse if (error >= 60 && error < 80){\n    distance = 15;\n    xSpeed = 30;\n}\n\nelse if (error >= 80 && error < 100){\n    distance = 20;\n    xSpeed = 30;\n}\n\nelse if (error >= 100){\n    distance = 25;\n    xSpeed = 30;\n}\n\nelse {\n    distance = 0;\n    xSpeed = 0;\n}"("error"=w2270) -> ("distance"=w2265:dbl, "xSpeed"=w2267:dbl)
            n758 = formula code="if (target > 0){\nif (current  >= target)\noutput = 1;\n\nelse if (current != target)\noutput = 0;\n}\n\nelse if (target == 0){\nif (current == target)\noutput = 1;\n\nelse if (current != target)\noutput = 0;\n}\n\nelse if (target < 0){\nif (current <= target)\noutput = 1;\n\nelse if (current != target)\noutput = 0;\n}\n\nelse if (current != target)\noutput = 0;"("target"=w2265, "current"=w2266) -> ("output"=w2264:dbl)
            n759 = Bundle By Name(cluster=w2269, "xSpeed"=w2267) -> (w2268:T19)
            n760 = Equal?(x=w2264, y=1.0) -> (x = y?=w2261:bool)
            n761 = case shown="\"Start Task 1\", Default" w2274 {
              tunnel: [w2289 State_Type_Definitions,_for_0.26g_versions_and_later_3."True Stop" ("Enum")] -> w2281
              tunnel: [w2292 w2309] -> w2280
              tunnel: [State_Type_Definitions,_for_0.26g_versions_and_later_3."Idle" ("Enum") State_Type_Definitions,_for_0.26g_versions_and_later_3."Shutdown" ("Enum")] -> w2282
              tunnel: w2278 -> [w2288 _]
              tunnel: w2279 -> [w2284 w2306]
              tunnel: w2261 -> [w2283 _]
              frame "Start Task 1", Default {
                # ">> T: Breaks out of state loop; F: Stays in loop>>"
                # ">> Manual override >>"
                # ">> Checks if time is up>>"
                # "Stays in Task 5D until the object is detected"
                # "T: Go back to idle, F: Continue with task\""
                # ">> Manual override >>"
                n762 = case shown="True" w2283 {
                  tunnel: [w2296 w2302] -> w2292
                  tunnel: w2284 -> [w2294 w2300]
                  frame False {
                    n763 = for {
                      tunnel: string[] ["X AXIS - SLOW", "READ ENCODERS", "READ NAVX"] ("element") -> [w2297] mode=indexing
                      shift-right: [w2299] -> w2296
                      shift-left: w2294 -> [w2298]
                      n764 = Enqueue Element(queue=w2298, element=w2297) -> (queue out=w2299:refnum<queue>)  [unwired: 2 in, 2 out]
                    }
                  }
                  frame True {
                    n765 = for {
                      shift-right: [w2304] -> w2302
                      shift-left: w2300 -> [w2305]
                      tunnel: string[] ["SET TIMER 2", "STOP", "READ STEPPER VALUES", ""] -> [w2303] mode=indexing
                      n766 = Enqueue Element(queue=w2305, element=w2303) -> (queue out=w2304:refnum<queue>)  [unwired: 2 in, 2 out]
                    }
                  }
                }
                n767 = Or(x=w2283, y=w2288) -> (x .or. y?=w2290:bool)
                n768 = Select(t=State_Type_Definitions,_for_0.26g_versions_and_later_3."True Stop" ("Enum"), s=w2288, f=State_Type_Definitions,_for_0.26g_versions_and_later_3."Task 8H: ARM ADJUST" ("Enum")) -> (s? t:f=w2285:T18)
                n769 = Select(t=w2285, s=w2290, f=State_Type_Definitions,_for_0.26g_versions_and_later_3."Task 8E: ROBOT ADJUST" ("Enum")) -> (s? t:f=w2289:T18)
              }
              frame "Exit" {
                n770 = for {
                  shift-right: [w2312] -> w2309
                  shift-left: w2306 -> [w2313]
                  tunnel: string[] ["STOP", "RESET ENCODERS", "RESET YAW", "ARDUINO MODE 0"] -> [w2311] mode=indexing
                  n771 = Enqueue Element(queue=w2313, element=w2311) -> (queue out=w2312:refnum<queue>)  [unwired: 2 in, 2 out]
                }
              }
            }
          }
          frame "Task 8F: CAM BURST 2" {
            # ">>> Motor control cluster >>>"
            # ">>> yStepper command>>>"
            # ">> Manual override >>"
            n772 = Dequeue Element(queue=w2324, timeout in ms (-1)=w2323, error in (no error)=w2322) -> (element=w2321:T10)  [unwired: 3 out]
            n773 = case shown="\"Start Task 1\", Default" w2321 {
              tunnel: [w2333 State_Type_Definitions,_for_0.26g_versions_and_later_3."True Stop" ("Enum")] -> w2326
              tunnel: [w2336 w2353] -> w2319
              tunnel: [State_Type_Definitions,_for_0.26g_versions_and_later_3."Idle" ("Enum") State_Type_Definitions,_for_0.26g_versions_and_later_3."Shutdown" ("Enum")] -> w2318
              tunnel: w2320 -> [w2327 _]
              tunnel: w2325 -> [w2332 w2350]
              tunnel: w2316 -> [w2331 _]
              frame "Start Task 1", Default {
                # ">> Is time up? >>"
                # "Determines if object is in range to pick up"
                # ">> Manual override >>"
                n774 = case shown="False" w2331 {
                  tunnel: [w2340 w2346] -> w2336
                  tunnel: w2332 -> [w2338 w2344]
                  frame False {
                    n775 = for {
                      tunnel: string[] ["CAM ACQ", "START TIMER"] ("element") -> [w2341] mode=indexing
                      shift-right: [w2343] -> w2340
                      shift-left: w2338 -> [w2342]
                      n776 = Enqueue Element(queue=w2342, element=w2341) -> (queue out=w2343:refnum<queue>)  [unwired: 2 in, 2 out]
                    }
                  }
                  frame True {
                    n777 = for {
                      shift-right: [w2348] -> w2346
                      shift-left: w2344 -> [w2349]
                      tunnel: string[] ["CAM CLOSE", "PROCESS IMAGE", "SET TIMER 3"] -> [w2347] mode=indexing
                      n778 = Enqueue Element(queue=w2349, element=w2347) -> (queue out=w2348:refnum<queue>)  [unwired: 2 in, 2 out]
                    }
                  }
                }
                n779 = Or(x=w2331, y=w2327) -> (x .or. y?=w2334:bool)
                n780 = Select(t=State_Type_Definitions,_for_0.26g_versions_and_later_3."True Stop" ("Enum"), s=w2327, f=State_Type_Definitions,_for_0.26g_versions_and_later_3."Task 8G: PROCESS IMAGE 2" ("Enum")) -> (s? t:f=w2329:T18)
                n781 = Select(t=w2329, s=w2334, f=State_Type_Definitions,_for_0.26g_versions_and_later_3."Task 8F: CAM BURST 2" ("Enum")) -> (s? t:f=w2333:T18)
              }
              frame "Exit" {
                n782 = for {
                  shift-right: [w2356] -> w2353
                  shift-left: w2350 -> [w2357]
                  tunnel: string[] ["STOP", "RESET ENCODERS", "RESET YAW", "ARDUINO MODE 0"] -> [w2355] mode=indexing
                  n783 = Enqueue Element(queue=w2357, element=w2355) -> (queue out=w2356:refnum<queue>)  [unwired: 2 in, 2 out]
                }
              }
            }
          }
          frame "Task 8G: PROCESS IMAGE 2" {
            # ">>> yStepper command>>>"
            n784 = Dequeue Element(queue=w2365, timeout in ms (-1)=w2364, error in (no error)=w2363) -> (element=w2362:T10)  [unwired: 3 out]
            n785 = case shown="\"Start Task 1\", Default" w2362 {
              tunnel: [w2377 State_Type_Definitions,_for_0.26g_versions_and_later_3."True Stop" ("Enum")] -> w2369
              tunnel: [w2380 w2397] -> w2368
              tunnel: [State_Type_Definitions,_for_0.26g_versions_and_later_3."Idle" ("Enum") State_Type_Definitions,_for_0.26g_versions_and_later_3."Shutdown" ("Enum")] -> w2370
              tunnel: w2366 -> [w2376 _]
              tunnel: w2367 -> [w2372 w2394]
              tunnel: w2360 -> [w2371 _]
              frame "Start Task 1", Default {
                # ">> T: Breaks out of state loop; F: Stays in loop>>"
                # ">> Manual override >>"
                # ">> Checks if time is up>>"
                # "Stays in Task 5D until the object is detected"
                # "T: Go back to idle, F: Continue with task\""
                # ">> Manual override >>"
                n786 = case shown="False" w2371 {
                  tunnel: [w2384 w2390] -> w2380
                  tunnel: w2372 -> [w2382 w2388]
                  frame False {
                    n787 = for {
                      tunnel: string[] ["START TIMER", "PROCESS IMAGE", ""] ("element") -> [w2385] mode=indexing
                      shift-right: [w2387] -> w2384
                      shift-left: w2382 -> [w2386]
                      n788 = Enqueue Element(queue=w2386, element=w2385) -> (queue out=w2387:refnum<queue>)  [unwired: 2 in, 2 out]
                    }
                  }
                  frame True {
                    n789 = for {
                      shift-right: [w2392] -> w2390
                      shift-left: w2388 -> [w2393]
                      tunnel: string[] ["READ STEPPER VALUES", "Y STEPPER CONTROL", ""] -> [w2391] mode=indexing
                      n790 = Enqueue Element(queue=w2393, element=w2391) -> (queue out=w2392:refnum<queue>)  [unwired: 2 in, 2 out]
                    }
                  }
                }
                n791 = Or(x=w2371, y=w2376) -> (x .or. y?=w2378:bool)
                n792 = Select(t=State_Type_Definitions,_for_0.26g_versions_and_later_3."True Stop" ("Enum"), s=w2376, f=State_Type_Definitions,_for_0.26g_versions_and_later_3."Task 8H: ARM ADJUST" ("Enum")) -> (s? t:f=w2373:T18)
                n793 = Select(t=w2373, s=w2378, f=State_Type_Definitions,_for_0.26g_versions_and_later_3."Task 8G: PROCESS IMAGE 2" ("Enum")) -> (s? t:f=w2377:T18)
              }
              frame "Exit" {
                n794 = for {
                  shift-right: [w2400] -> w2397
                  shift-left: w2394 -> [w2401]
                  tunnel: string[] ["STOP", "RESET ENCODERS", "RESET YAW", "ARDUINO MODE 0"] -> [w2399] mode=indexing
                  n795 = Enqueue Element(queue=w2401, element=w2399) -> (queue out=w2400:refnum<queue>)  [unwired: 2 in, 2 out]
                }
              }
            }
          }
          frame "Task 8H: ARM ADJUST" {
            # ">>> yStepper command>>>"
            n796 = Dequeue Element(queue=w2415, timeout in ms (-1)=w2416, error in (no error)=w2417) -> (element=w2419:T10)  [unwired: 3 out]
            n797 = formula code="if (pos >= 50 && pos < 80)\ny = 40;\n\nelse if (pos >= 80 && pos < 100)\ny = 35;\n\nelse if (pos >= 100 && pos < 120)\ny = 20;\n\nelse if (pos >= 120 && pos < 140)\ny = 15;\n\nelse if (pos >= 140 && pos < 150)\ny = 10;\n\nelse if (pos >= 150 && 170)\ny = 5;\n\nelse \ny = 0;"("pos"=w2407) -> ("y"=w2410:dbl)
            n798 = To Unsigned Byte Integer(number=w2410) -> (unsigned 8bit integer=w2405:u8)
            n799 = Equal?(x=w2406, y=w2405) -> (x = y?=w2404:bool)
            n800 = case shown="\"Start Task 1\", Default" w2419 {
              tunnel: [w2426 State_Type_Definitions,_for_0.26g_versions_and_later_3."True Stop" ("Enum")] -> w2413
              tunnel: [w2429 w2446] -> w2411
              tunnel: [State_Type_Definitions,_for_0.26g_versions_and_later_3."Idle" ("Enum") State_Type_Definitions,_for_0.26g_versions_and_later_3."Shutdown" ("Enum")] -> w2412
              tunnel: w2418 -> [w2425 _]
              tunnel: w2414 -> [w2421 w2443]
              tunnel: w2404 -> [w2420 _]
              frame "Start Task 1", Default {
                # ">> T: Breaks out of state loop; F: Stays in loop>>"
                # ">> Manual override >>"
                # ">> Checks if time is up>>"
                # "Stays in Task 5D until the object is detected"
                # "T: Go back to idle, F: Continue with task\""
                # ">> Manual override >>"
                n801 = case shown="False" w2420 {
                  tunnel: [w2433 w2439] -> w2429
                  tunnel: w2421 -> [w2431 w2437]
                  frame False {
                    n802 = for {
                      tunnel: string[] ["READ STEPPER VALUES", "Y STEPPER CONTROL", ""] ("element") -> [w2434] mode=indexing
                      shift-right: [w2436] -> w2433
                      shift-left: w2431 -> [w2435]
                      n803 = Enqueue Element(queue=w2435, element=w2434) -> (queue out=w2436:refnum<queue>)  [unwired: 2 in, 2 out]
                    }
                  }
                  frame True {
                    n804 = for {
                      shift-right: [w2441] -> w2439
                      shift-left: w2437 -> [w2442]
                      tunnel: string[] ["DISPOSE BUFFERS", "READ STEPPER VALUES", ""] -> [w2440] mode=indexing
                      n805 = Enqueue Element(queue=w2442, element=w2440) -> (queue out=w2441:refnum<queue>)  [unwired: 2 in, 2 out]
                    }
                  }
                }
                n806 = Or(x=w2420, y=w2425) -> (x .or. y?=w2427:bool)
                n807 = Select(t=State_Type_Definitions,_for_0.26g_versions_and_later_3."True Stop" ("Enum"), s=w2425, f=State_Type_Definitions,_for_0.26g_versions_and_later_3."Task 8I: ARM GRAB HEIGHT" ("Enum")) -> (s? t:f=w2422:T18)
                n808 = Select(t=w2422, s=w2427, f=State_Type_Definitions,_for_0.26g_versions_and_later_3."Task 8H: ARM ADJUST" ("Enum")) -> (s? t:f=w2426:T18)
              }
              frame "Exit" {
                n809 = for {
                  shift-right: [w2449] -> w2446
                  shift-left: w2443 -> [w2450]
                  tunnel: string[] ["STOP", "RESET ENCODERS", "RESET YAW", "ARDUINO MODE 0"] -> [w2448] mode=indexing
                  n810 = Enqueue Element(queue=w2450, element=w2448) -> (queue out=w2449:refnum<queue>)  [unwired: 2 in, 2 out]
                }
              }
            }
            n811 = Bundle By Name(cluster=w2409, "yStepper desired"=w2405) -> (w2408:T20)
          }
          frame "Task 8I: ARM GRAB HEIGHT" {
            # ">>> Motor control cluster >>>"
            # ">>> yStepper command>>>"
            # ">> Manual override >>"
            n812 = Dequeue Element(queue=w2461, timeout in ms (-1)=w2460, error in (no error)=w2462) -> (element=w2459:T10)  [unwired: 3 out]
            n813 = Equal?(x=w2458, y=u8 1) -> (x = y?=w2456:bool)
            n814 = case shown="\"Start Task 1\", Default" w2459 {
              tunnel: [w2472 State_Type_Definitions,_for_0.26g_versions_and_later_3."True Stop" ("Enum")] -> w2463
              tunnel: [w2475 w2492] -> w2464
              tunnel: [State_Type_Definitions,_for_0.26g_versions_and_later_3."Idle" ("Enum") State_Type_Definitions,_for_0.26g_versions_and_later_3."Shutdown" ("Enum")] -> w2465
              tunnel: w2456 -> [w2471 _]
              tunnel: w2455 -> [w2470 _]
              tunnel: w2454 -> [w2466 w2489]
              frame "Start Task 1", Default {
                # "Stays in Task 5F until stepper reaches desired \nheight"
                # "T: Go back to idle, F: Continue with task\""
                # ">> Manual override >>"
                n815 = case shown="True" w2471 {
                  tunnel: [w2479 w2485] -> w2475
                  tunnel: w2466 -> [w2477 w2483]
                  frame False {
                    n816 = for {
                      tunnel: string[] ["Z STEPPER GRAB HEIGHT", "READ STEPPER VALUES"] ("element") -> [w2480] mode=indexing
                      shift-right: [w2482] -> w2479
                      shift-left: w2477 -> [w2481]
                      n817 = Enqueue Element(queue=w2481, element=w2480) -> (queue out=w2482:refnum<queue>)  [unwired: 2 in, 2 out]
                    }
                  }
                  frame True {
                    n818 = for {
                      shift-right: [w2487] -> w2485
                      shift-left: w2483 -> [w2488]
                      tunnel: string[] ["SET TIMER 2", "CLOSE CLAW", ""] -> [w2486] mode=indexing
                      n819 = Enqueue Element(queue=w2488, element=w2486) -> (queue out=w2487:refnum<queue>)  [unwired: 2 in, 2 out]
                    }
                  }
                }
                n820 = Or(x=w2471, y=w2470) -> (x .or. y?=w2473:bool)
                n821 = Select(t=State_Type_Definitions,_for_0.26g_versions_and_later_3."True Stop" ("Enum"), s=w2470, f=State_Type_Definitions,_for_0.26g_versions_and_later_3."Task 8J: CLOSE CLAW" ("Enum")) -> (s? t:f=w2467:T18)
                n822 = Select(t=w2467, s=w2473, f=State_Type_Definitions,_for_0.26g_versions_and_later_3."Task 8I: ARM GRAB HEIGHT" ("Enum")) -> (s? t:f=w2472:T18)
              }
              frame "Exit" {
                n823 = for {
                  shift-right: [w2495] -> w2492
                  shift-left: w2489 -> [w2496]
                  tunnel: string[] ["STOP", "RESET ENCODERS", "RESET YAW", "ARDUINO MODE 0"] -> [w2494] mode=indexing
                  n824 = Enqueue Element(queue=w2496, element=w2494) -> (queue out=w2495:refnum<queue>)  [unwired: 2 in, 2 out]
                }
              }
            }
          }
          frame "Task 8J: CLOSE CLAW" {
            # ">>> yStepper command>>>"
            # ">> Manual override >>"
            n825 = Dequeue Element(queue=w2507, timeout in ms (-1)=w2506, error in (no error)=w2505) -> (element=w2504:T10)  [unwired: 3 out]
            n826 = case shown="\"Start Task 1\", Default" w2504 {
              tunnel: [w2516 State_Type_Definitions,_for_0.26g_versions_and_later_3."True Stop" ("Enum")] -> w2509
              tunnel: [w2519 w2536] -> w2502
              tunnel: [State_Type_Definitions,_for_0.26g_versions_and_later_3."Idle" ("Enum") State_Type_Definitions,_for_0.26g_versions_and_later_3."Shutdown" ("Enum")] -> w2501
              tunnel: w2503 -> [w2510 _]
              tunnel: w2508 -> [w2515 w2533]
              tunnel: w2499 -> [w2514 _]
              frame "Start Task 1", Default {
                # ">> Is time up? >>"
                # "Determines if object is in range to pick up"
                # ">> Manual override >>"
                n827 = case shown="True" w2514 {
                  tunnel: [w2523 w2529] -> w2519
                  tunnel: w2515 -> [w2521 w2527]
                  frame False {
                    n828 = for {
                      tunnel: string[] ["CLOSE CLAW", "START TIMER"] ("element") -> [w2524] mode=indexing
                      shift-right: [w2526] -> w2523
                      shift-left: w2521 -> [w2525]
                      n829 = Enqueue Element(queue=w2525, element=w2524) -> (queue out=w2526:refnum<queue>)  [unwired: 2 in, 2 out]
                    }
                  }
                  frame True {
                    n830 = for {
                      shift-right: [w2531] -> w2529
                      shift-left: w2527 -> [w2532]
                      tunnel: string[] ["READ STEPPER VALUES", "", ""] -> [w2530] mode=indexing
                      n831 = Enqueue Element(queue=w2532, element=w2530) -> (queue out=w2531:refnum<queue>)  [unwired: 2 in, 2 out]
                    }
                  }
                }
                n832 = Or(x=w2514, y=w2510) -> (x .or. y?=w2517:bool)
                n833 = Select(t=State_Type_Definitions,_for_0.26g_versions_and_later_3."True Stop" ("Enum"), s=w2510, f=State_Type_Definitions,_for_0.26g_versions_and_later_3."Task 8K: RAISE MY SWORD" ("Enum")) -> (s? t:f=w2512:T18)
                n834 = Select(t=w2512, s=w2517, f=State_Type_Definitions,_for_0.26g_versions_and_later_3."Task 8J: CLOSE CLAW" ("Enum")) -> (s? t:f=w2516:T18)
              }
              frame "Exit" {
                n835 = for {
                  shift-right: [w2539] -> w2536
                  shift-left: w2533 -> [w2540]
                  tunnel: string[] ["STOP", "RESET ENCODERS", "RESET YAW", "ARDUINO MODE 0"] -> [w2538] mode=indexing
                  n836 = Enqueue Element(queue=w2540, element=w2538) -> (queue out=w2539:refnum<queue>)  [unwired: 2 in, 2 out]
                }
              }
            }
          }
          frame "Task 8K: RAISE MY SWORD" {
            # ">>> yStepper command>>>"
            # ">> Manual override >>"
            n837 = Dequeue Element(queue=w2551, timeout in ms (-1)=w2550, error in (no error)=w2552) -> (element=w2549:T10)  [unwired: 3 out]
            n838 = Equal?(x=w2548, y=u8 60) -> (x = y?=w2546:bool)
            n839 = case shown="\"Start Task 1\", Default" w2549 {
              tunnel: [w2562 State_Type_Definitions,_for_0.26g_versions_and_later_3."True Stop" ("Enum")] -> w2553
              tunnel: [w2565 w2582] -> w2554
              tunnel: [State_Type_Definitions,_for_0.26g_versions_and_later_3."Idle" ("Enum") State_Type_Definitions,_for_0.26g_versions_and_later_3."Shutdown" ("Enum")] -> w2555
              tunnel: w2546 -> [w2561 _]
              tunnel: w2545 -> [w2560 _]
              tunnel: w2544 -> [w2556 w2579]
              frame "Start Task 1", Default {
                # "Stays in Task 5_A until stepper reaches desired \nheight"
                # "T: Go back to idle, F: Continue with task\""
                # ">> Manual override >>"
                n840 = case shown="True" w2561 {
                  tunnel: [w2569 w2575] -> w2565
                  tunnel: w2556 -> [w2567 w2573]
                  frame False {
                    n841 = for {
                      tunnel: string[] ["Z STEPPER CAM HEIGHT", "READ STEPPER VALUES"] ("element") -> [w2570] mode=indexing
                      shift-right: [w2572] -> w2569
                      shift-left: w2567 -> [w2571]
                      n842 = Enqueue Element(queue=w2571, element=w2570) -> (queue out=w2572:refnum<queue>)  [unwired: 2 in, 2 out]
                    }
                  }
                  frame True {
                    n843 = for {
                      shift-right: [w2577] -> w2575
                      shift-left: w2573 -> [w2578]
                      tunnel: string[] ["CAM CLOSE", "DISPOSE CAM BUFFERS", "DISPOSE PROC BUFFERS", "RESET ENCODERS"] -> [w2576] mode=indexing
                      n844 = Enqueue Element(queue=w2578, element=w2576) -> (queue out=w2577:refnum<queue>)  [unwired: 2 in, 2 out]
                    }
                  }
                }
                n845 = Or(x=w2561, y=w2560) -> (x .or. y?=w2563:bool)
                n846 = Select(t=State_Type_Definitions,_for_0.26g_versions_and_later_3."True Stop" ("Enum"), s=w2560, f=State_Type_Definitions,_for_0.26g_versions_and_later_3."True Stop" ("Enum")) -> (s? t:f=w2557:T18)
                n847 = Select(t=w2557, s=w2563, f=State_Type_Definitions,_for_0.26g_versions_and_later_3."Task 8K: RAISE MY SWORD" ("Enum")) -> (s? t:f=w2562:T18)
              }
              frame "Exit" {
                n848 = for {
                  shift-right: [w2585] -> w2582
                  shift-left: w2579 -> [w2586]
                  tunnel: string[] ["STOP", "RESET ENCODERS", "RESET YAW", "ARDUINO MODE 0"] -> [w2584] mode=indexing
                  n849 = Enqueue Element(queue=w2586, element=w2584) -> (queue out=w2585:refnum<queue>)  [unwired: 2 in, 2 out]
                }
              }
            }
          }
          frame "Task 9A: Raise Arm" {
            # ">>> Motor control cluster >>>"
            # ">> Stepper height reeached >>"
            # ">>> yStepper command>>>"
            # ">> Manual override >>"
            n850 = Dequeue Element(queue=w2599, timeout in ms (-1)=w2594, error in (no error)=w2598) -> (element=w2601:T10)  [unwired: 3 out]
            n851 = Equal?(x=w2596, y=u8 50) -> (x = y?=w2587:bool)
            n852 = case shown="\"Start Task 1\", Default" w2601 {
              tunnel: [w2612 State_Type_Definitions,_for_0.26g_versions_and_later_3."True Stop" ("Enum")] -> w2592
              tunnel: [w2610 w2627] -> w2591
              tunnel: w2595 -> [w2609 _]
              tunnel: w2597 -> [w2603 _]
              tunnel: [State_Type_Definitions,_for_0.26g_versions_and_later_3."Idle" ("Enum") State_Type_Definitions,_for_0.26g_versions_and_later_3."Shutdown" ("Enum")] -> w2593
              tunnel: w2587 -> [w2602 _]
              frame "Start Task 1", Default {
                # ">> WIill proceed to part ii if not manual override >>"
                # ">>If ENABLE or Trigger is set to true>>"
                n853 = Or(x=w2602, y=w2603) -> (x .or. y?=w2604:bool)
                n854 = case shown="False" w2602 {
                  tunnel: [w2615 w2621] -> w2610
                  tunnel: w2609 -> [w2614 w2620]
                  frame False {
                    n855 = for {
                      shift-right: [w2617] -> w2615
                      shift-left: w2614 -> [w2618]
                      tunnel: string[] ["Z STEPPER BOX HEIGHT", "READ STEPPER VALUES"] ("element") -> [w2616] mode=indexing
                      n856 = Enqueue Element(queue=w2618, element=w2616) -> (queue out=w2617:refnum<queue>)  [unwired: 2 in, 2 out]
                    }
                  }
                  frame True {
                    n857 = for {
                      shift-right: [w2623] -> w2621
                      shift-left: w2620 -> [w2624]
                      tunnel: string[] ["READ NAVX", "RESET FLAGS", "RESET YAW", "", "", ""] -> [w2622] mode=indexing
                      n858 = Enqueue Element(queue=w2624, element=w2622) -> (queue out=w2623:refnum<queue>)  [unwired: 2 in, 2 out]
                    }
                  }
                }
                n859 = Select(t=State_Type_Definitions,_for_0.26g_versions_and_later_3."True Stop" ("Enum"), s=w2603, f=State_Type_Definitions,_for_0.26g_versions_and_later_3."Task 9B: Rotate to Angle" ("Enum")) -> (s? t:f=w2606:T18)
                n860 = Select(t=w2606, s=w2604, f=State_Type_Definitions,_for_0.26g_versions_and_later_3."Task 9A: Raise Arm" ("Enum")) -> (s? t:f=w2612:T18)
              }
              frame "Exit" {
                n861 = for {
                  shift-right: [w2630] -> w2627
                  shift-left: _ -> [w2631]
                  tunnel: string[] ["STOP", "RESET ENCODERS", "RESET YAW", ""] -> [w2629] mode=indexing
                  n862 = Enqueue Element(queue=w2631, element=w2629) -> (queue out=w2630:refnum<queue>)  [unwired: 2 in, 2 out]
                }
              }
            }
          }
          frame "Task 9B: Rotate to Angle" {
            # ">>> Motor control cluster >>>"
            # ">>> yStepper command>>>"
            n863 = Dequeue Element(queue=w2645, timeout in ms (-1)=w2644, error in (no error)=w2643) -> (element=w2647:T10)  [unwired: 3 out]
            n864 = In Range and Coerce(upper limit=65.0, x=w2637, lower limit=58.0) -> (In Range?=w2632:bool)  [unwired: 1 out]
            n865 = case shown="\"Start Task 1\", Default" w2647 {
              tunnel: w2638 -> [w2650 _]
              tunnel: [w2658 State_Type_Definitions,_for_0.26g_versions_and_later_3."True Stop" ("Enum")] -> w2640
              tunnel: w2646 -> [w2656 w2674]
              tunnel: [w2655 w2673] -> w2639
              tunnel: [State_Type_Definitions,_for_0.26g_versions_and_later_3."Idle" ("Enum") State_Type_Definitions,_for_0.26g_versions_and_later_3."Shutdown" ("Enum")] -> w2641
              tunnel: w2632 -> [w2648 _]
              frame "Start Task 1", Default {
                n866 = Or(x=w2648, y=w2650) -> (x .or. y?=w2649:bool)
                n867 = case shown="False" w2648 {
                  tunnel: w2656 -> [w2661 w2667]
                  tunnel: [w2660 w2665] -> w2655
                  frame False {
                    n868 = for {
                      shift-right: [w2663] -> w2660
                      shift-left: w2661 -> [w2664]
                      tunnel: string[] ["READ NAVX", "R-CW", ""] ("element") -> [w2662] mode=indexing
                      n869 = Enqueue Element(queue=w2664, element=w2662) -> (queue out=w2663:refnum<queue>)  [unwired: 2 in, 2 out]
                    }
                  }
                  frame True {
                    n870 = for {
                      shift-right: [w2669] -> w2665
                      shift-left: w2667 -> [w2670]
                      tunnel: string[] ["STOP", "RESET ENCODERS", "RESET YAW", "", ""] -> [w2668] mode=indexing
                      n871 = Enqueue Element(queue=w2670, element=w2668) -> (queue out=w2669:refnum<queue>)  [unwired: 2 in, 2 out]
                    }
                  }
                }
                n872 = Select(t=State_Type_Definitions,_for_0.26g_versions_and_later_3."True Stop" ("Enum"), s=w2650, f=State_Type_Definitions,_for_0.26g_versions_and_later_3."Task 9C: Detect Box") -> (s? t:f=w2652:T18)
                n873 = Select(t=w2652, s=w2649, f=State_Type_Definitions,_for_0.26g_versions_and_later_3."Task 9B: Rotate to Angle" ("Enum")) -> (s? t:f=w2658:T18)
              }
              frame "Exit" {
                n874 = for {
                  shift-right: [w2677] -> w2673
                  shift-left: w2674 -> [w2678]
                  tunnel: string[] ["STOP", "RESET ENCODERS", "RESET YAW", ""] -> [w2676] mode=indexing
                  n875 = Enqueue Element(queue=w2678, element=w2676) -> (queue out=w2677:refnum<queue>)  [unwired: 2 in, 2 out]
                }
              }
            }
          }
          frame "Task 9C: Detect Box" {
            # ">>> Motor control cluster >>>"
            # ">>Line Detected>>"
            # ">>Action Queue>>"
            # ">>> yStepper command>>>"
            n876 = Dequeue Element(queue=w2690, timeout in ms (-1)=w2689, error in (no error)=w2688) -> (element=w2691:T10)  [unwired: 3 out]
            n877 = case shown="\"Start Task 1\", Default" w2691 {
              tunnel: w2686 -> [w2692 _]
              tunnel: [w2702 State_Type_Definitions,_for_0.26g_versions_and_later_3."True Stop" ("Enum")] -> w2683
              tunnel: w2687 -> [w2700 w2718]
              tunnel: [w2699 w2717] -> w2682
              tunnel: [State_Type_Definitions,_for_0.26g_versions_and_later_3."Idle" ("Enum") State_Type_Definitions,_for_0.26g_versions_and_later_3."Shutdown" ("Enum")] -> w2685
              tunnel: w2679 -> [w2693 _]
              frame "Start Task 1", Default {
                n878 = Or(x=w2692, y=w2693) -> (x .or. y?=w2694:bool)
                n879 = case shown="False" w2693 {
                  tunnel: w2700 -> [w2705 w2711]
                  tunnel: [w2704 w2709] -> w2699
                  frame False {
                    n880 = for {
                      shift-right: [w2707] -> w2704
                      shift-left: w2705 -> [w2708]
                      tunnel: string[] ["READ IR", "READ LINE SENSOR", "FORWARD - IR ASSIST"] ("element") -> [w2706] mode=indexing
                      n881 = Enqueue Element(queue=w2708, element=w2706) -> (queue out=w2707:refnum<queue>)  [unwired: 2 in, 2 out]
                    }
                  }
                  frame True {
                    n882 = for {
                      shift-right: [w2713] -> w2709
                      shift-left: w2711 -> [w2714]
                      tunnel: string[] ["STOP", "RESET ENCODERS", "RESET YAW", "RESET FLAGS"] -> [w2712] mode=indexing
                      n883 = Enqueue Element(queue=w2714, element=w2712) -> (queue out=w2713:refnum<queue>)  [unwired: 2 in, 2 out]
                    }
                  }
                }
                n884 = Select(t=State_Type_Definitions,_for_0.26g_versions_and_later_3."True Stop" ("Enum"), s=w2692, f=State_Type_Definitions,_for_0.26g_versions_and_later_3."Task 9D: MOVE FORWARD") -> (s? t:f=w2696:T18)
                n885 = Select(t=w2696, s=w2694, f=State_Type_Definitions,_for_0.26g_versions_and_later_3."Task 9C: Detect Box" ("Enum")) -> (s? t:f=w2702:T18)
              }
              frame "Exit" {
                n886 = for {
                  shift-right: [w2721] -> w2717
                  shift-left: w2718 -> [w2722]
                  tunnel: string[] ["STOP", "RESET ENCODERS", "RESET YAW", ""] -> [w2720] mode=indexing
                  n887 = Enqueue Element(queue=w2722, element=w2720) -> (queue out=w2721:refnum<queue>)  [unwired: 2 in, 2 out]
                }
              }
            }
          }
          frame "Task 9D: MOVE FORWARD" {
            (unwired) 50.0 ("y")
            # ">> Item Selection Bias >>"
            # ">> Wall detected >>"
            # ">> Manual override >>"
            # ">>Table Detected>>"
            # ">>> Motor control cluster >>>"
            # ">>Table or wall detectected>>"
            # ">>Action Queue>>"
            # ">>> yStepper command>>>"
            n888 = Dequeue Element(queue=w2740, timeout in ms (-1)=w2739, error in (no error)=w2738) -> (element=w2741:T10)  [unwired: 3 out]
            n889 = Less Or Equal?(x=w2729, y=20.0) -> (x <= y?=w2724:bool)
            n890 = Less?(x=w2727, y=20.0) -> (x < y?=w2725:bool)
            n891 = Or(x=w2724, y=w2725) -> (x .or. y?=w2723:bool)
            n892 = case shown="\"Start Task 1\", Default" w2741 {
              tunnel: w2736 -> [w2742 _]
              tunnel: [w2752 State_Type_Definitions,_for_0.26g_versions_and_later_3."True Stop" ("Enum")] -> w2733
              tunnel: w2737 -> [w2750 w2768]
              tunnel: [w2749 w2767] -> w2732
              tunnel: [State_Type_Definitions,_for_0.26g_versions_and_later_3."Idle" ("Enum") State_Type_Definitions,_for_0.26g_versions_and_later_3."Shutdown" ("Enum")] -> w2735
              tunnel: w2723 -> [w2743 _]
              frame "Start Task 1", Default {
                n893 = Or(x=w2742, y=w2743) -> (x .or. y?=w2744:bool)
                n894 = case shown="True" w2743 {
                  tunnel: w2750 -> [w2755 w2761]
                  tunnel: [w2754 w2759] -> w2749
                  frame False {
                    n895 = for {
                      shift-right: [w2757] -> w2754
                      shift-left: w2755 -> [w2758]
                      tunnel: string[] ["READ IR", "FORWARD - IR ASSIST", ""] ("element") -> [w2756] mode=indexing
                      n896 = Enqueue Element(queue=w2758, element=w2756) -> (queue out=w2757:refnum<queue>)  [unwired: 2 in, 2 out]
                    }
                  }
                  frame True {
                    n897 = for {
                      shift-right: [w2763] -> w2759
                      shift-left: w2761 -> [w2764]
                      tunnel: string[] ["STOP", "RESET ENCODERS", "RESET YAW", "RESET FLAGS"] -> [w2762] mode=indexing
                      n898 = Enqueue Element(queue=w2764, element=w2762) -> (queue out=w2763:refnum<queue>)  [unwired: 2 in, 2 out]
                    }
                  }
                }
                n899 = Select(t=State_Type_Definitions,_for_0.26g_versions_and_later_3."True Stop" ("Enum"), s=w2742, f=State_Type_Definitions,_for_0.26g_versions_and_later_3."Task 9E: MOVE LEFT") -> (s? t:f=w2746:T18)
                n900 = Select(t=w2746, s=w2744, f=State_Type_Definitions,_for_0.26g_versions_and_later_3."Task 9D: MOVE FORWARD" ("Enum")) -> (s? t:f=w2752:T18)
              }
              frame "Exit" {
                n901 = for {
                  shift-right: [w2771] -> w2767
                  shift-left: w2768 -> [w2772]
                  tunnel: string[] ["STOP", "RESET ENCODERS", "RESET YAW", ""] -> [w2770] mode=indexing
                  n902 = Enqueue Element(queue=w2772, element=w2770) -> (queue out=w2771:refnum<queue>)  [unwired: 2 in, 2 out]
                }
              }
            }
          }
          frame "Task 9E: MOVE LEFT" {
            # ">> Item Selection Bias >>"
            # ">> Line detected? >>"
            # ">> Manual override >>"
            # ">>> Motor control cluster >>>"
            # ">>Action Queue>>"
            # ">>> yStepper command>>>"
            n903 = Dequeue Element(queue=w2784, timeout in ms (-1)=w2783, error in (no error)=w2782) -> (element=w2785:T10)  [unwired: 3 out]
            n904 = case shown="\"Start Task 1\", Default" w2785 {
              tunnel: w2780 -> [w2786 _]
              tunnel: [w2796 State_Type_Definitions,_for_0.26g_versions_and_later_3."True Stop" ("Enum")] -> w2777
              tunnel: w2781 -> [w2794 w2812]
              tunnel: [w2793 w2811] -> w2776
              tunnel: [State_Type_Definitions,_for_0.26g_versions_and_later_3."Idle" ("Enum") State_Type_Definitions,_for_0.26g_versions_and_later_3."Shutdown" ("Enum")] -> w2779
              tunnel: w2773 -> [w2787 _]
              frame "Start Task 1", Default {
                n905 = Or(x=w2786, y=w2787) -> (x .or. y?=w2788:bool)
                n906 = case shown="True" w2787 {
                  tunnel: w2794 -> [w2799 w2805]
                  tunnel: [w2798 w2803] -> w2793
                  frame False {
                    n907 = for {
                      shift-right: [w2801] -> w2798
                      shift-left: w2799 -> [w2802]
                      tunnel: string[] ["LEFT", "READ NAVX", "READ LINE SENSOR", ""] ("element") -> [w2800] mode=indexing
                      n908 = Enqueue Element(queue=w2802, element=w2800) -> (queue out=w2801:refnum<queue>)  [unwired: 2 in, 2 out]
                    }
                  }
                  frame True {
                    n909 = for {
                      shift-right: [w2807] -> w2803
                      shift-left: w2805 -> [w2808]
                      tunnel: string[] ["STOP", "RESET ENCODERS", "RESET YAW", "BOX COLOUR", "", ""] -> [w2806] mode=indexing
                      n910 = Enqueue Element(queue=w2808, element=w2806) -> (queue out=w2807:refnum<queue>)  [unwired: 2 in, 2 out]
                    }
                  }
                }
                n911 = Select(t=State_Type_Definitions,_for_0.26g_versions_and_later_3."True Stop" ("Enum"), s=w2786, f=State_Type_Definitions,_for_0.26g_versions_and_later_3."Task 9F: SCAN BOX") -> (s? t:f=w2790:T18)
                n912 = Select(t=w2790, s=w2788, f=State_Type_Definitions,_for_0.26g_versions_and_later_3."Task 9E: MOVE LEFT" ("Enum")) -> (s? t:f=w2796:T18)
              }
              frame "Exit" {
                n913 = for {
                  shift-right: [w2815] -> w2811
                  shift-left: w2812 -> [w2816]
                  tunnel: string[] ["STOP", "RESET ENCODERS", "RESET YAW", ""] -> [w2814] mode=indexing
                  n914 = Enqueue Element(queue=w2816, element=w2814) -> (queue out=w2815:refnum<queue>)  [unwired: 2 in, 2 out]
                }
              }
            }
          }
          frame "Task 9F: SCAN BOX" {
            # ">>> Motor control cluster >>>"
            # ">>Colour detection >>"
            # ">>> yStepper command>>>"
            # ">> Manual override >>"
            n915 = Dequeue Element(queue=w2833, timeout in ms (-1)=w2831, error in (no error)=w2832) -> (element=w2826:T10)  [unwired: 3 out]
            n916 = call "Box Colour FGV.vi"("Init/R/W State"=Box_Colour_FGV_States."Read") -> ("Colour to detect (output)"=w2819:T2)  [unwired: 9 in, 1 out]
            n917 = Equal?(x=w2820, y=w2819) -> (x = y?=w2818:bool)
            n918 = case shown="\"Start Task 1\", Default" w2826 {
              tunnel: [w2846 State_Type_Definitions,_for_0.26g_versions_and_later_3."True Stop" ("Enum")] -> w2823
              tunnel: [w2844 w2861] -> w2824
              tunnel: w2825 -> [w2843 _]
              tunnel: w2827 -> [w2836 _]
              tunnel: [State_Type_Definitions,_for_0.26g_versions_and_later_3."Idle" ("Enum") State_Type_Definitions,_for_0.26g_versions_and_later_3."Shutdown" ("Enum")] -> w2822
              tunnel: w2817 -> [w2837 _]
              tunnel: w2818 -> [w2835 _]
              frame "Start Task 1", Default {
                # ">> Will stop either due to manual override or is same box colour >>"
                # ">> WIill proceed to part ii if not manual override >>"
                # ">>If ENABLE or Trigger is set to true>>"
                n919 = Or(x=w2837, y=w2836) -> (x .or. y?=w2838:bool)
                n920 = case shown="True" w2837 {
                  tunnel: [w2849 w2855] -> w2844
                  tunnel: w2843 -> [w2848 w2854]
                  frame False {
                    n921 = for {
                      shift-right: [w2851] -> w2849
                      shift-left: w2848 -> [w2852]
                      tunnel: string[] ["", ""] ("element") -> [w2850] mode=indexing
                      n922 = Enqueue Element(queue=w2852, element=w2850) -> (queue out=w2851:refnum<queue>)  [unwired: 2 in, 2 out]
                    }
                  }
                  frame True {
                    n923 = for {
                      shift-right: [w2857] -> w2855
                      shift-left: w2854 -> [w2858]
                      tunnel: string[] ["RESET ENCODER", "RESET FLAGS", "RESET YAW", "", "", ""] -> [w2856] mode=indexing
                      n924 = Enqueue Element(queue=w2858, element=w2856) -> (queue out=w2857:refnum<queue>)  [unwired: 2 in, 2 out]
                    }
                  }
                }
                n925 = Or(x=w2836, y=w2835) -> (x .or. y?=w2834:bool)
                n926 = Select(t=State_Type_Definitions,_for_0.26g_versions_and_later_3."True Stop" ("Enum"), s=w2834, f=State_Type_Definitions,_for_0.26g_versions_and_later_3."Task 9G: MOVE RIGHT" ("Enum")) -> (s? t:f=w2840:T18)
                n927 = Select(t=w2840, s=w2838, f=State_Type_Definitions,_for_0.26g_versions_and_later_3."Task 9F: SCAN BOX" ("Enum")) -> (s? t:f=w2846:T18)
              }
              frame "Exit" {
                n928 = for {
                  shift-right: [w2864] -> w2861
                  shift-left: _ -> [w2865]
                  tunnel: string[] ["STOP", "RESET ENCODERS", "RESET YAW", ""] -> [w2863] mode=indexing
                  n929 = Enqueue Element(queue=w2865, element=w2863) -> (queue out=w2864:refnum<queue>)  [unwired: 2 in, 2 out]
                }
              }
            }
          }
          frame "Task 9G: MOVE RIGHT" {
            # ">>> Motor control cluster >>>"
            # ">>> yStepper command>>>"
            n930 = Dequeue Element(queue=w2877, timeout in ms (-1)=w2876, error in (no error)=w2875) -> (element=w2882:T10)  [unwired: 3 out]
            n931 = Greater?(x=w2867, y=50.0) -> (0:w2870:bool)
            n932 = And(x=w2868, y=w2870) -> (x .and. y?=w2866:bool)
            n933 = case shown="\"Start Task 1\", Default" w2882 {
              tunnel: w2866 -> [w2885 _]
              tunnel: [w2892 State_Type_Definitions,_for_0.26g_versions_and_later_3."True Stop" ("Enum")] -> w2881
              tunnel: w2874 -> [w2884 _]
              tunnel: w2878 -> [w2891 w2908]
              tunnel: [w2890 w2909] -> w2880
              tunnel: [State_Type_Definitions,_for_0.26g_versions_and_later_3."Idle" ("Enum") State_Type_Definitions,_for_0.26g_versions_and_later_3."Shutdown" ("Enum")] -> w2879
              frame "Start Task 1", Default {
                n934 = case shown="True" w2885 {
                  tunnel: w2891 -> [w2895 w2902]
                  tunnel: [w2896 w2901] -> w2890
                  frame False {
                    n935 = for {
                      tunnel: string[] ["READ LINE SENSOR", "READ NAVX", "RIGHT", "READ ENCODERS"] ("element") -> [w2897] mode=indexing
                      shift-right: [w2899] -> w2896
                      shift-left: w2895 -> [w2898]
                      n936 = Enqueue Element(queue=w2898, element=w2897) -> (queue out=w2899:refnum<queue>)  [unwired: 2 in, 2 out]
                    }
                  }
                  frame True {
                    n937 = for {
                      shift-right: [w2904] -> w2901
                      shift-left: w2902 -> [w2905]
                      tunnel: string[] ["RESET ENCODERS", "RESET YAW", "RESET FLAGS", "STOP", "BOX COLOUR"] -> [w2903] mode=indexing
                      n938 = Enqueue Element(queue=w2905, element=w2903) -> (queue out=w2904:refnum<queue>)  [unwired: 2 in, 2 out]
                    }
                  }
                }
                n939 = Or(x=w2885, y=w2884) -> (x .or. y?=w2883:bool)
                n940 = Select(t=State_Type_Definitions,_for_0.26g_versions_and_later_3."True Stop" ("Enum"), s=w2884, f=State_Type_Definitions,_for_0.26g_versions_and_later_3."Task 9H: SCAN BOX 2" ("Enum")) -> (s? t:f=w2886:T18)
                n941 = Select(t=w2886, s=w2883, f=State_Type_Definitions,_for_0.26g_versions_and_later_3."Task 9G: MOVE RIGHT" ("Enum")) -> (s? t:f=w2892:T18)
              }
              frame "Exit" {
                n942 = for {
                  shift-right: [w2912] -> w2909
                  shift-left: w2908 -> [w2913]
                  tunnel: string[] ["STOP", "RESET ENCODERS", "RESET YAW", "ARDUINO MODE 0"] -> [w2911] mode=indexing
                  n943 = Enqueue Element(queue=w2913, element=w2911) -> (queue out=w2912:refnum<queue>)  [unwired: 2 in, 2 out]
                }
              }
            }
          }
          frame "Task 9H: SCAN BOX 2" {
            # ">> Item Selection Bias >>"
            # ">>> Motor control cluster >>>"
            # ">>> yStepper command>>>"
            n944 = Dequeue Element(queue=w2923, timeout in ms (-1)=w2924, error in (no error)=w2925) -> (element=w2927:T10)  [unwired: 3 out]
            n945 = call "Box Colour FGV.vi"("Init/R/W State"=Box_Colour_FGV_States."Read") -> ("Colour to detect (output)"=w2917:T2)  [unwired: 9 in, 1 out]
            n946 = Equal?(x=w2916, y=w2917) -> (x = y?=w2915:bool)
            n947 = case shown="\"Start Task 1\", Default" w2927 {
              tunnel: w2914 -> [w2935 _]
              tunnel: [w2942 State_Type_Definitions,_for_0.26g_versions_and_later_3."True Stop" ("Enum")] -> w2920
              tunnel: w2926 -> [w2932 _]
              tunnel: w2922 -> [w2941 w2958]
              tunnel: [w2940 w2959] -> w2921
              tunnel: [State_Type_Definitions,_for_0.26g_versions_and_later_3."Idle" ("Enum") State_Type_Definitions,_for_0.26g_versions_and_later_3."Shutdown" ("Enum")] -> w2919
              tunnel: w2915 -> [w2933 _]
              frame "Start Task 1", Default {
                n948 = Or(x=w2935, y=w2932) -> (x .or. y?=w2934:bool)
                n949 = Or(x=w2933, y=w2932) -> (x .or. y?=w2931:bool)
                n950 = case shown="True" w2935 {
                  tunnel: w2941 -> [w2945 w2952]
                  tunnel: [w2946 w2951] -> w2940
                  frame False {
                    n951 = for {
                      tunnel: string[] ["", "", "", ""] ("element") -> [w2947] mode=indexing
                      shift-right: [w2949] -> w2946
                      shift-left: w2945 -> [w2948]
                      n952 = Enqueue Element(queue=w2948, element=w2947) -> (queue out=w2949:refnum<queue>)  [unwired: 2 in, 2 out]
                    }
                  }
                  frame True {
                    n953 = for {
                      shift-right: [w2954] -> w2951
                      shift-left: w2952 -> [w2955]
                      tunnel: string[] ["READ NAVX", "RESET FLAGS", "RESET ENCODERS", "", "", ""] -> [w2953] mode=indexing
                      n954 = Enqueue Element(queue=w2955, element=w2953) -> (queue out=w2954:refnum<queue>)  [unwired: 2 in, 2 out]
                    }
                  }
                }
                n955 = Select(t=State_Type_Definitions,_for_0.26g_versions_and_later_3."True Stop" ("Enum"), s=w2931, f=State_Type_Definitions,_for_0.26g_versions_and_later_3."Task 9I: ROTATE 90 CW" ("Enum")) -> (s? t:f=w2936:T18)
                n956 = Select(t=w2936, s=w2934, f=State_Type_Definitions,_for_0.26g_versions_and_later_3."Task 9H: SCAN BOX 2" ("Enum")) -> (s? t:f=w2942:T18)
              }
              frame "Exit" {
                n957 = for {
                  shift-right: [w2962] -> w2959
                  shift-left: w2958 -> [w2963]
                  tunnel: string[] ["STOP", "RESET ENCODERS", "RESET YAW", "ARDUINO MODE 0"] -> [w2961] mode=indexing
                  n958 = Enqueue Element(queue=w2963, element=w2961) -> (queue out=w2962:refnum<queue>)  [unwired: 2 in, 2 out]
                }
              }
            }
          }
          frame "Task 9I: ROTATE 90 CW" {
            # "High battery voltage: -36\nMid voltage: -38 \nLow voltage: -40"
            # ">> Item Selection Bias >>"
            n959 = Less Or Equal?(x=w2966, y=-38.0) -> (x <= y?=w2964:bool)
            n960 = Dequeue Element(queue=w2967, timeout in ms (-1)=w2968, error in (no error)=w2969) -> (element=w2975:T10)  [unwired: 3 out]
            n961 = case shown="\"Start Task 1\", Default" w2975 {
              tunnel: w2964 -> [w2981 _]
              tunnel: [w2988 State_Type_Definitions,_for_0.26g_versions_and_later_3."True Stop" ("Enum")] -> w2972
              tunnel: w2970 -> [w2980 _]
              tunnel: w2974 -> [w2987 w3004]
              tunnel: [w2986 w3005] -> w2973
              tunnel: [State_Type_Definitions,_for_0.26g_versions_and_later_3."Idle" ("Enum") State_Type_Definitions,_for_0.26g_versions_and_later_3."Shutdown" ("Enum")] -> w2971
              frame "Start Task 1", Default {
                n962 = case shown="False" w2981 {
                  tunnel: w2987 -> [w2991 w2998]
                  tunnel: [w2992 w2997] -> w2986
                  frame False {
                    n963 = for {
                      tunnel: string[] ["R-CW", "READ ENCODERS", "READ IR", "READ NAVX"] ("element") -> [w2993] mode=indexing
                      shift-right: [w2995] -> w2992
                      shift-left: w2991 -> [w2994]
                      n964 = Enqueue Element(queue=w2994, element=w2993) -> (queue out=w2995:refnum<queue>)  [unwired: 2 in, 2 out]
                    }
                  }
                  frame True {
                    n965 = for {
                      shift-right: [w3000] -> w2997
                      shift-left: w2998 -> [w3001]
                      tunnel: string[] ["STOP", "RESET ENCODERS", "RESET YAW", "RESET FLAGS", "READ IR", ""] -> [w2999] mode=indexing
                      n966 = Enqueue Element(queue=w3001, element=w2999) -> (queue out=w3000:refnum<queue>)  [unwired: 2 in, 2 out]
                    }
                  }
                }
                n967 = Or(x=w2981, y=w2980) -> (x .or. y?=w2979:bool)
                n968 = Select(t=State_Type_Definitions,_for_0.26g_versions_and_later_3."True Stop" ("Enum"), s=w2980, f=State_Type_Definitions,_for_0.26g_versions_and_later_3."Task 9J: FORWARD" ("Enum")) -> (s? t:f=w2982:T18)
                n969 = Select(t=w2982, s=w2979, f=State_Type_Definitions,_for_0.26g_versions_and_later_3."Task 9I: ROTATE 90 CW" ("Enum")) -> (s? t:f=w2988:T18)
              }
              frame "Exit" {
                n970 = for {
                  shift-right: [w3008] -> w3005
                  shift-left: w3004 -> [w3009]
                  tunnel: string[] ["STOP", "RESET ENCODERS", "RESET YAW", "ARDUINO MODE 0"] -> [w3007] mode=indexing
                  n971 = Enqueue Element(queue=w3009, element=w3007) -> (queue out=w3008:refnum<queue>)  [unwired: 2 in, 2 out]
                }
              }
            }
          }
          frame "Task 9J: FORWARD" {
            # "Tried values: 70, 150"
            # ">>Stops if either table or wall is obstructing >>"
            # ">> Item Selection Bias >>"
            n972 = Less?(x=w3012, y=150.0) -> (x < y?=w3015:bool)
            n973 = Greater Than 0?(x=w3012) -> (x > 0?=w3014:bool)
            n974 = Less Or Equal?(x=w3018, y=20.0) -> (x <= y?=w3016:bool)
            n975 = Greater Than 0?(x=w3018) -> (x > 0?=w3017:bool)
            n976 = And(x=w3014, y=w3015) -> ()  [unwired: 1 out]
            n977 = Dequeue Element(queue=w3024, timeout in ms (-1)=w3025, error in (no error)=w3026) -> (element=w3028:T10)  [unwired: 3 out]
            n978 = And(x=w3017, y=w3016) -> (x .and. y?=w3010:bool)
            n979 = Or(x=w3010, y=w3010) -> (x .or. y?=w3011:bool)
            n980 = case shown="\"Start Task 1\", Default" w3028 {
              tunnel: w3011 -> [w3034 _]
              tunnel: [w3041 State_Type_Definitions,_for_0.26g_versions_and_later_3."True Stop" ("Enum")] -> w3022
              tunnel: w3027 -> [w3033 _]
              tunnel: w3023 -> [w3040 w3057]
              tunnel: [w3039 w3058] -> w3021
              tunnel: [State_Type_Definitions,_for_0.26g_versions_and_later_3."Idle" ("Enum") State_Type_Definitions,_for_0.26g_versions_and_later_3."Shutdown" ("Enum")] -> w3020
              frame "Start Task 1", Default {
                n981 = case shown="True" w3034 {
                  tunnel: w3040 -> [w3044 w3051]
                  tunnel: [w3045 w3050] -> w3039
                  frame False {
                    n982 = for {
                      tunnel: string[] ["READ IR", "READ NAVX", "FORWARD"] ("element") -> [w3046] mode=indexing
                      shift-right: [w3048] -> w3045
                      shift-left: w3044 -> [w3047]
                      n983 = Enqueue Element(queue=w3047, element=w3046) -> (queue out=w3048:refnum<queue>)  [unwired: 2 in, 2 out]
                    }
                  }
                  frame True {
                    n984 = for {
                      shift-right: [w3053] -> w3050
                      shift-left: w3051 -> [w3054]
                      tunnel: string[] ["STOP", "RESET ENCODERS", "RESET YAW", "RESET FLAGS", "READ IR", ""] -> [w3052] mode=indexing
                      n985 = Enqueue Element(queue=w3054, element=w3052) -> (queue out=w3053:refnum<queue>)  [unwired: 2 in, 2 out]
                    }
                  }
                }
                n986 = Or(x=w3034, y=w3033) -> (x .or. y?=w3032:bool)
                n987 = Select(t=State_Type_Definitions,_for_0.26g_versions_and_later_3."True Stop" ("Enum"), s=w3033, f=State_Type_Definitions,_for_0.26g_versions_and_later_3."Task 9K: RAM WALL" ("Enum")) -> (s? t:f=w3035:T18)
                n988 = Select(t=w3035, s=w3032, f=State_Type_Definitions,_for_0.26g_versions_and_later_3."Task 9J: FORWARD" ("Enum")) -> (s? t:f=w3041:T18)
              }
              frame "Exit" {
                n989 = for {
                  shift-right: [w3061] -> w3058
                  shift-left: w3057 -> [w3062]
                  tunnel: string[] ["STOP", "RESET ENCODERS", "RESET YAW", "ARDUINO MODE 0"] -> [w3060] mode=indexing
                  n990 = Enqueue Element(queue=w3062, element=w3060) -> (queue out=w3061:refnum<queue>)  [unwired: 2 in, 2 out]
                }
              }
            }
          }
          frame "Task 9K: RAM WALL" {
            # "High battery voltage: 15"
            # ">> Item Selection Bias >>"
            # ">>Stops if either table or wall is obstructing >>"
            n991 = Less?(x=w3063, y=15.0) -> (x < y?=w3073:bool)
            n992 = Dequeue Element(queue=w3071, timeout in ms (-1)=w3070, error in (no error)=w3069) -> (element=w3075:T10)  [unwired: 3 out]
            n993 = case shown="\"Start Task 1\", Default" w3075 {
              tunnel: w3073 -> [w3080 _]
              tunnel: [w3087 State_Type_Definitions,_for_0.26g_versions_and_later_3."True Stop" ("Enum")] -> w3065
              tunnel: w3068 -> [w3079 _]
              tunnel: w3072 -> [w3086 w3103]
              tunnel: [w3085 w3104] -> w3066
              tunnel: [State_Type_Definitions,_for_0.26g_versions_and_later_3."Idle" ("Enum") State_Type_Definitions,_for_0.26g_versions_and_later_3."Shutdown" ("Enum")] -> w3064
              frame "Start Task 1", Default {
                n994 = case shown="True" w3080 {
                  tunnel: w3086 -> [w3090 w3097]
                  tunnel: [w3091 w3096] -> w3085
                  frame False {
                    n995 = for {
                      tunnel: string[] ["LEFT", "READ NAVX", "READ IR", ""] ("element") -> [w3092] mode=indexing
                      shift-right: [w3094] -> w3091
                      shift-left: w3090 -> [w3093]
                      n996 = Enqueue Element(queue=w3093, element=w3092) -> (queue out=w3094:refnum<queue>)  [unwired: 2 in, 2 out]
                    }
                  }
                  frame True {
                    n997 = for {
                      shift-right: [w3099] -> w3096
                      shift-left: w3097 -> [w3100]
                      tunnel: string[] ["STOP", "RESET ENCODERS", "RESET FLAGS", "RESET YAW", "READ IR", ""] -> [w3098] mode=indexing
                      n998 = Enqueue Element(queue=w3100, element=w3098) -> (queue out=w3099:refnum<queue>)  [unwired: 2 in, 2 out]
                    }
                  }
                }
                n999 = Or(x=w3080, y=w3079) -> (x .or. y?=w3078:bool)
                n1000 = Select(t=State_Type_Definitions,_for_0.26g_versions_and_later_3."True Stop" ("Enum"), s=w3079, f=State_Type_Definitions,_for_0.26g_versions_and_later_3."Task 9L: MOVE RIGHT" ("Enum")) -> (s? t:f=w3081:T18)
                n1001 = Select(t=w3081, s=w3078, f=State_Type_Definitions,_for_0.26g_versions_and_later_3."Task 9K: RAM WALL" ("Enum")) -> (s? t:f=w3087:T18)
              }
              frame "Exit" {
                n1002 = for {
                  shift-right: [w3107] -> w3104
                  shift-left: w3103 -> [w3108]
                  tunnel: string[] ["STOP", "RESET ENCODERS", "RESET YAW", "ARDUINO MODE 0"] -> [w3106] mode=indexing
                  n1003 = Enqueue Element(queue=w3108, element=w3106) -> (queue out=w3107:refnum<queue>)  [unwired: 2 in, 2 out]
                }
              }
            }
          }
          frame "Task 9L: MOVE RIGHT" {
            # "High battery voltage: 15"
            # ">>> Motor control cluster >>>"
            # ">>> yStepper command>>>"
            # ">> Item Selection Bias >>"
            n1004 = Dequeue Element(queue=w3116, timeout in ms (-1)=w3115, error in (no error)=w3114) -> (element=w3118:T10)  [unwired: 3 out]
            n1005 = case shown="\"Start Task 1\", Default" w3118 {
              tunnel: w3109 -> [w3124 _]
              tunnel: [w3131 State_Type_Definitions,_for_0.26g_versions_and_later_3."True Stop" ("Enum")] -> w3112
              tunnel: w3113 -> [w3123 _]
              tunnel: w3117 -> [w3130 w3147]
              tunnel: [w3129 w3148] -> w3110
              tunnel: [State_Type_Definitions,_for_0.26g_versions_and_later_3."Idle" ("Enum") State_Type_Definitions,_for_0.26g_versions_and_later_3."Shutdown" ("Enum")] -> w3111
              frame "Start Task 1", Default {
                n1006 = case shown="True" w3124 {
                  tunnel: w3130 -> [w3134 w3141]
                  tunnel: [w3135 w3140] -> w3129
                  frame False {
                    n1007 = for {
                      tunnel: string[] ["RIGHT", "READ NAVX", "READ LINE SENSOR", ""] ("element") -> [w3136] mode=indexing
                      shift-right: [w3138] -> w3135
                      shift-left: w3134 -> [w3137]
                      n1008 = Enqueue Element(queue=w3137, element=w3136) -> (queue out=w3138:refnum<queue>)  [unwired: 2 in, 2 out]
                    }
                  }
                  frame True {
                    n1009 = for {
                      shift-right: [w3143] -> w3140
                      shift-left: w3141 -> [w3144]
                      tunnel: string[] ["STOP", "RESET ENCODERS", "RESET FLAGS", "RESET YAW", "BOX COLOUR", ""] -> [w3142] mode=indexing
                      n1010 = Enqueue Element(queue=w3144, element=w3142) -> (queue out=w3143:refnum<queue>)  [unwired: 2 in, 2 out]
                    }
                  }
                }
                n1011 = Or(x=w3124, y=w3123) -> (x .or. y?=w3122:bool)
                n1012 = Select(t=State_Type_Definitions,_for_0.26g_versions_and_later_3."True Stop" ("Enum"), s=w3123, f=State_Type_Definitions,_for_0.26g_versions_and_later_3."Task 9M: SCAN BOX 3" ("Enum")) -> (s? t:f=w3125:T18)
                n1013 = Select(t=w3125, s=w3122, f=State_Type_Definitions,_for_0.26g_versions_and_later_3."Task 9L: MOVE RIGHT" ("Enum")) -> (s? t:f=w3131:T18)
              }
              frame "Exit" {
                n1014 = for {
                  shift-right: [w3151] -> w3148
                  shift-left: w3147 -> [w3152]
                  tunnel: string[] ["STOP", "RESET ENCODERS", "RESET YAW", "ARDUINO MODE 0"] -> [w3150] mode=indexing
                  n1015 = Enqueue Element(queue=w3152, element=w3150) -> (queue out=w3151:refnum<queue>)  [unwired: 2 in, 2 out]
                }
              }
            }
          }
          frame "Task 9M: SCAN BOX 3" {
            # ">>> Motor control cluster >>>"
            # ">>> yStepper command>>>"
            # ">> Item Selection Bias >>"
            n1016 = Dequeue Element(queue=w3162, timeout in ms (-1)=w3161, error in (no error)=w3160) -> (element=w3166:T10)  [unwired: 3 out]
            n1017 = call "Box Colour FGV.vi"("Init/R/W State"=Box_Colour_FGV_States."Read") -> ("Colour to detect (output)"=w3156:T2)  [unwired: 9 in, 1 out]
            n1018 = Equal?(x=w3155, y=w3156) -> (x = y?=w3154:bool)
            n1019 = case shown="\"Start Task 1\", Default" w3166 {
              tunnel: w3153 -> [w3174 _]
              tunnel: [w3181 State_Type_Definitions,_for_0.26g_versions_and_later_3."True Stop" ("Enum")] -> w3164
              tunnel: w3159 -> [w3170 _]
              tunnel: w3163 -> [w3180 w3197]
              tunnel: [w3179 w3198] -> w3158
              tunnel: [State_Type_Definitions,_for_0.26g_versions_and_later_3."Idle" ("Enum") State_Type_Definitions,_for_0.26g_versions_and_later_3."Shutdown" ("Enum")] -> w3165
              tunnel: w3154 -> [w3172 _]
              frame "Start Task 1", Default {
                n1020 = case shown="True" w3174 {
                  tunnel: w3180 -> [w3184 w3191]
                  tunnel: [w3185 w3190] -> w3179
                  frame False {
                    n1021 = for {
                      tunnel: string[] ["", "", "", ""] ("element") -> [w3186] mode=indexing
                      shift-right: [w3188] -> w3185
                      shift-left: w3184 -> [w3187]
                      n1022 = Enqueue Element(queue=w3187, element=w3186) -> (queue out=w3188:refnum<queue>)  [unwired: 2 in, 2 out]
                    }
                  }
                  frame True {
                    n1023 = for {
                      shift-right: [w3193] -> w3190
                      shift-left: w3191 -> [w3194]
                      tunnel: string[] ["STOP", "RESET ENCODERS", "RESET FLAGS", "RESET YAW", "", ""] -> [w3192] mode=indexing
                      n1024 = Enqueue Element(queue=w3194, element=w3192) -> (queue out=w3193:refnum<queue>)  [unwired: 2 in, 2 out]
                    }
                  }
                }
                n1025 = Or(x=w3174, y=w3170) -> (x .or. y?=w3173:bool)
                n1026 = Or(x=w3172, y=w3170) -> (x .or. y?=w3171:bool)
                n1027 = Select(t=State_Type_Definitions,_for_0.26g_versions_and_later_3."True Stop" ("Enum"), s=w3171, f=State_Type_Definitions,_for_0.26g_versions_and_later_3."Task 9N: MOVE RIGHT" ("Enum")) -> (s? t:f=w3175:T18)
                n1028 = Select(t=w3175, s=w3173, f=State_Type_Definitions,_for_0.26g_versions_and_later_3."Task 9M: SCAN BOX 3" ("Enum")) -> (s? t:f=w3181:T18)
              }
              frame "Exit" {
                n1029 = for {
                  shift-right: [w3201] -> w3198
                  shift-left: w3197 -> [w3202]
                  tunnel: string[] ["STOP", "RESET ENCODERS", "RESET YAW", "ARDUINO MODE 0"] -> [w3200] mode=indexing
                  n1030 = Enqueue Element(queue=w3202, element=w3200) -> (queue out=w3201:refnum<queue>)  [unwired: 2 in, 2 out]
                }
              }
            }
          }
          frame "Task 9N: MOVE RIGHT" {
            # ">> Item Selection Bias >>"
            n1031 = Dequeue Element(queue=w3207, timeout in ms (-1)=w3206, error in (no error)=w3205) -> (element=w3212:T10)  [unwired: 3 out]
            n1032 = case shown="\"Start Task 1\", Default" w3212 {
              tunnel: w3203 -> [w3218 _]
              tunnel: [w3225 State_Type_Definitions,_for_0.26g_versions_and_later_3."True Stop" ("Enum")] -> w3210
              tunnel: w3204 -> [w3217 _]
              tunnel: w3208 -> [w3224 w3241]
              tunnel: [w3223 w3242] -> w3209
              tunnel: [State_Type_Definitions,_for_0.26g_versions_and_later_3."Idle" ("Enum") State_Type_Definitions,_for_0.26g_versions_and_later_3."Shutdown" ("Enum")] -> w3211
              frame "Start Task 1", Default {
                n1033 = case shown="True" w3218 {
                  tunnel: w3224 -> [w3228 w3235]
                  tunnel: [w3229 w3234] -> w3223
                  frame False {
                    n1034 = for {
                      tunnel: string[] ["READ LINE SENSOR", "READ NAVX", "RIGHT", "READ ENCODERS"] ("element") -> [w3230] mode=indexing
                      shift-right: [w3232] -> w3229
                      shift-left: w3228 -> [w3231]
                      n1035 = Enqueue Element(queue=w3231, element=w3230) -> (queue out=w3232:refnum<queue>)  [unwired: 2 in, 2 out]
                    }
                  }
                  frame True {
                    n1036 = for {
                      shift-right: [w3237] -> w3234
                      shift-left: w3235 -> [w3238]
                      tunnel: string[] ["STOP", "RESET ENCODERS", "RESET YAW", "RESET FLAGS", "BOX COLOUR", ""] -> [w3236] mode=indexing
                      n1037 = Enqueue Element(queue=w3238, element=w3236) -> (queue out=w3237:refnum<queue>)  [unwired: 2 in, 2 out]
                    }
                  }
                }
                n1038 = Or(x=w3218, y=w3217) -> (x .or. y?=w3216:bool)
                n1039 = Select(t=State_Type_Definitions,_for_0.26g_versions_and_later_3."True Stop" ("Enum"), s=w3217, f=State_Type_Definitions,_for_0.26g_versions_and_later_3."Task 9O: SCAN BOX 4" ("Enum")) -> (s? t:f=w3219:T18)
                n1040 = Select(t=w3219, s=w3216, f=State_Type_Definitions,_for_0.26g_versions_and_later_3."Task 9N: MOVE RIGHT" ("Enum")) -> (s? t:f=w3225:T18)
              }
              frame "Exit" {
                n1041 = for {
                  shift-right: [w3245] -> w3242
                  shift-left: w3241 -> [w3246]
                  tunnel: string[] ["STOP", "RESET ENCODERS", "RESET YAW", "ARDUINO MODE 0"] -> [w3244] mode=indexing
                  n1042 = Enqueue Element(queue=w3246, element=w3244) -> (queue out=w3245:refnum<queue>)  [unwired: 2 in, 2 out]
                }
              }
            }
          }
          frame "Task 9O: SCAN BOX 4" {
            # ">>> Motor control cluster >>>"
            # ">>> yStepper command>>>"
            # ">> Item Selection Bias >>"
            n1043 = Dequeue Element(queue=w3257, timeout in ms (-1)=w3256, error in (no error)=w3255) -> (element=w3261:T10)  [unwired: 3 out]
            n1044 = call "Box Colour FGV.vi"("Init/R/W State"=Box_Colour_FGV_States."Read") -> ("Colour to detect (output)"=w3259:T2)  [unwired: 9 in, 1 out]
            n1045 = Equal?(x=w3249, y=w3259) -> (x = y?=w3258:bool)
            n1046 = case shown="\"Start Task 1\", Default" w3261 {
              tunnel: w3247 -> [w3268 _]
              tunnel: [w3275 State_Type_Definitions,_for_0.26g_versions_and_later_3."True Stop" ("Enum")] -> w3251
              tunnel: w3254 -> [w3264 _]
              tunnel: w3248 -> [w3274 w3291]
              tunnel: [w3273 w3292] -> w3252
              tunnel: [State_Type_Definitions,_for_0.26g_versions_and_later_3."Idle" ("Enum") State_Type_Definitions,_for_0.26g_versions_and_later_3."Shutdown" ("Enum")] -> w3250
              tunnel: w3258 -> [w3266 _]
              frame "Start Task 1", Default {
                n1047 = case shown="True" w3268 {
                  tunnel: w3274 -> [w3278 w3285]
                  tunnel: [w3279 w3284] -> w3273
                  frame False {
                    n1048 = for {
                      tunnel: string[] ["", "", "", ""] ("element") -> [w3280] mode=indexing
                      shift-right: [w3282] -> w3279
                      shift-left: w3278 -> [w3281]
                      n1049 = Enqueue Element(queue=w3281, element=w3280) -> (queue out=w3282:refnum<queue>)  [unwired: 2 in, 2 out]
                    }
                  }
                  frame True {
                    n1050 = for {
                      shift-right: [w3287] -> w3284
                      shift-left: w3285 -> [w3288]
                      tunnel: string[] ["STOP", "RESET ENCODERS", "RESET FLAGS", "RESET YAW", "", ""] -> [w3286] mode=indexing
                      n1051 = Enqueue Element(queue=w3288, element=w3286) -> (queue out=w3287:refnum<queue>)  [unwired: 2 in, 2 out]
                    }
                  }
                }
                n1052 = Or(x=w3268, y=w3264) -> (x .or. y?=w3267:bool)
                n1053 = Or(x=w3266, y=w3264) -> (x .or. y?=w3265:bool)
                n1054 = Select(t=State_Type_Definitions,_for_0.26g_versions_and_later_3."True Stop" ("Enum"), s=w3265, f=State_Type_Definitions,_for_0.26g_versions_and_later_3."True Stop" ("Enum")) -> (s? t:f=w3269:T18)
                n1055 = Select(t=w3269, s=w3267, f=State_Type_Definitions,_for_0.26g_versions_and_later_3."Task 9O: SCAN BOX 4" ("Enum")) -> (s? t:f=w3275:T18)
              }
              frame "Exit" {
                n1056 = for {
                  shift-right: [w3295] -> w3292
                  shift-left: w3291 -> [w3296]
                  tunnel: string[] ["STOP", "RESET ENCODERS", "RESET YAW", "ARDUINO MODE 0"] -> [w3294] mode=indexing
                  n1057 = Enqueue Element(queue=w3296, element=w3294) -> (queue out=w3295:refnum<queue>)  [unwired: 2 in, 2 out]
                }
              }
            }
          }
        }
        "Object Detection" <- w320
        "Ultrasonic sensors" <- w343
        "Encoder values" <- w332
        "Stepper position values" <- w316
        "NAVX Values" <- w314
        "IR Sensors" <- w306
        "Line sensors" <- w301
        "Time cluster" <- w312
        "Box Colour Detection" <- w294
      }
    }
    "Object recognition mode" <- w218
    "Front Ultrasonic obstruct" <- w215
    "Front IR obstruct" <- w214
    "Table IR obstruct" <- w213
    "Same colour?" <- w208
    n1058 = local write "Green LED"(w228) -> ()
  }
  n1059 = while {
    tunnel: w47 -> [w4215]
    tunnel: w46 -> [w4212]
    stop <- w4209 stop-if-true
    # "Status Loop for Action Queues"
    n1060 = Get Queue Status(queue=w4215, return elements? (F)=TRUE) -> (error out=w4211:errorcluster, # elements in queue=→"Action Queue Items":i32, elements=→"Action Queues items":string[])  [unwired: 1 in, 5 out]
    n1061 = Get Queue Status(queue=w4212, return elements? (F)=TRUE) -> (# pending remove=→"State Logic Queue Items":i32, error out=w4210:errorcluster, elements=→"elements":T10[])  [unwired: 1 in, 5 out]
    n1062 = Merge Errors(w4211, w4210) -> (w4209:errorcluster)
    n1063 = Wait (ms)(milliseconds to wait=u32 500) -> ()  [unwired: 1 out]
  }
  n1064 = call <vilib>:"DIO Close.vi"("error in (no error)"=w23, "DIO Info In"=w26) -> ()  [unwired: 9 in, 1 out]
  n1065 = call <vilib>:"DIO Close.vi"("error in (no error)"=w33, "DIO Info In"=w35) -> ()  [unwired: 9 in, 1 out]
  n1066 = call <vilib>:"NavX Close.vi"("error in (no error)"=w10, "NavX Info In"=w9) -> ()  [unwired: 9 in, 1 out]
  n1067 = call <vilib>:"DIO Close.vi"("error in (no error)"=w28, "DIO Info In"=w30) -> ()  [unwired: 9 in, 1 out]
  n1068 = call <vilib>:"DIO Close.vi"("error in (no error)"=w17, "DIO Info In"=w18) -> ()  [unwired: 9 in, 1 out]
  n1069 = call <vilib>:"DIO Close.vi"("error in (no error)"=w12, "DIO Info In"=w13) -> ()  [unwired: 9 in, 1 out]
  n1070 = Merge Errors "Merge Errors"(w63, w62) -> (w45:errorcluster)
  n1071 = Merge Errors(w49, w45) -> (w44:errorcluster)
  n1072 = Destroy User Event(user event=w67, error in=w44) -> ()  [unwired: 1 out]
  n1073 = Release Queue(queue=w40, error in (no error)=w44) -> (error out=→"Queue Errors":errorcluster)  [unwired: 1 in, 2 out]
  n1074 = Release Queue(queue=w57, error in (no error)=w44) -> ()  [unwired: 1 in, 3 out]
  n1075 = Destroy User Event(user event=w66, error in=w44) -> ()  [unwired: 1 out]
  n1076 = Unregister For Events(event registration refnum=w58, error in=w44) -> ()  [unwired: 1 out]
